vi "FIB MAIN.vi"() -> ()   [LabVIEW 2018]
uses:
  <vilib>/userdefined/High Color/IMAQdx.ctl
  STAGE POSITION.ctl
  Original FIB Source/CENTER STIGMATOR.ctl
  FIB EVENTS.ctl
  PI APERTURE POSITION.ctl
  APERTURE POSITION.ctl
  FIB CAMERA EVENTS.ctl
  <vilib>/vision/driver/IMAQdx.llb/IMAQdx Buffer Number Mode.ctl
  <vilib>/vision/driver/IMAQdx.llb/IMAQdx Camera Control Mode.ctl
  <vilib>/Instr/_visa.llb/VISA Flush IO Buffer Mask.ctl
  <vilib>/Utility/error.llb/whitespace.ctl
  Mikrodaq/HYMOD MAIA/ddd.ctl
  PI STAGE MAXIMUMS.ctl
  FIB STAGE EVENTS.ctl
  <vilib>/Instr/_visa.llb/VISA Configure Serial Port (Instr).vi
  <vilib>/vision/driver/NI_Vision_Acquisition_Software.lvlib
  <resource>/objmgr/imaqdx.rc
  <vilib>/vision/NI_Vision_Development_Module.lvlib
  <vilib>/Utility/Variable/NI_VariableUtilities.lvlib
panel:
  out "elements":T1[](array[typedef])
  out "PREVIOUS GUN SETTINGS":T2 {"ION CURRENT" min=0 max=3e-05 step=1e-07; "SUPPRESSOR" min=0 max=30000 step=250; "EXTRACTOR" min=0 max=30000 step=250; "BEAM ENERGY" min=0 max=30000 step=1000}
  out "size(s) 5":i32
  in  "ENABLE ORSAY":bool=TRUE
  in  "ENABLE CAMERA":bool
  out "size(s) 4":i32
  in  "Tab Control 4":enum32{"COMMANDS", "HV RAMPS"}(tab)
  in  "1V ENERGY RAMP":bool
  out "TEST OUTPUT":string
  in  "TEST COMMAND":bool
  in  "TEST COMMAND":string
  out "SERIAL \nRESPONSE":string[](array[string])
  out "WARNING":string
  out "PROCESS":string
  out "PROCESSES":string[](array[string])
  out "BEAM RAMP":dbl[unit][](graph)
  out "EXTRACTOR RAMP":dbl[unit][](graph)
  out "SUPPRESSOR RAMP":dbl[unit][](graph)
  in  "Tab Control 3":T3(tab)
  in  "E&B":T4 {"ELECTRIC FIELD" min=0 max=20 step=0.1 scale=0.0..2.0; "M-FINE" min=0 max=20000 step=100 scale=-0.08..0.08; "M-COARSE" min=0 max=20 step=0.1 scale=0.0..2.0}
  in  "WIEN":bool
  out "CURRENT":dbl[unit] format="%_4g"
  out "VOLTAGE":dbl[unit] format="%_4g"
  out "BEAM VOLTAGE":dbl[unit](graph)
  out "BEAM CURRENT":dbl[unit](graph)
  out "VOLTAGE":dbl[unit] format="%_4g"
  out "CURRENT":dbl[unit] format="%_4g"
  out "EXTRACTOR":dbl[unit](graph)
  out "EXTRACTOR  CURRENT":dbl[unit](graph)
  out "VOLTAGE":dbl[unit] format="%_4g"
  out "CURRENT":dbl[unit] format="%_4g"
  out "SUPPRESSOR VOLTAGE":dbl[unit](graph)
  out "SUPPRESSOR CURRENT":dbl[unit](graph)
  out "CONDENSOR VOLTAGE":dbl[unit](graph)
  out "CONDENSOR CURRENT":dbl[unit](graph)
  out "OBJECTIVE VOLTAGE":dbl[unit](graph)
  out "OBJECTIVE CURRENT":dbl[unit](graph)
  out "HV SUPPLY FEEDBACK 13":dbl[unit](graph)
  out "HV SUPPLY FEEDBACK 12":dbl[unit](graph)
  out "HEAT POWER":cluster{i32[], dbl[unit][]}(graph)
  in  "IGAIN":dbl=0.00039 format="%_3p"
  in  "IOFFSET":dbl format="%_4g"
  in  "VOFFSET":dbl format="%_4g"
  out "CURRENT":dbl[unit] format="%_4g"
  out "VOLTAGE":dbl[unit] format="%_4g"
  in  "VGAIN":dbl=0.00071 format="%_3p"
  in  "OFFSET":dbl
  in  "RPONT":dbl[unit]
  in  "RMES":dbl[unit]
  out "TIMER":u32
  out "size(s)":i32
  out "SUPPRESSOR RAMP":dbl[unit][](array[numeric])
  out "EXTRACTOR RAMP":dbl[unit][](array[numeric])
  out "BEAM RAMP":dbl[unit][](array[numeric])
  in  "MEASURE HV":bool
  out "SERIAL \nRESPONSE 2":string[](array[string])
  out "VISA ERROR":errorcluster
  out "BEAM CURRENT (FC2)":dbl[unit] format="%_4g"
  out "BEAM CURRENT (FC1)":dbl[unit] format="%_4g"
  in  "APERTURE (MASS)":u16(ring)=3 items=["10 um", "20 um", "50 um", "50 um", "100 um", "200 um", "400 um"]
  in  "BRIGHT,CONT,GAMMA":cluster{"B":dbl, "C":dbl, "G":dbl}={"B"=250.0, "C"=67.0, "G"=1.6000000000000005} {"G" format="%_4g"; "C" format="%_4g"; "B" format="%_4g"}
  in  "REFLECTIVITY":bool
  in  "ROTATE VIEW":bool
  in  "ANGLE":sgl format="%.2f"
  in  "IMAGE SYMMETRY":u32(ring)=2 items=["Horizontal", "Vertical", "CENTRAL", "1st Diagonal", "2nd Diagonal"]
  in  "SYMMETRY":bool
  out "FIB CAMERA ERROR":errorcluster
  out "FIB SAMPLE CAMERA":T5="CSIRO-SAMPLE" caption="Session Out"
  out "IMAGE YCENTRE":dbl
  out "IMAGE XCENTRE":dbl
  out "ActualPeakBandwidth":dbl=1000.0
  out "IMAGE YPIXELS":u32=1024
  out "IMAGE XPIXELS":u32=1360
  in  "START SCANNING":bool
  in  "STOP":bool
  out "INTERLOCK STATE":bool
  in  "BEAM ON":bool=TRUE
  in  "BLANKING CONTROL":u16(ring) items=["LOCAL ", "SOURCE", "EXTERNAL"]
  in  "FIB SETUP FILE":path=path "C:/Users/jamie/Desktop/test.tdms"
  in  "SAVE SETUP":bool
  in  "READ & APPLY SETUP":bool
  in  "OBJECT APERTURE":u16(ring)=3 items=["10 um", "20 um", "50 um", "50 um", "100 um", "200 um", "400 um"]
  in  "USER":string="jslaird"
  in  "COMMENT":string
  in  "NAME":string
  out "gamme":bool
  out "Image":T6(plugin-control)
  in  "Tab Control":T7(tab)
  in  "RESET":bool
  in  "INTERLOCK HV":bool
  out "HIGH ENERGY":bool
  in  "SETTINGS DELAY":dbl[unit]=0.2
  in  "dV ENERGY":dbl[unit]=250.0
  in  "dV SUPPRESS":dbl[unit]=50.0
  in  "SHUTDOWN":bool
  in  "FILAMENT":bool
  out "HIGH VOLTAGE SUPPLIES":cluster{dbl[unit], dbl[unit], dbl[unit]}(knob)={0.0, 103.78830891166923, 181.50345045415557} scale format="%#_6p"
  in  "ION GUN":bool
  in  "FILAMENT HEATING":dbl[unit](slide) min=0.0 max=5.0 step=0.1 scale=0.0..5.000000000000001
  in  "ION GUN SETTINGS":T2 {"ION CURRENT" min=0 max=3e-05 step=1e-07; "SUPPRESSOR" min=0 max=30000 step=250; "EXTRACTOR" min=0 max=30000 step=250; "BEAM ENERGY" min=0 max=30000 step=250}
  in  "dV EXTRACTOR":dbl[unit]=50.0
  in  "MOVE 2 POSITION":T8 {"Z" format="%_4g"; "Y" format="%_4g"; "X" format="%_4g"}
  out "POSITION":T8 {"Z" format="%_4g"; "Y" format="%_4g"; "X" format="%_4g"}
  in  "EXPOSURE":dbl(slide)=106.26827541712952 min=1.0 max=2500.0 step=10.0 scale=5.0..1000.0 scale format="%#_3f"
  out "FIB CAMERA":T6(plugin-control)
  out "IP ADDRESS":string="192.168.1.10"
  in  "CONFIGS":u16(ring) items=["MANUAL", "BEAM FOCUS", "SAMPLE VIEWING"]
  in  "GAIN METHOD":u16(ring)=2 items=["OFF", "ONCE", "CONTINOUS"]
  in  "GAIN":sgl=1.0 min=0 max=31 step=1
  out "CENTRE CAMERA FOV":T9={"Numeric Control"=677, "Numeric Control"=510}
  in  "Tab Control 2":T10(tab)
  in  "STORE OBJECT":bool
  in  "WOBBLER SETTINBGS FOR OBJECT ALIGNMENT":T11={"WOBBLER AMPLITUDE"={0.0, 33.333523, 47.735184}, "WOBBLE"=1} {"WOBBLE" items=["ENERGY", "CONDENSOR", "OBJECTIVE"]; "WOBBLER AMPLITUDE" scale=0.0..100.0}
  in  "OBJ APERTURE ALIGNMENT":T12={"DOWN"=FALSE, "UP"=FALSE, "STEP SIZE"=1, "LEFT"=FALSE, "RIGHT"=FALSE} {"STEP SIZE" items=["1 um", "5 um", "20 um", "50 um", "100 um", "250 um", "500 um", "1000 um"]}
  in  "TURN ON WOBBLER":bool
  out "OBJECT POSITION":T13 {"Yo" format="%.3f"; "Xo" min=0.0 max=12.5 step=0.1 format="%.3f"}
  in  "SET OBJECT":T13 {"Yo" min=0.0 max=10.0 step=0.1 format="%.3f"; "Xo" min=0.0 max=12.5 step=0.1 format="%.3f"}
  in  "OBJECT POSITIONS":T14(array[cluster])=[{"POSITION"={"Xm"=0.5, "Ym"=0.1114}}, {"POSITION"={"Xm"=0.0, "Ym"=0.0}}, {"POSITION"={"Xm"=11.3603, "Ym"=0.0}}, {"POSITION"={"Xm"=9.6127, "Ym"=0.0}}, {"POSITION"={"Xm"=7.8602, "Ym"=0.0}}, {"POSITION"={"Xm"=6.1203, "Ym"=0.0}}, {"POSITION"={"Xm"=4.37, "Ym"=0.0}}, {"POSITION"={"Xm"=0.0, "Ym"=0.0}}, {"POSITION"={"Xm"=0.0, "Ym"=0.0}}] {"POSITION"."Ym" format="%.3f"; "POSITION"."Xm" format="%.3f"}
  in  "MASS APERTURE ALIGNMENT":T12={"DOWN"=FALSE, "UP"=FALSE, "STEP SIZE"=1, "LEFT"=FALSE, "RIGHT"=FALSE} {"STEP SIZE" items=["1 um", "5 um", "20 um", "50 um", "100 um", "250 um", "500 um", "1000 um"]}
  in  "STORE APERTURE":bool
  out "APERTURE POSITION":cluster{"Xm":dbl, "Ym":dbl} {"Ym" format="%.3f"; "Xm" format="%.3f"}
  in  "SET APERTURE":T15 {"Ym" min=-0.5 max=0.5 step=0.01 format="%.3f"; "Xm" min=-25.0 max=25.0 step=0.1 format="%.3f"}
  in  "APERTURE POSITIONS":T14(array[cluster])=[{"POSITION"={"Xm"=0.0, "Ym"=0.0}}, {"POSITION"={"Xm"=0.0, "Ym"=0.0}}, {"POSITION"={"Xm"=0.0, "Ym"=0.0}}, {"POSITION"={"Xm"=0.0, "Ym"=0.0}}, {"POSITION"={"Xm"=1.0, "Ym"=0.0}}, {"POSITION"={"Xm"=0.0, "Ym"=0.0}}, {"POSITION"={"Xm"=0.0, "Ym"=0.0}}] {"POSITION"."Ym" format="%.3f"; "POSITION"."Xm" format="%.3f"}
  in  "STIGMATOR":T16 {"STIG ALIGN"."-Y" min=-100 max=100 step=0.1 scale=-100.0..100.0; "STIG ALIGN"."+Y" min=-100 max=100 step=0.1 scale=-100.0..100.0; "STIG ALIGN"."-X" min=-100 max=100 step=0.1 scale=-100.0..100.0; "STIG ALIGN"."+X" min=-100 max=100 step=0.1 scale=-100.0..100.0; "THETA" format="%_3g"; "OFFY" format="%_3g"; "OFFX" format="%_3g"; "STIG Y" format="%_3g"; "STIG X" format="%_3g"}
  in  "STIGMATOR X & Y":cluster{"X":sgl, "Y":sgl} {"Y" min=0 max=20000 step=100 scale=0.0..1000.0; "X" min=0 max=20 step=0.1 scale=0.0..20.0}
  out "OBJECTIVE":sgl[unit] format="%_4g"
  out "CONDENSOR":sgl[unit] format="%_4g"
  in  "OBJECTIVE":cluster{"COARSE":sgl[unit], "FINE":sgl[unit]} {"FINE" min=0 max=20000 step=100 scale=0.0..1000.0; "COARSE" min=0 max=20000 step=100}
  in  "CONDENSOR":cluster{"COARSE":sgl[unit], "FINE":sgl[unit]} {"FINE" min=0 max=20000 step=100 scale=1.0..1000.0; "COARSE" min=0 max=20000 step=100}
  in  "SCAN CENTRE ON STAGE":T17 {"Zs" format="%_2g"; "Xs" format="%_2g"; "Ys" format="%_2g"}
  in  "STAGE POSITION":T17 {"Zs" format="%_2g"; "Xs" format="%_2g"; "Ys" format="%_2g"}
  in  "SCANNING CLUSTER":T18 {"MAGNIFICATION" scale=-180.0..180.0; "Y-OFFSET" min=0 max=3e-05 step=1e-07; "X-OFFSET" min=0 max=3e-05 step=1e-07; "SCANNING TYPE" items=["EXTERNAL", "ION MILLING"]}
  in  "EXTERNAL SCANNING ROI":T19={"X-AMPLITUDE"=1e-07, "dX"=0.0, "Y-AMPLITUDE"=1e-07, "dY"=0.0} {"Y-AMPLITUDE" min=1e-07 max=0.0005 step=9.999999999999999e-06; "X-AMPLITUDE" min=1e-07 max=0.0005 step=9.999999999999999e-06}
  out "CHAMBER VACUUM":cluster{dbl[unit], dbl[unit]}(knob)={2.179544466940017e-05, 0.00030039245125477424} scale format="%#_2e"
  in  "COLUMN THRESHOLD":dbl[unit]=6.666118421052631e-05
  out "VACUUM STATE":bool
  out "COLUMN VACUUM":dbl[unit](graph)
  out "COLUMN VACUUM":cluster{dbl[unit], dbl[unit]}(knob)={8.118323356328827e-09, 0.00010317996118558537} scale format="%#_1e"
  out "150V GOOD":bool
  in  "CHAMBER THRESHOLD":dbl[unit]
  in  "GATE VALVE":bool=TRUE
  in  "TERMINATION":bool=TRUE
  in  "TERMINATION CHAR":u16(ring)=1 items=["NONE", "CR", "LF", "CR+LF"]
  out "APPEND":string
  out "ORSAY CONNECTED":bool
  in  "STARTUP":T1[](array[typedef])=[enum."OPEN SERIAL CONN TO ORSAY", enum."INITIALISE ORSAY", enum."TURN OFF WOBBLER", enum."VACUUM ", enum."CHECK 150V", enum."BLANKING TOGGLE"]
  out "ORSAY":refnum<visa-resource-name>
  # "EXTRACTOR"
  # "CONDENSOR"
  # "OBJECT\nAPERTURES"
  # "OBJECTIVE"
  # "FILAMENT SHOULD BE ON PRIOR TO GUN !"
  # "E"
  # "C"
  # "O"
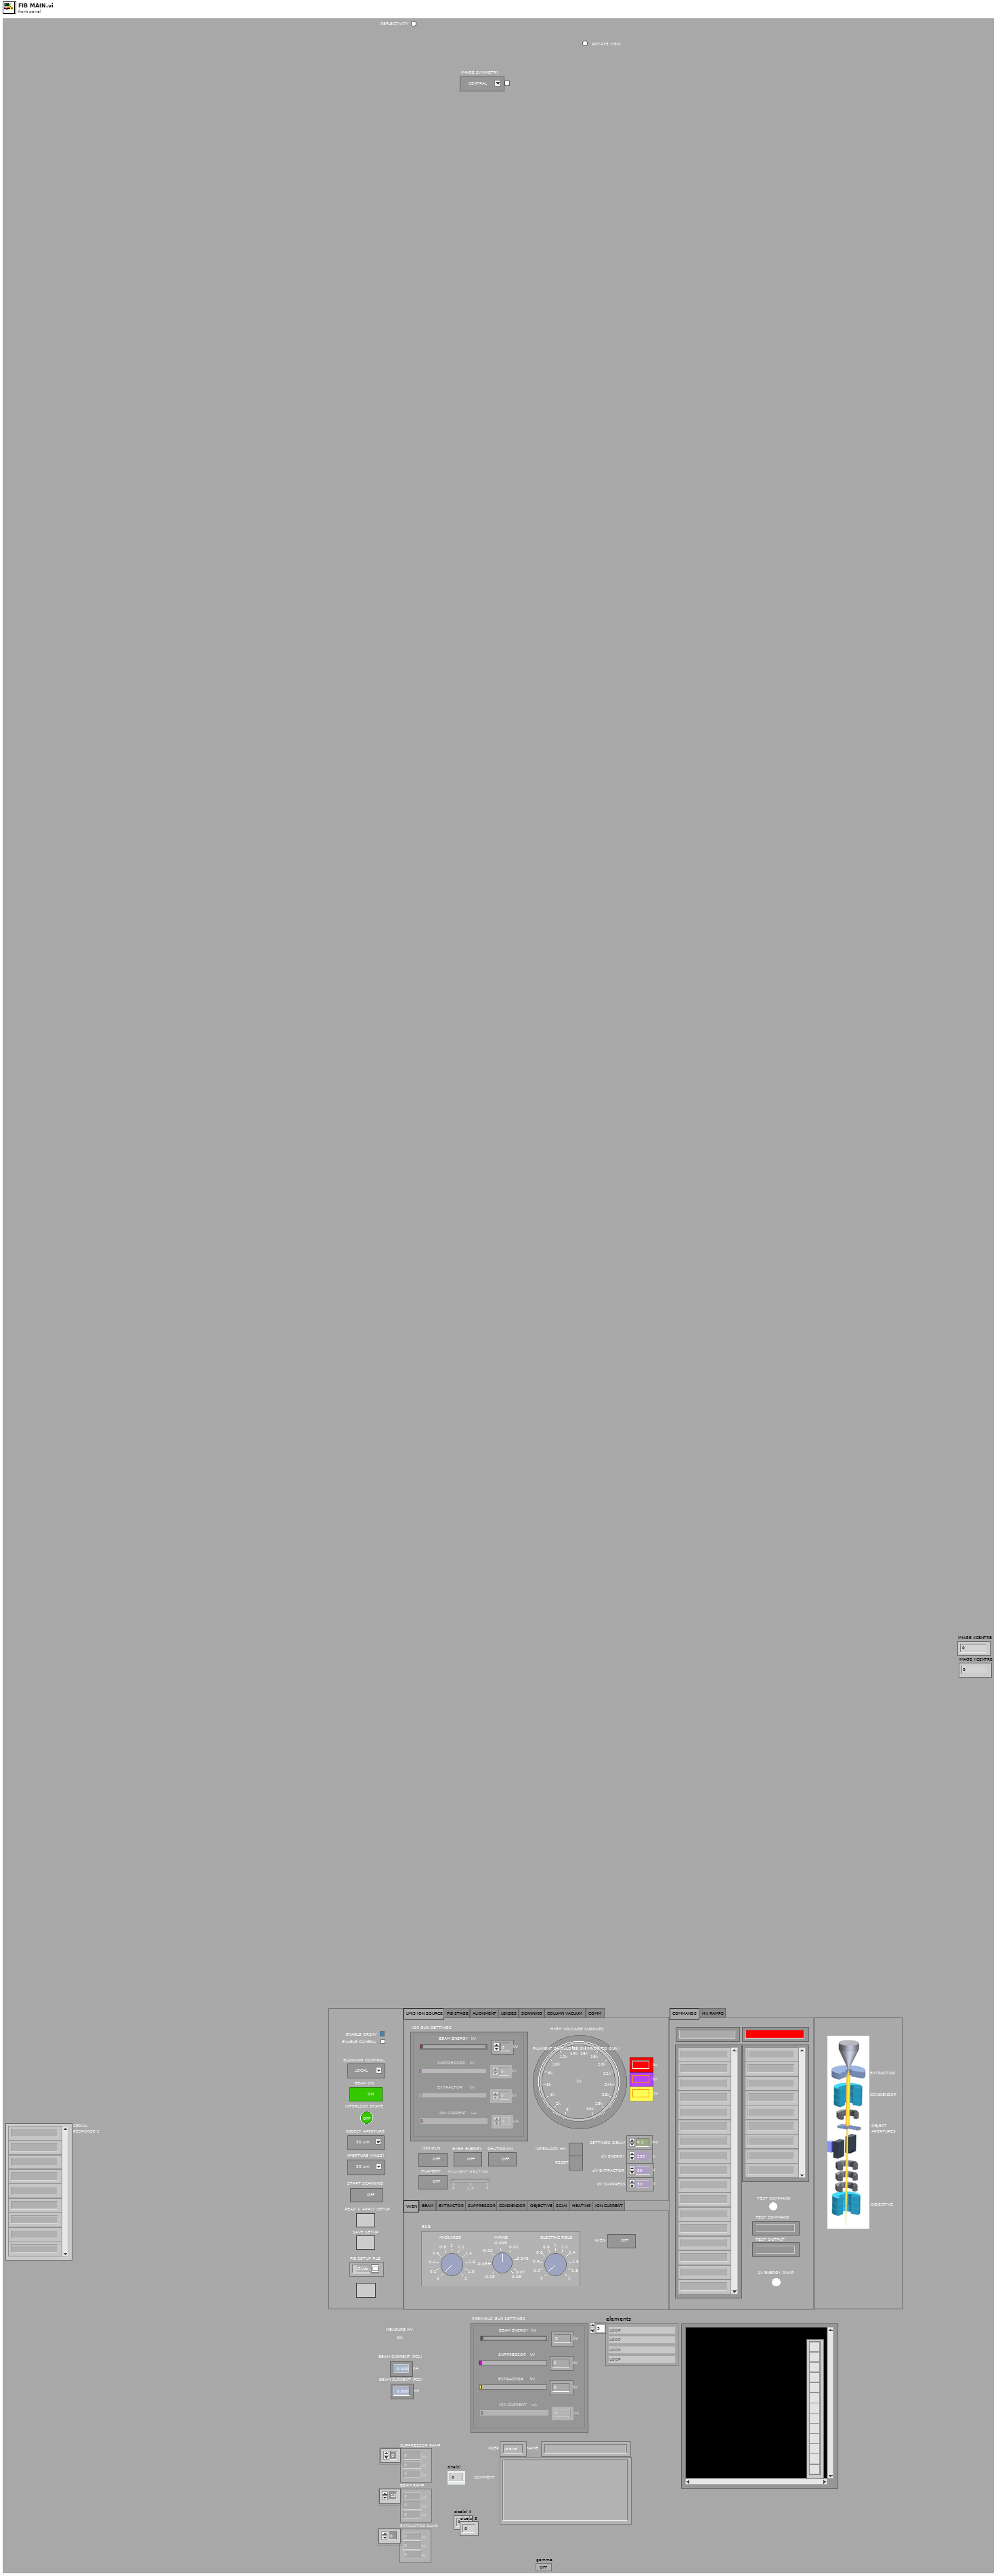
[diagram p1: front panel]
types:
  T1 = typedef "FIB EVENTS.ctl" = enum16{"LOOP", "OPEN SERIAL CONN TO ORSAY", "INITIALISE ORSAY", "READ SETTINGS", "SAVE SETTINGS", "OBJECTIVE LENS", "CONDENSOR LENS", "BLANKING TOGGLE", "TURN ON HEATER", "TURN OFF WOBBLER", "MEASURE HEATER OUTPUT", "TOGGLE GATE VALVE", "SCANNING CONTROLS", "TURN ON BEAM HV", "ENERGY RAMP CYCLE", "TURN ON SUPPRESSOR", "TURN ON EXTRACTOR", "TURN ON WIEN FILTER", "SET ENERGY RANGE", "MEASURE HV SUPPLY VOLTAGES", "SHUTDOWN ION SOURCE", "RESET TYPE II", "PROBE CURRENT FC#1", "PROBE CURRENT FC#2", "VACUUM ", "CHECK 150V", "INITIALISE PI MOTORS", "SET STIGMATOR", "SET WOBBLER FOR OBJECT", "SHIFT OBJECT APERTURE", "STORE OBJECT POSITION", "STORE APERTURE POSITION", "SHIFT MASS APERTURE", "DEFINE NEW APERTURE", "MOVE TO OBJECT", "MOVE TO APERTURE", "STOP SYSTEM", "TEST COMMANDS"}
  T2 = cluster{"BEAM ENERGY":sgl[unit], "SUPPRESSOR":sgl[unit], "EXTRACTOR":sgl[unit], "ION CURRENT":sgl[unit]}
  T3 = enum32{"WIEN", "BEAM", "EXTRACTOR", "SUPPRESSOR", "CONDENSOR", "OBJECTIVE", "SCAN", "HEATING", "ION CURRENT"}
  T4 = cluster{"M-COARSE":sgl, "M-FINE":sgl, "ELECTRIC FIELD":sgl}
  T5 = typedef "IMAQdx.ctl" = refnum<k21>
  T6 = typedef "IMAQ Image.ctl" = refnum<image>
  T7 = enum32{"LMIS ION SOURCE", "FIB STAGE", "ALIGNMENT", "LENSES", "SCANNING", "COLUMN VACUUM", "COMM"}
  T8 = typedef "STAGE POSITION.ctl" = cluster{"X":dbl[unit], "Y":dbl[unit], "Z":dbl[unit]}
  T9 = cluster{"Numeric Control":i32, "Numeric Control":i32}
  T10 = enum32{"OBJECTS", " APERTURES", "CENTRE STIGMATOR"}
  T11 = cluster{"WOBBLER AMPLITUDE":cluster{sgl, sgl, sgl}, "WOBBLE":u16}
  T12 = cluster{"DOWN":bool, "UP":bool, "STEP SIZE":u16, "LEFT":bool, "RIGHT":bool}
  T13 = typedef "PI APERTURE POSITION.ctl" = cluster{"Xo":dbl, "Yo":dbl}
  T14 = cluster{"POSITION":cluster{"Xm":dbl, "Ym":dbl}}[]
  T15 = typedef "APERTURE POSITION.ctl" = cluster{"Xm":dbl, "Ym":dbl}
  T16 = typedef "CENTER STIGMATOR.ctl" = cluster{"STIG ALIGN":cluster{"+X":sgl, "-X":sgl, "+Y":sgl, "-Y":sgl}, "STIG X":dbl, "OFFX":dbl, "STIG Y":dbl, "OFFY":dbl, "THETA":dbl}
  T17 = cluster{"Xs":dbl[unit], "Ys":dbl[unit], "Zs":dbl[unit]}
  T18 = cluster{"SCANNING TYPE":u16, "X-OFFSET":sgl[unit], "Y-OFFSET":sgl[unit], "ROTATION":dbl[unit], "MAGNIFICATION":dbl}
  T19 = cluster{"X-AMPLITUDE":dbl[unit], "dX":dbl[unit], "Y-AMPLITUDE":dbl[unit], "dY":dbl[unit]}
  T20 = typedef "FIB CAMERA EVENTS.ctl" = enum16{"INIT VIDEO", "CAMERA GAIN", "CAMERA EXPOSURE", "LOOP"}
  T21 = enum8{"Enabled", "Disabled", "Disabled and Grayed Out"}
  T22 = cluster{"BEAM ENERGY":sgl[unit], "EXTRACTOR":sgl[unit], "SUPPRESSOR":sgl[unit], "ION CURRENT":sgl[unit]}
  T23 = typedef "FIB STAGE EVENTS.ctl" = enum16{"LOOP", "INIT STAGE CONTROLLER", "SEND COMMAND TO CONTROLLER", "HOME X", "HOME Y", "HOME Z", "ABORT ALL AXES", "GOTO MARKER", "ZERO XYZ", "READ XYZ POSITIONS", "GOTO XYZ POSITION", "STOP", "JOG XYZ", "WAIT FOR MOVE COMPLETE"}
  T24 = cluster{"BEAM":dbl[unit], "SUPPRESSOR":dbl[unit], "EXTRACTOR":dbl[unit]}
  T25 = typedef "ddd.ctl" = string[]
  T26 = enum16{"open", "open or create", "create or replace", "create", "open (read-only)"}
  T27 = typedef "VISA Flush IO Buffer Mask.ctl" = u16
  T28 = cluster{dbl[unit], "CHAMBER THRESHOLD":dbl[unit]}
  T29 = typedef "whitespace.ctl" = u16
  T30 = typedef "PI STAGE MAXIMUMS.ctl" = cluster{"Xo MAX":dbl, "Xm MAX":dbl, "Yo MAX":dbl, "Ym MAX":dbl}
  T31 = cluster{"Xo MIN":dbl, "Xm MIN":dbl, "Yo MIN":dbl, "Ym MIN":dbl}
  T32 = typedef "NI_Vision_Acquisition_Software.lvlib/IMAQdx Buffer Number Mode.ctl" = enum32{"Next", "Last", "Buffer Number", "Every", "Last New"}
  T33 = typedef "NI_Vision_Acquisition_Software.lvlib/IMAQdx Camera Control Mode.ctl" = enum32{"Controller", "Listener"}
  T34 = typedef "Image Type" = u32
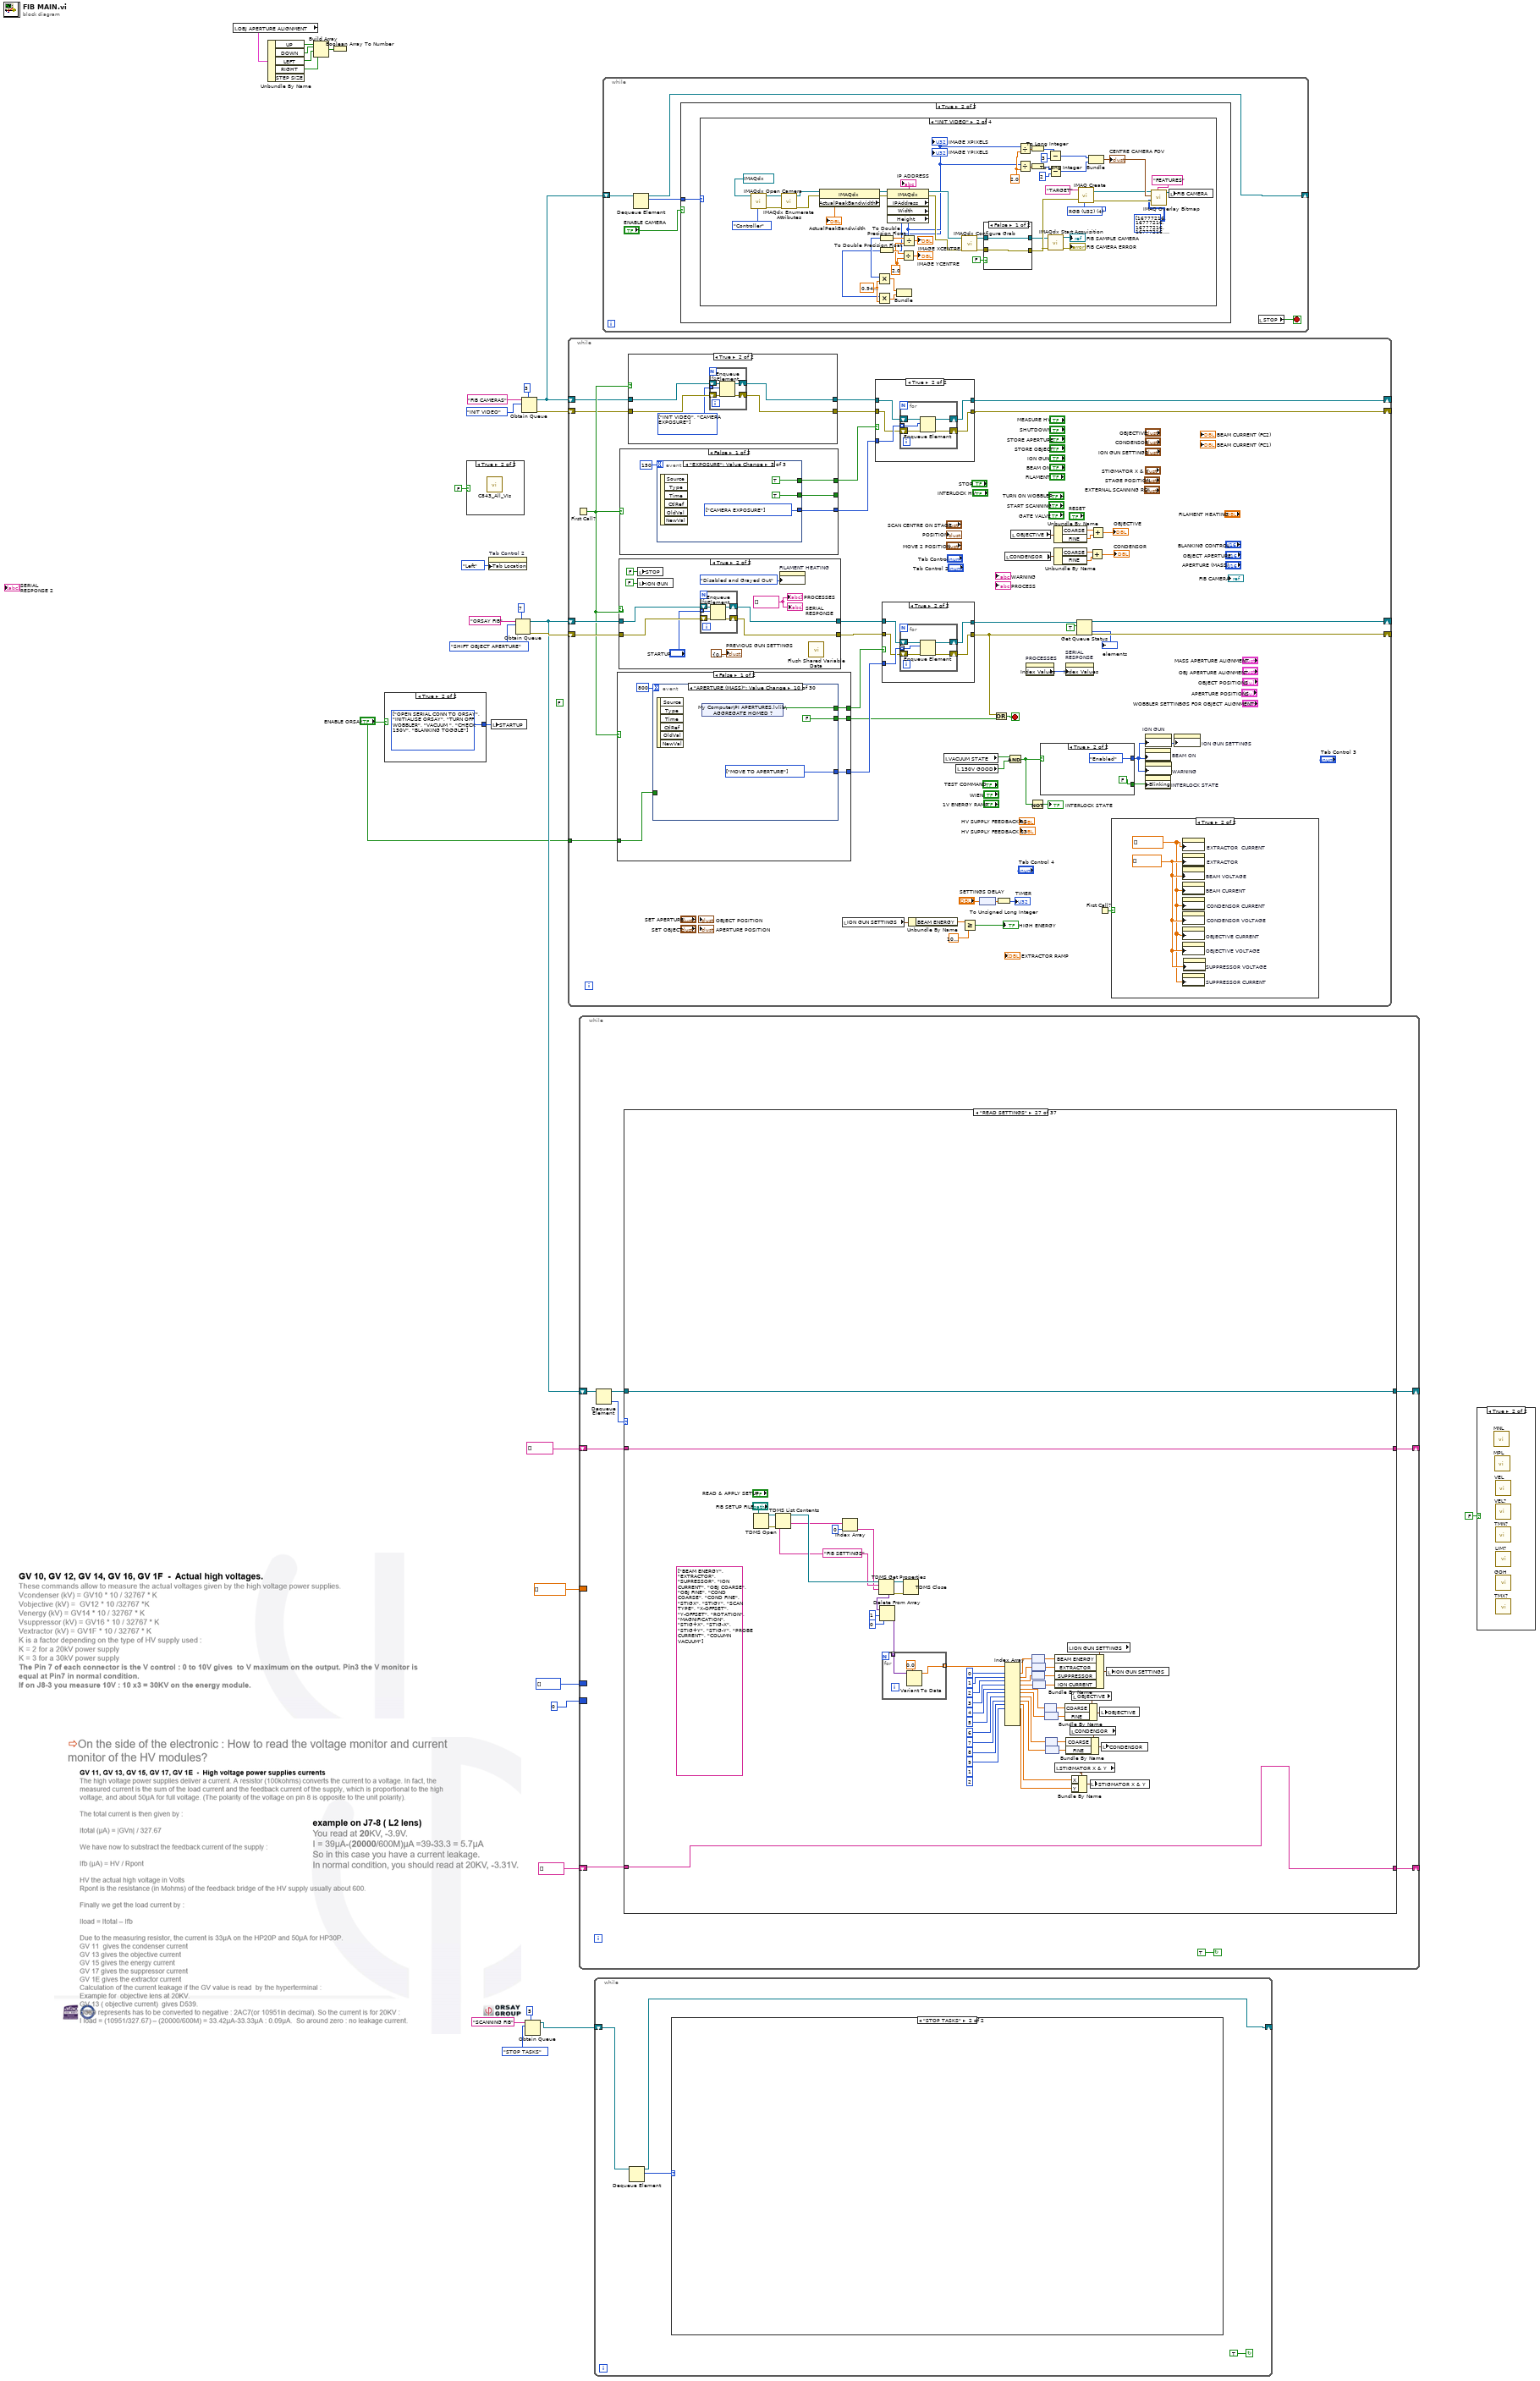
[diagram p0: block diagram]
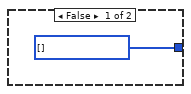
[diagram p2: hidden frame]
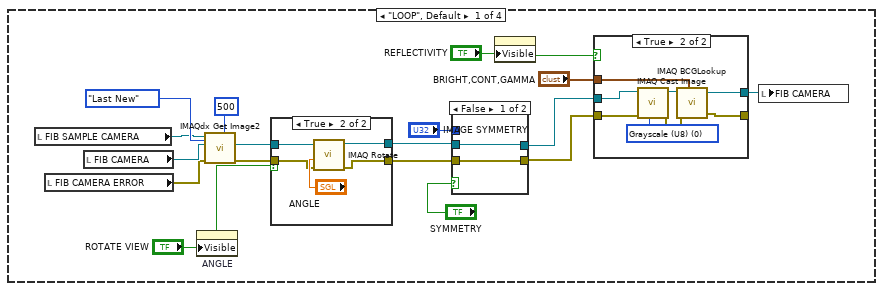
[diagram p7: hidden frame]
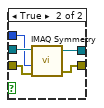
[diagram p10: hidden frame]
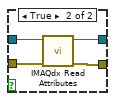
[diagram p11: hidden frame]
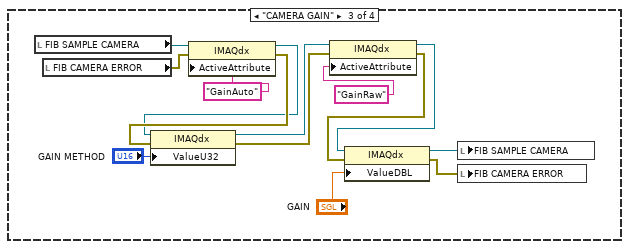
[diagram p12: hidden frame]
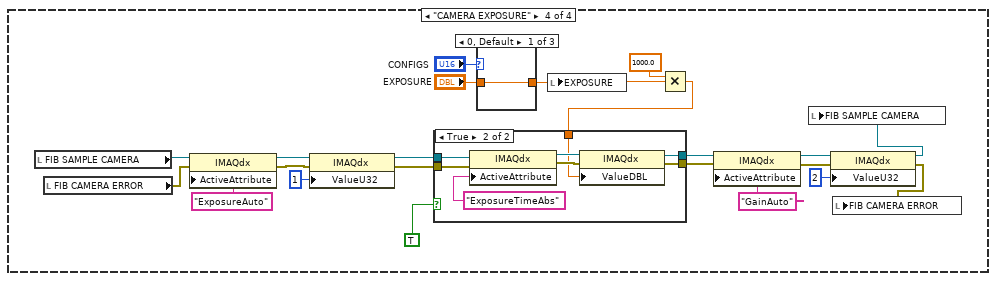
[diagram p13: hidden frame]
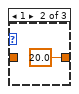
[diagram p15: hidden frame]
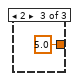
[diagram p16: hidden frame]
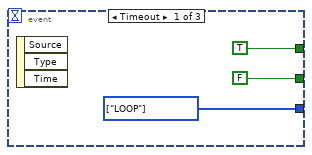
[diagram p19: hidden frame]
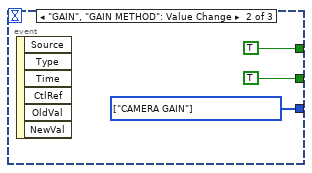
[diagram p20: hidden frame]
diagram:
  (unwired) FALSE ("ION GUN")
  n1 = local read "OBJ APERTURE ALIGNMENT"() -> (w17:T12)
  n2 = Unbundle By Name(w17) -> ("UP"=w18:bool, "DOWN"=w19:bool, "LEFT"=w20:bool, "RIGHT"=w21:bool)  [unwired: 1 out]
  n3 = Build Array(w18, w19, w20, w21) -> (w22:bool[])
  n4 = Boolean Array To Number(Boolean array=w22) -> ()  [unwired: 1 out]
  n5 = case shown="True" "ENABLE ORSAY" {
    tunnel: [w31 w32] -> w1
    frame False {
      w31 = T1[] [] items=["LOOP", "OPEN SERIAL CONN TO ORSAY", "INITIALISE ORSAY", "READ SETTINGS", "SAVE SETTINGS", "OBJECTIVE LENS", "CONDENSOR LENS", "BLANKING TOGGLE", "TURN ON HEATER", "TURN OFF WOBBLER", "MEASURE HEATER OUTPUT", "TOGGLE GATE VALVE", "SCANNING CONTROLS", "TURN ON BEAM HV", "ENERGY RAMP CYCLE", "TURN ON SUPPRESSOR", "TURN ON EXTRACTOR", "TURN ON WIEN FILTER", "SET ENERGY RANGE", "MEASURE HV SUPPLY VOLTAGES", "SHUTDOWN ION SOURCE", "RESET TYPE II", "PROBE CURRENT FC#1", "PROBE CURRENT FC#2", "VACUUM ", "CHECK 150V", "INITIALISE PI MOTORS", "SET STIGMATOR", "SET WOBBLER FOR OBJECT", "SHIFT OBJECT APERTURE", "STORE OBJECT POSITION", "STORE APERTURE POSITION", "SHIFT MASS APERTURE", "DEFINE NEW APERTURE", "MOVE TO OBJECT", "MOVE TO APERTURE", "STOP SYSTEM", "TEST COMMANDS"] ("STARTUP")
    }
    frame True {
      w32 = T1[] [enum."OPEN SERIAL CONN TO ORSAY", enum."INITIALISE ORSAY", enum."TURN OFF WOBBLER", enum."VACUUM ", enum."CHECK 150V", enum."BLANKING TOGGLE"] items=["LOOP", "OPEN SERIAL CONN TO ORSAY", "INITIALISE ORSAY", "READ SETTINGS", "SAVE SETTINGS", "OBJECTIVE LENS", "CONDENSOR LENS", "BLANKING TOGGLE", "TURN ON HEATER", "TURN OFF WOBBLER", "MEASURE HEATER OUTPUT", "TOGGLE GATE VALVE", "SCANNING CONTROLS", "TURN ON BEAM HV", "ENERGY RAMP CYCLE", "TURN ON SUPPRESSOR", "TURN ON EXTRACTOR", "TURN ON WIEN FILTER", "SET ENERGY RANGE", "MEASURE HV SUPPLY VOLTAGES", "SHUTDOWN ION SOURCE", "RESET TYPE II", "PROBE CURRENT FC#1", "PROBE CURRENT FC#2", "VACUUM ", "CHECK 150V", "INITIALISE PI MOTORS", "SET STIGMATOR", "SET WOBBLER FOR OBJECT", "SHIFT OBJECT APERTURE", "STORE OBJECT POSITION", "STORE APERTURE POSITION", "SHIFT MASS APERTURE", "DEFINE NEW APERTURE", "MOVE TO OBJECT", "MOVE TO APERTURE", "STOP SYSTEM", "TEST COMMANDS"] ("STARTUP")
    }
  }
  n6 = case shown="True" FALSE {
    frame False {
    }
    frame True {
      n7 = call "C843_All_VIs.vi"() -> ()  [unwired: 1 in]
    }
  }
  n8 = property on="Tab Control 2" class="TabCtl (strict)"("Tab Location"=enum32{"Top", "Bottom", "Left", "Right"}."Left") -> ()  [unwired: 2 in, 2 out]
  n9 = local write "STARTUP"(w1) -> ()
  n10 = Obtain Queue(max queue size (-1, unlimited)=7, name (unnamed)="ORSAY FIB", element data type=FIB_EVENTS."SHIFT OBJECT APERTURE" ("Enum")) -> (queue out=w7:refnum<queue>, error out=w28:errorcluster)  [unwired: 2 in, 1 out]
  n11 = Obtain Queue(max queue size (-1, unlimited)=3, name (unnamed)="FIB CAMERAS", element data type=FIB_CAMERA_EVENTS."INIT VIDEO") -> (queue out=w23:refnum<queue>, error out=w24:errorcluster)  [unwired: 2 in, 1 out]
  n12 = Obtain Queue(max queue size (-1, unlimited)=5, name (unnamed)="SCANNING FIB", element data type=enum16{"INIT DAQ", "STOP TASKS"}."STOP TASKS") -> (queue out=w11:refnum<queue>)  [unwired: 2 in, 2 out]
  n13 = while {
    shift-right: [w71] -> _
    shift-left: w7 -> [w79]
    shift-right: [w68] -> _
    shift-left: w28 -> [w78]
    shift-right: [w57] -> _
    shift-left: w23 -> [w63]
    shift-right: [w56] -> _
    shift-left: w24 -> [w62]
    tunnel: "ENABLE ORSAY" -> [w34]
    stop <- w40 stop-if-true
    n14 = First Call?() -> (First Call?: T/F=w64:bool)
    n15 = case shown="False" w64 {
      tunnel: [w129 FALSE] -> w76
      tunnel: [w128 w244] -> w75
      tunnel: [w127 FALSE] -> w72
      tunnel: w34 -> [w126 _]
      frame False {
        n16 = event shown="[9] \"APERTURE (MASS)\": Value Change" {
          selector: _ -> [_ _ _ _ _ _ _ _ _ _ _ _ _ _ _ _ _ _ _ _ _ _ _ _ _ _ _ _ _ _]
          dyn-events: _ -> [_ _ _ _ _ _ _ _ _ _ _ _ _ _ _ _ _ _ _ _ _ _ _ _ _ _ _ _ _ _]
          timeout: 800 -> [_ _ _ _ _ _ _ _ _ _ _ _ _ _ _ _ _ _ _ _ _ _ _ _ _ _ _ _ _ _]
          tunnel: [TRUE TRUE ("VACUUM STATE") TRUE ("VACUUM STATE") TRUE ("VACUUM STATE") w148 w150 w157 w162 w165 w168 w171 w175 w179 w182 w189 TRUE ("VACUUM STATE") TRUE ("VACUUM STATE") TRUE ("VACUUM STATE") w203 w205 w211 _ TRUE ("VACUUM STATE") w217 w221 w225 w229 TRUE w235 w239] -> w129
          tunnel: [FALSE FALSE FALSE FALSE FALSE FALSE FALSE FALSE FALSE FALSE FALSE FALSE FALSE FALSE FALSE FALSE FALSE FALSE FALSE FALSE FALSE _ FALSE FALSE FALSE FALSE FALSE FALSE FALSE FALSE] -> w127
          tunnel: [w131 w139 w140 w145 w146 w154 w160 w163 w167 w169 w172 w176 w178 w185 w187 w192 w195 w198 w201 w208 w209 w213 w214 w220 w224 w228 w231 w234 w236 w238] -> w128
          tunnel: w126 -> [w132 _ _ _ _ _ _ _ _ _ _ _ _ _ _ _ _ _ _ _ _ _ _ _ _ _ _ _ _ _]
          event Timeout {
            n17 = event-data() -> ()  [unwired: 1 in, 3 out]
            n18 = case shown="True" w132 {
              tunnel: [w135 w136] -> w131
              frame False {
                w135 = T1[] [] items=["LOOP", "OPEN SERIAL CONN TO ORSAY", "INITIALISE ORSAY", "READ SETTINGS", "SAVE SETTINGS", "OBJECTIVE LENS", "CONDENSOR LENS", "BLANKING TOGGLE", "TURN ON HEATER", "TURN OFF WOBBLER", "MEASURE HEATER OUTPUT", "TOGGLE GATE VALVE", "SCANNING CONTROLS", "TURN ON BEAM HV", "ENERGY RAMP CYCLE", "TURN ON SUPPRESSOR", "TURN ON EXTRACTOR", "TURN ON WIEN FILTER", "SET ENERGY RANGE", "MEASURE HV SUPPLY VOLTAGES", "SHUTDOWN ION SOURCE", "RESET TYPE II", "PROBE CURRENT FC#1", "PROBE CURRENT FC#2", "VACUUM ", "CHECK 150V", "INITIALISE PI MOTORS", "SET STIGMATOR", "SET WOBBLER FOR OBJECT", "SHIFT OBJECT APERTURE", "STORE OBJECT POSITION", "STORE APERTURE POSITION", "SHIFT MASS APERTURE", "DEFINE NEW APERTURE", "MOVE TO OBJECT", "MOVE TO APERTURE", "STOP SYSTEM", "TEST COMMANDS"]
              }
              frame True {
                w136 = T1[] [enum."MEASURE HV SUPPLY VOLTAGES", enum."MEASURE HEATER OUTPUT", enum."CHECK 150V", enum."LOOP"] items=["LOOP", "OPEN SERIAL CONN TO ORSAY", "INITIALISE ORSAY", "READ SETTINGS", "SAVE SETTINGS", "OBJECTIVE LENS", "CONDENSOR LENS", "BLANKING TOGGLE", "TURN ON HEATER", "TURN OFF WOBBLER", "MEASURE HEATER OUTPUT", "TOGGLE GATE VALVE", "SCANNING CONTROLS", "TURN ON BEAM HV", "ENERGY RAMP CYCLE", "TURN ON SUPPRESSOR", "TURN ON EXTRACTOR", "TURN ON WIEN FILTER", "SET ENERGY RANGE", "MEASURE HV SUPPLY VOLTAGES", "SHUTDOWN ION SOURCE", "RESET TYPE II", "PROBE CURRENT FC#1", "PROBE CURRENT FC#2", "VACUUM ", "CHECK 150V", "INITIALISE PI MOTORS", "SET STIGMATOR", "SET WOBBLER FOR OBJECT", "SHIFT OBJECT APERTURE", "STORE OBJECT POSITION", "STORE APERTURE POSITION", "SHIFT MASS APERTURE", "DEFINE NEW APERTURE", "MOVE TO OBJECT", "MOVE TO APERTURE", "STOP SYSTEM", "TEST COMMANDS"]
              }
            }
          }
          event "1V ENERGY RAMP": Mouse Down {
            w139 = T1[] [enum."ENERGY RAMP CYCLE"] items=["LOOP", "OPEN SERIAL CONN TO ORSAY", "INITIALISE ORSAY", "READ SETTINGS", "SAVE SETTINGS", "OBJECTIVE LENS", "CONDENSOR LENS", "BLANKING TOGGLE", "TURN ON HEATER", "TURN OFF WOBBLER", "MEASURE HEATER OUTPUT", "TOGGLE GATE VALVE", "SCANNING CONTROLS", "TURN ON BEAM HV", "ENERGY RAMP CYCLE", "TURN ON SUPPRESSOR", "TURN ON EXTRACTOR", "TURN ON WIEN FILTER", "SET ENERGY RANGE", "MEASURE HV SUPPLY VOLTAGES", "SHUTDOWN ION SOURCE", "RESET TYPE II", "PROBE CURRENT FC#1", "PROBE CURRENT FC#2", "VACUUM ", "CHECK 150V", "INITIALISE PI MOTORS", "SET STIGMATOR", "SET WOBBLER FOR OBJECT", "SHIFT OBJECT APERTURE", "STORE OBJECT POSITION", "STORE APERTURE POSITION", "SHIFT MASS APERTURE", "DEFINE NEW APERTURE", "MOVE TO OBJECT", "MOVE TO APERTURE", "STOP SYSTEM", "TEST COMMANDS"]
            n19 = event-data() -> ()  [unwired: 1 in, 8 out]
          }
          event "RESET": Mouse Down {
            w140 = T1[] [enum."INITIALISE ORSAY"] items=["LOOP", "OPEN SERIAL CONN TO ORSAY", "INITIALISE ORSAY", "READ SETTINGS", "SAVE SETTINGS", "OBJECTIVE LENS", "CONDENSOR LENS", "BLANKING TOGGLE", "TURN ON HEATER", "TURN OFF WOBBLER", "MEASURE HEATER OUTPUT", "TOGGLE GATE VALVE", "SCANNING CONTROLS", "TURN ON BEAM HV", "ENERGY RAMP CYCLE", "TURN ON SUPPRESSOR", "TURN ON EXTRACTOR", "TURN ON WIEN FILTER", "SET ENERGY RANGE", "MEASURE HV SUPPLY VOLTAGES", "SHUTDOWN ION SOURCE", "RESET TYPE II", "PROBE CURRENT FC#1", "PROBE CURRENT FC#2", "VACUUM ", "CHECK 150V", "INITIALISE PI MOTORS", "SET STIGMATOR", "SET WOBBLER FOR OBJECT", "SHIFT OBJECT APERTURE", "STORE OBJECT POSITION", "STORE APERTURE POSITION", "SHIFT MASS APERTURE", "DEFINE NEW APERTURE", "MOVE TO OBJECT", "MOVE TO APERTURE", "STOP SYSTEM", "TEST COMMANDS"]
            n20 = event-data() -> ()  [unwired: 1 in, 8 out]
          }
          event "MEASURE HV": Mouse Down {
            w145 = T1[] [enum."MEASURE HV SUPPLY VOLTAGES"] items=["LOOP", "OPEN SERIAL CONN TO ORSAY", "INITIALISE ORSAY", "READ SETTINGS", "SAVE SETTINGS", "OBJECTIVE LENS", "CONDENSOR LENS", "BLANKING TOGGLE", "TURN ON HEATER", "TURN OFF WOBBLER", "MEASURE HEATER OUTPUT", "TOGGLE GATE VALVE", "SCANNING CONTROLS", "TURN ON BEAM HV", "ENERGY RAMP CYCLE", "TURN ON SUPPRESSOR", "TURN ON EXTRACTOR", "TURN ON WIEN FILTER", "SET ENERGY RANGE", "MEASURE HV SUPPLY VOLTAGES", "SHUTDOWN ION SOURCE", "RESET TYPE II", "PROBE CURRENT FC#1", "PROBE CURRENT FC#2", "VACUUM ", "CHECK 150V", "INITIALISE PI MOTORS", "SET STIGMATOR", "SET WOBBLER FOR OBJECT", "SHIFT OBJECT APERTURE", "STORE OBJECT POSITION", "STORE APERTURE POSITION", "SHIFT MASS APERTURE", "DEFINE NEW APERTURE", "MOVE TO OBJECT", "MOVE TO APERTURE", "STOP SYSTEM", "TEST COMMANDS"]
            n21 = event-data() -> ()  [unwired: 1 in, 8 out]
          }
          event "GATE VALVE": Mouse Down {
            w146 = T1[] [enum."TOGGLE GATE VALVE"] items=["LOOP", "OPEN SERIAL CONN TO ORSAY", "INITIALISE ORSAY", "READ SETTINGS", "SAVE SETTINGS", "OBJECTIVE LENS", "CONDENSOR LENS", "BLANKING TOGGLE", "TURN ON HEATER", "TURN OFF WOBBLER", "MEASURE HEATER OUTPUT", "TOGGLE GATE VALVE", "SCANNING CONTROLS", "TURN ON BEAM HV", "ENERGY RAMP CYCLE", "TURN ON SUPPRESSOR", "TURN ON EXTRACTOR", "TURN ON WIEN FILTER", "SET ENERGY RANGE", "MEASURE HV SUPPLY VOLTAGES", "SHUTDOWN ION SOURCE", "RESET TYPE II", "PROBE CURRENT FC#1", "PROBE CURRENT FC#2", "VACUUM ", "CHECK 150V", "INITIALISE PI MOTORS", "SET STIGMATOR", "SET WOBBLER FOR OBJECT", "SHIFT OBJECT APERTURE", "STORE OBJECT POSITION", "STORE APERTURE POSITION", "SHIFT MASS APERTURE", "DEFINE NEW APERTURE", "MOVE TO OBJECT", "MOVE TO APERTURE", "STOP SYSTEM", "TEST COMMANDS"]
            n22 = event-data() -> ()  [unwired: 1 in, 8 out]
            n23 = local read "INTERLOCK STATE"() -> (w149:bool)
            n24 = Not(x=w149) -> (.not. x?=w148:bool)
          }
          event "ION GUN": Value Change {
            w154 = T1[] [enum."SET ENERGY RANGE", enum."TURN ON BEAM HV", enum."TURN ON SUPPRESSOR", enum."TURN ON EXTRACTOR"] items=["LOOP", "OPEN SERIAL CONN TO ORSAY", "INITIALISE ORSAY", "READ SETTINGS", "SAVE SETTINGS", "OBJECTIVE LENS", "CONDENSOR LENS", "BLANKING TOGGLE", "TURN ON HEATER", "TURN OFF WOBBLER", "MEASURE HEATER OUTPUT", "TOGGLE GATE VALVE", "SCANNING CONTROLS", "TURN ON BEAM HV", "ENERGY RAMP CYCLE", "TURN ON SUPPRESSOR", "TURN ON EXTRACTOR", "TURN ON WIEN FILTER", "SET ENERGY RANGE", "MEASURE HV SUPPLY VOLTAGES", "SHUTDOWN ION SOURCE", "RESET TYPE II", "PROBE CURRENT FC#1", "PROBE CURRENT FC#2", "VACUUM ", "CHECK 150V", "INITIALISE PI MOTORS", "SET STIGMATOR", "SET WOBBLER FOR OBJECT", "SHIFT OBJECT APERTURE", "STORE OBJECT POSITION", "STORE APERTURE POSITION", "SHIFT MASS APERTURE", "DEFINE NEW APERTURE", "MOVE TO OBJECT", "MOVE TO APERTURE", "STOP SYSTEM", "TEST COMMANDS"]
            n25 = event-data() -> ()  [unwired: 1 in, 6 out]
            n26 = local read "INTERLOCK STATE"() -> (w153:bool)
            n27 = local read "ION GUN"() -> (w151:bool)
            n28 = Not(x=w153) -> (.not. x?=w152:bool)
            n29 = And(x=w152, y=w151) -> (x .and. y?=w150:bool)
          }
          event "ION GUN SETTINGS.SUPPRESSOR": Value Change {
            w160 = T1[] [enum."TURN ON SUPPRESSOR"] items=["LOOP", "OPEN SERIAL CONN TO ORSAY", "INITIALISE ORSAY", "READ SETTINGS", "SAVE SETTINGS", "OBJECTIVE LENS", "CONDENSOR LENS", "BLANKING TOGGLE", "TURN ON HEATER", "TURN OFF WOBBLER", "MEASURE HEATER OUTPUT", "TOGGLE GATE VALVE", "SCANNING CONTROLS", "TURN ON BEAM HV", "ENERGY RAMP CYCLE", "TURN ON SUPPRESSOR", "TURN ON EXTRACTOR", "TURN ON WIEN FILTER", "SET ENERGY RANGE", "MEASURE HV SUPPLY VOLTAGES", "SHUTDOWN ION SOURCE", "RESET TYPE II", "PROBE CURRENT FC#1", "PROBE CURRENT FC#2", "VACUUM ", "CHECK 150V", "INITIALISE PI MOTORS", "SET STIGMATOR", "SET WOBBLER FOR OBJECT", "SHIFT OBJECT APERTURE", "STORE OBJECT POSITION", "STORE APERTURE POSITION", "SHIFT MASS APERTURE", "DEFINE NEW APERTURE", "MOVE TO OBJECT", "MOVE TO APERTURE", "STOP SYSTEM", "TEST COMMANDS"]
            n30 = event-data() -> ()  [unwired: 1 in, 6 out]
            n31 = local read "INTERLOCK STATE"() -> (w159:bool)
            n32 = local read "ION GUN"() -> (w156:bool)
            n33 = Not(x=w159) -> (.not. x?=w158:bool)
            n34 = And(x=w158, y=w156) -> (x .and. y?=w157:bool)
          }
          event "OBJ APERTURE ALIGNMENT": Value Change {
            w163 = T1[] [enum."SHIFT OBJECT APERTURE"] items=["LOOP", "OPEN SERIAL CONN TO ORSAY", "INITIALISE ORSAY", "READ SETTINGS", "SAVE SETTINGS", "OBJECTIVE LENS", "CONDENSOR LENS", "BLANKING TOGGLE", "TURN ON HEATER", "TURN OFF WOBBLER", "MEASURE HEATER OUTPUT", "TOGGLE GATE VALVE", "SCANNING CONTROLS", "TURN ON BEAM HV", "ENERGY RAMP CYCLE", "TURN ON SUPPRESSOR", "TURN ON EXTRACTOR", "TURN ON WIEN FILTER", "SET ENERGY RANGE", "MEASURE HV SUPPLY VOLTAGES", "SHUTDOWN ION SOURCE", "RESET TYPE II", "PROBE CURRENT FC#1", "PROBE CURRENT FC#2", "VACUUM ", "CHECK 150V", "INITIALISE PI MOTORS", "SET STIGMATOR", "SET WOBBLER FOR OBJECT", "SHIFT OBJECT APERTURE", "STORE OBJECT POSITION", "STORE APERTURE POSITION", "SHIFT MASS APERTURE", "DEFINE NEW APERTURE", "MOVE TO OBJECT", "MOVE TO APERTURE", "STOP SYSTEM", "TEST COMMANDS"]
            n35 = event-data() -> ()  [unwired: 1 in, 6 out]
            n36 = shared-variable "My Computer\\PI APERTURES.lvlib\\AGGREGATE HOMED ?"() -> (w162:bool)  [unwired: 1 in, 1 out]
          }
          event "OBJECT APERTURE": Value Change {
            w167 = T1[] [enum."MOVE TO OBJECT"] items=["LOOP", "OPEN SERIAL CONN TO ORSAY", "INITIALISE ORSAY", "READ SETTINGS", "SAVE SETTINGS", "OBJECTIVE LENS", "CONDENSOR LENS", "BLANKING TOGGLE", "TURN ON HEATER", "TURN OFF WOBBLER", "MEASURE HEATER OUTPUT", "TOGGLE GATE VALVE", "SCANNING CONTROLS", "TURN ON BEAM HV", "ENERGY RAMP CYCLE", "TURN ON SUPPRESSOR", "TURN ON EXTRACTOR", "TURN ON WIEN FILTER", "SET ENERGY RANGE", "MEASURE HV SUPPLY VOLTAGES", "SHUTDOWN ION SOURCE", "RESET TYPE II", "PROBE CURRENT FC#1", "PROBE CURRENT FC#2", "VACUUM ", "CHECK 150V", "INITIALISE PI MOTORS", "SET STIGMATOR", "SET WOBBLER FOR OBJECT", "SHIFT OBJECT APERTURE", "STORE OBJECT POSITION", "STORE APERTURE POSITION", "SHIFT MASS APERTURE", "DEFINE NEW APERTURE", "MOVE TO OBJECT", "MOVE TO APERTURE", "STOP SYSTEM", "TEST COMMANDS"]
            n37 = event-data() -> ()  [unwired: 1 in, 6 out]
            n38 = shared-variable "My Computer\\PI APERTURES.lvlib\\AGGREGATE HOMED ?"() -> (w165:bool)  [unwired: 1 in, 1 out]
          }
          event "APERTURE (MASS)": Value Change {
            w169 = T1[] [enum."MOVE TO APERTURE"] items=["LOOP", "OPEN SERIAL CONN TO ORSAY", "INITIALISE ORSAY", "READ SETTINGS", "SAVE SETTINGS", "OBJECTIVE LENS", "CONDENSOR LENS", "BLANKING TOGGLE", "TURN ON HEATER", "TURN OFF WOBBLER", "MEASURE HEATER OUTPUT", "TOGGLE GATE VALVE", "SCANNING CONTROLS", "TURN ON BEAM HV", "ENERGY RAMP CYCLE", "TURN ON SUPPRESSOR", "TURN ON EXTRACTOR", "TURN ON WIEN FILTER", "SET ENERGY RANGE", "MEASURE HV SUPPLY VOLTAGES", "SHUTDOWN ION SOURCE", "RESET TYPE II", "PROBE CURRENT FC#1", "PROBE CURRENT FC#2", "VACUUM ", "CHECK 150V", "INITIALISE PI MOTORS", "SET STIGMATOR", "SET WOBBLER FOR OBJECT", "SHIFT OBJECT APERTURE", "STORE OBJECT POSITION", "STORE APERTURE POSITION", "SHIFT MASS APERTURE", "DEFINE NEW APERTURE", "MOVE TO OBJECT", "MOVE TO APERTURE", "STOP SYSTEM", "TEST COMMANDS"]
            n39 = event-data() -> ()  [unwired: 1 in, 6 out]
            n40 = shared-variable "My Computer\\PI APERTURES.lvlib\\AGGREGATE HOMED ?"() -> (w168:bool)  [unwired: 1 in, 1 out]
          }
          event "MASS APERTURE ALIGNMENT": Value Change {
            w172 = T1[] [enum."SHIFT MASS APERTURE"] items=["LOOP", "OPEN SERIAL CONN TO ORSAY", "INITIALISE ORSAY", "READ SETTINGS", "SAVE SETTINGS", "OBJECTIVE LENS", "CONDENSOR LENS", "BLANKING TOGGLE", "TURN ON HEATER", "TURN OFF WOBBLER", "MEASURE HEATER OUTPUT", "TOGGLE GATE VALVE", "SCANNING CONTROLS", "TURN ON BEAM HV", "ENERGY RAMP CYCLE", "TURN ON SUPPRESSOR", "TURN ON EXTRACTOR", "TURN ON WIEN FILTER", "SET ENERGY RANGE", "MEASURE HV SUPPLY VOLTAGES", "SHUTDOWN ION SOURCE", "RESET TYPE II", "PROBE CURRENT FC#1", "PROBE CURRENT FC#2", "VACUUM ", "CHECK 150V", "INITIALISE PI MOTORS", "SET STIGMATOR", "SET WOBBLER FOR OBJECT", "SHIFT OBJECT APERTURE", "STORE OBJECT POSITION", "STORE APERTURE POSITION", "SHIFT MASS APERTURE", "DEFINE NEW APERTURE", "MOVE TO OBJECT", "MOVE TO APERTURE", "STOP SYSTEM", "TEST COMMANDS"]
            n41 = event-data() -> ()  [unwired: 1 in, 6 out]
            n42 = shared-variable "My Computer\\PI APERTURES.lvlib\\AGGREGATE HOMED ?"() -> (w171:bool)  [unwired: 1 in, 1 out]
          }
          event "STORE OBJECT": Mouse Down {
            w176 = T1[] [enum."STORE OBJECT POSITION"] items=["LOOP", "OPEN SERIAL CONN TO ORSAY", "INITIALISE ORSAY", "READ SETTINGS", "SAVE SETTINGS", "OBJECTIVE LENS", "CONDENSOR LENS", "BLANKING TOGGLE", "TURN ON HEATER", "TURN OFF WOBBLER", "MEASURE HEATER OUTPUT", "TOGGLE GATE VALVE", "SCANNING CONTROLS", "TURN ON BEAM HV", "ENERGY RAMP CYCLE", "TURN ON SUPPRESSOR", "TURN ON EXTRACTOR", "TURN ON WIEN FILTER", "SET ENERGY RANGE", "MEASURE HV SUPPLY VOLTAGES", "SHUTDOWN ION SOURCE", "RESET TYPE II", "PROBE CURRENT FC#1", "PROBE CURRENT FC#2", "VACUUM ", "CHECK 150V", "INITIALISE PI MOTORS", "SET STIGMATOR", "SET WOBBLER FOR OBJECT", "SHIFT OBJECT APERTURE", "STORE OBJECT POSITION", "STORE APERTURE POSITION", "SHIFT MASS APERTURE", "DEFINE NEW APERTURE", "MOVE TO OBJECT", "MOVE TO APERTURE", "STOP SYSTEM", "TEST COMMANDS"]
            n43 = event-data() -> ()  [unwired: 1 in, 8 out]
            n44 = shared-variable "My Computer\\PI APERTURES.lvlib\\AGGREGATE HOMED ?"() -> (w175:bool)  [unwired: 1 in, 1 out]
          }
          event "STORE APERTURE": Mouse Down {
            w178 = T1[] [enum."STORE APERTURE POSITION"] items=["LOOP", "OPEN SERIAL CONN TO ORSAY", "INITIALISE ORSAY", "READ SETTINGS", "SAVE SETTINGS", "OBJECTIVE LENS", "CONDENSOR LENS", "BLANKING TOGGLE", "TURN ON HEATER", "TURN OFF WOBBLER", "MEASURE HEATER OUTPUT", "TOGGLE GATE VALVE", "SCANNING CONTROLS", "TURN ON BEAM HV", "ENERGY RAMP CYCLE", "TURN ON SUPPRESSOR", "TURN ON EXTRACTOR", "TURN ON WIEN FILTER", "SET ENERGY RANGE", "MEASURE HV SUPPLY VOLTAGES", "SHUTDOWN ION SOURCE", "RESET TYPE II", "PROBE CURRENT FC#1", "PROBE CURRENT FC#2", "VACUUM ", "CHECK 150V", "INITIALISE PI MOTORS", "SET STIGMATOR", "SET WOBBLER FOR OBJECT", "SHIFT OBJECT APERTURE", "STORE OBJECT POSITION", "STORE APERTURE POSITION", "SHIFT MASS APERTURE", "DEFINE NEW APERTURE", "MOVE TO OBJECT", "MOVE TO APERTURE", "STOP SYSTEM", "TEST COMMANDS"]
            n45 = event-data() -> ()  [unwired: 1 in, 8 out]
            n46 = shared-variable "My Computer\\PI APERTURES.lvlib\\AGGREGATE HOMED ?"() -> (w179:bool)  [unwired: 1 in, 1 out]
          }
          event "ION GUN SETTINGS.EXTRACTOR": Value Change {
            w185 = T1[] [enum."TURN ON EXTRACTOR"] items=["LOOP", "OPEN SERIAL CONN TO ORSAY", "INITIALISE ORSAY", "READ SETTINGS", "SAVE SETTINGS", "OBJECTIVE LENS", "CONDENSOR LENS", "BLANKING TOGGLE", "TURN ON HEATER", "TURN OFF WOBBLER", "MEASURE HEATER OUTPUT", "TOGGLE GATE VALVE", "SCANNING CONTROLS", "TURN ON BEAM HV", "ENERGY RAMP CYCLE", "TURN ON SUPPRESSOR", "TURN ON EXTRACTOR", "TURN ON WIEN FILTER", "SET ENERGY RANGE", "MEASURE HV SUPPLY VOLTAGES", "SHUTDOWN ION SOURCE", "RESET TYPE II", "PROBE CURRENT FC#1", "PROBE CURRENT FC#2", "VACUUM ", "CHECK 150V", "INITIALISE PI MOTORS", "SET STIGMATOR", "SET WOBBLER FOR OBJECT", "SHIFT OBJECT APERTURE", "STORE OBJECT POSITION", "STORE APERTURE POSITION", "SHIFT MASS APERTURE", "DEFINE NEW APERTURE", "MOVE TO OBJECT", "MOVE TO APERTURE", "STOP SYSTEM", "TEST COMMANDS"]
            n47 = event-data() -> ()  [unwired: 1 in, 6 out]
            n48 = local read "INTERLOCK STATE"() -> (w184:bool)
            n49 = local read "ION GUN"() -> (w180:bool)
            n50 = Not(x=w184) -> (.not. x?=w181:bool)
            n51 = And(x=w181, y=w180) -> (x .and. y?=w182:bool)
          }
          event "ION GUN SETTINGS.BEAM ENERGY": Value Change {
            w187 = T1[] [enum."TURN ON BEAM HV"] items=["LOOP", "OPEN SERIAL CONN TO ORSAY", "INITIALISE ORSAY", "READ SETTINGS", "SAVE SETTINGS", "OBJECTIVE LENS", "CONDENSOR LENS", "BLANKING TOGGLE", "TURN ON HEATER", "TURN OFF WOBBLER", "MEASURE HEATER OUTPUT", "TOGGLE GATE VALVE", "SCANNING CONTROLS", "TURN ON BEAM HV", "ENERGY RAMP CYCLE", "TURN ON SUPPRESSOR", "TURN ON EXTRACTOR", "TURN ON WIEN FILTER", "SET ENERGY RANGE", "MEASURE HV SUPPLY VOLTAGES", "SHUTDOWN ION SOURCE", "RESET TYPE II", "PROBE CURRENT FC#1", "PROBE CURRENT FC#2", "VACUUM ", "CHECK 150V", "INITIALISE PI MOTORS", "SET STIGMATOR", "SET WOBBLER FOR OBJECT", "SHIFT OBJECT APERTURE", "STORE OBJECT POSITION", "STORE APERTURE POSITION", "SHIFT MASS APERTURE", "DEFINE NEW APERTURE", "MOVE TO OBJECT", "MOVE TO APERTURE", "STOP SYSTEM", "TEST COMMANDS"]
            n52 = event-data() -> ()  [unwired: 1 in, 6 out]
            n53 = local read "INTERLOCK STATE"() -> (w186:bool)
            n54 = local read "ION GUN"() -> (w191:bool)
            n55 = Not(x=w186) -> (.not. x?=w190:bool)
            n56 = And(x=w190, y=w191) -> (x .and. y?=w189:bool)
          }
          event "TEST COMMAND": Mouse Down {
            w192 = T1[] [enum."TEST COMMANDS"] items=["LOOP", "OPEN SERIAL CONN TO ORSAY", "INITIALISE ORSAY", "READ SETTINGS", "SAVE SETTINGS", "OBJECTIVE LENS", "CONDENSOR LENS", "BLANKING TOGGLE", "TURN ON HEATER", "TURN OFF WOBBLER", "MEASURE HEATER OUTPUT", "TOGGLE GATE VALVE", "SCANNING CONTROLS", "TURN ON BEAM HV", "ENERGY RAMP CYCLE", "TURN ON SUPPRESSOR", "TURN ON EXTRACTOR", "TURN ON WIEN FILTER", "SET ENERGY RANGE", "MEASURE HV SUPPLY VOLTAGES", "SHUTDOWN ION SOURCE", "RESET TYPE II", "PROBE CURRENT FC#1", "PROBE CURRENT FC#2", "VACUUM ", "CHECK 150V", "INITIALISE PI MOTORS", "SET STIGMATOR", "SET WOBBLER FOR OBJECT", "SHIFT OBJECT APERTURE", "STORE OBJECT POSITION", "STORE APERTURE POSITION", "SHIFT MASS APERTURE", "DEFINE NEW APERTURE", "MOVE TO OBJECT", "MOVE TO APERTURE", "STOP SYSTEM", "TEST COMMANDS"]
            n57 = event-data() -> ()  [unwired: 1 in, 8 out]
          }
          event "INTERLOCK HV": Mouse Down {
            w195 = T1[] [enum."RESET TYPE II"] items=["LOOP", "OPEN SERIAL CONN TO ORSAY", "INITIALISE ORSAY", "READ SETTINGS", "SAVE SETTINGS", "OBJECTIVE LENS", "CONDENSOR LENS", "BLANKING TOGGLE", "TURN ON HEATER", "TURN OFF WOBBLER", "MEASURE HEATER OUTPUT", "TOGGLE GATE VALVE", "SCANNING CONTROLS", "TURN ON BEAM HV", "ENERGY RAMP CYCLE", "TURN ON SUPPRESSOR", "TURN ON EXTRACTOR", "TURN ON WIEN FILTER", "SET ENERGY RANGE", "MEASURE HV SUPPLY VOLTAGES", "SHUTDOWN ION SOURCE", "RESET TYPE II", "PROBE CURRENT FC#1", "PROBE CURRENT FC#2", "VACUUM ", "CHECK 150V", "INITIALISE PI MOTORS", "SET STIGMATOR", "SET WOBBLER FOR OBJECT", "SHIFT OBJECT APERTURE", "STORE OBJECT POSITION", "STORE APERTURE POSITION", "SHIFT MASS APERTURE", "DEFINE NEW APERTURE", "MOVE TO OBJECT", "MOVE TO APERTURE", "STOP SYSTEM", "TEST COMMANDS"]
            n58 = event-data() -> ()  [unwired: 1 in, 8 out]
          }
          event "STOP": Mouse Down {
            w198 = T1[] [enum."SHUTDOWN ION SOURCE", enum."STOP SYSTEM"] items=["LOOP", "OPEN SERIAL CONN TO ORSAY", "INITIALISE ORSAY", "READ SETTINGS", "SAVE SETTINGS", "OBJECTIVE LENS", "CONDENSOR LENS", "BLANKING TOGGLE", "TURN ON HEATER", "TURN OFF WOBBLER", "MEASURE HEATER OUTPUT", "TOGGLE GATE VALVE", "SCANNING CONTROLS", "TURN ON BEAM HV", "ENERGY RAMP CYCLE", "TURN ON SUPPRESSOR", "TURN ON EXTRACTOR", "TURN ON WIEN FILTER", "SET ENERGY RANGE", "MEASURE HV SUPPLY VOLTAGES", "SHUTDOWN ION SOURCE", "RESET TYPE II", "PROBE CURRENT FC#1", "PROBE CURRENT FC#2", "VACUUM ", "CHECK 150V", "INITIALISE PI MOTORS", "SET STIGMATOR", "SET WOBBLER FOR OBJECT", "SHIFT OBJECT APERTURE", "STORE OBJECT POSITION", "STORE APERTURE POSITION", "SHIFT MASS APERTURE", "DEFINE NEW APERTURE", "MOVE TO OBJECT", "MOVE TO APERTURE", "STOP SYSTEM", "TEST COMMANDS"]
            n59 = event-data() -> ()  [unwired: 1 in, 8 out]
          }
          event "HIGH ENERGY": Value Change {
            w201 = T1[] [enum."SET ENERGY RANGE"] items=["LOOP", "OPEN SERIAL CONN TO ORSAY", "INITIALISE ORSAY", "READ SETTINGS", "SAVE SETTINGS", "OBJECTIVE LENS", "CONDENSOR LENS", "BLANKING TOGGLE", "TURN ON HEATER", "TURN OFF WOBBLER", "MEASURE HEATER OUTPUT", "TOGGLE GATE VALVE", "SCANNING CONTROLS", "TURN ON BEAM HV", "ENERGY RAMP CYCLE", "TURN ON SUPPRESSOR", "TURN ON EXTRACTOR", "TURN ON WIEN FILTER", "SET ENERGY RANGE", "MEASURE HV SUPPLY VOLTAGES", "SHUTDOWN ION SOURCE", "RESET TYPE II", "PROBE CURRENT FC#1", "PROBE CURRENT FC#2", "VACUUM ", "CHECK 150V", "INITIALISE PI MOTORS", "SET STIGMATOR", "SET WOBBLER FOR OBJECT", "SHIFT OBJECT APERTURE", "STORE OBJECT POSITION", "STORE APERTURE POSITION", "SHIFT MASS APERTURE", "DEFINE NEW APERTURE", "MOVE TO OBJECT", "MOVE TO APERTURE", "STOP SYSTEM", "TEST COMMANDS"]
            n60 = event-data() -> ()  [unwired: 1 in, 6 out]
            n61 = local read "INTERLOCK STATE"() -> (w204:bool)
            n62 = Not(x=w204) -> (.not. x?=w203:bool)
          }
          event "BEAM ON": Value Change {
            w208 = T1[] [enum."BLANKING TOGGLE"] items=["LOOP", "OPEN SERIAL CONN TO ORSAY", "INITIALISE ORSAY", "READ SETTINGS", "SAVE SETTINGS", "OBJECTIVE LENS", "CONDENSOR LENS", "BLANKING TOGGLE", "TURN ON HEATER", "TURN OFF WOBBLER", "MEASURE HEATER OUTPUT", "TOGGLE GATE VALVE", "SCANNING CONTROLS", "TURN ON BEAM HV", "ENERGY RAMP CYCLE", "TURN ON SUPPRESSOR", "TURN ON EXTRACTOR", "TURN ON WIEN FILTER", "SET ENERGY RANGE", "MEASURE HV SUPPLY VOLTAGES", "SHUTDOWN ION SOURCE", "RESET TYPE II", "PROBE CURRENT FC#1", "PROBE CURRENT FC#2", "VACUUM ", "CHECK 150V", "INITIALISE PI MOTORS", "SET STIGMATOR", "SET WOBBLER FOR OBJECT", "SHIFT OBJECT APERTURE", "STORE OBJECT POSITION", "STORE APERTURE POSITION", "SHIFT MASS APERTURE", "DEFINE NEW APERTURE", "MOVE TO OBJECT", "MOVE TO APERTURE", "STOP SYSTEM", "TEST COMMANDS"]
            n63 = event-data() -> ()  [unwired: 1 in, 6 out]
            n64 = local read "INTERLOCK STATE"() -> (w206:bool)
            n65 = Not(x=w206) -> (.not. x?=w205:bool)
          }
          event "WIEN", "E&B": Value Change {
            w209 = T1[] [enum."TURN ON WIEN FILTER"] items=["LOOP", "OPEN SERIAL CONN TO ORSAY", "INITIALISE ORSAY", "READ SETTINGS", "SAVE SETTINGS", "OBJECTIVE LENS", "CONDENSOR LENS", "BLANKING TOGGLE", "TURN ON HEATER", "TURN OFF WOBBLER", "MEASURE HEATER OUTPUT", "TOGGLE GATE VALVE", "SCANNING CONTROLS", "TURN ON BEAM HV", "ENERGY RAMP CYCLE", "TURN ON SUPPRESSOR", "TURN ON EXTRACTOR", "TURN ON WIEN FILTER", "SET ENERGY RANGE", "MEASURE HV SUPPLY VOLTAGES", "SHUTDOWN ION SOURCE", "RESET TYPE II", "PROBE CURRENT FC#1", "PROBE CURRENT FC#2", "VACUUM ", "CHECK 150V", "INITIALISE PI MOTORS", "SET STIGMATOR", "SET WOBBLER FOR OBJECT", "SHIFT OBJECT APERTURE", "STORE OBJECT POSITION", "STORE APERTURE POSITION", "SHIFT MASS APERTURE", "DEFINE NEW APERTURE", "MOVE TO OBJECT", "MOVE TO APERTURE", "STOP SYSTEM", "TEST COMMANDS"]
            n66 = event-data() -> ()  [unwired: 1 in, 6 out]
            n67 = local read "INTERLOCK STATE"() -> (w212:bool)
            n68 = Not(x=w212) -> (.not. x?=w211:bool)
          }
          event "SHUTDOWN": Mouse Down {
            w213 = T1[] [enum."SHUTDOWN ION SOURCE"] items=["LOOP", "OPEN SERIAL CONN TO ORSAY", "INITIALISE ORSAY", "READ SETTINGS", "SAVE SETTINGS", "OBJECTIVE LENS", "CONDENSOR LENS", "BLANKING TOGGLE", "TURN ON HEATER", "TURN OFF WOBBLER", "MEASURE HEATER OUTPUT", "TOGGLE GATE VALVE", "SCANNING CONTROLS", "TURN ON BEAM HV", "ENERGY RAMP CYCLE", "TURN ON SUPPRESSOR", "TURN ON EXTRACTOR", "TURN ON WIEN FILTER", "SET ENERGY RANGE", "MEASURE HV SUPPLY VOLTAGES", "SHUTDOWN ION SOURCE", "RESET TYPE II", "PROBE CURRENT FC#1", "PROBE CURRENT FC#2", "VACUUM ", "CHECK 150V", "INITIALISE PI MOTORS", "SET STIGMATOR", "SET WOBBLER FOR OBJECT", "SHIFT OBJECT APERTURE", "STORE OBJECT POSITION", "STORE APERTURE POSITION", "SHIFT MASS APERTURE", "DEFINE NEW APERTURE", "MOVE TO OBJECT", "MOVE TO APERTURE", "STOP SYSTEM", "TEST COMMANDS"]
            n69 = event-data() -> ()  [unwired: 1 in, 8 out]
          }
          event "FILAMENT HEATING", "FILAMENT": Value Change {
            w214 = T1[] [enum."TURN ON HEATER", enum."MEASURE HEATER OUTPUT"] items=["LOOP", "OPEN SERIAL CONN TO ORSAY", "INITIALISE ORSAY", "READ SETTINGS", "SAVE SETTINGS", "OBJECTIVE LENS", "CONDENSOR LENS", "BLANKING TOGGLE", "TURN ON HEATER", "TURN OFF WOBBLER", "MEASURE HEATER OUTPUT", "TOGGLE GATE VALVE", "SCANNING CONTROLS", "TURN ON BEAM HV", "ENERGY RAMP CYCLE", "TURN ON SUPPRESSOR", "TURN ON EXTRACTOR", "TURN ON WIEN FILTER", "SET ENERGY RANGE", "MEASURE HV SUPPLY VOLTAGES", "SHUTDOWN ION SOURCE", "RESET TYPE II", "PROBE CURRENT FC#1", "PROBE CURRENT FC#2", "VACUUM ", "CHECK 150V", "INITIALISE PI MOTORS", "SET STIGMATOR", "SET WOBBLER FOR OBJECT", "SHIFT OBJECT APERTURE", "STORE OBJECT POSITION", "STORE APERTURE POSITION", "SHIFT MASS APERTURE", "DEFINE NEW APERTURE", "MOVE TO OBJECT", "MOVE TO APERTURE", "STOP SYSTEM", "TEST COMMANDS"]
            n70 = event-data() -> ()  [unwired: 1 in, 6 out]
          }
          event "OBJECTIVE": Value Change {
            w220 = T1[] [enum."OBJECTIVE LENS"] items=["LOOP", "OPEN SERIAL CONN TO ORSAY", "INITIALISE ORSAY", "READ SETTINGS", "SAVE SETTINGS", "OBJECTIVE LENS", "CONDENSOR LENS", "BLANKING TOGGLE", "TURN ON HEATER", "TURN OFF WOBBLER", "MEASURE HEATER OUTPUT", "TOGGLE GATE VALVE", "SCANNING CONTROLS", "TURN ON BEAM HV", "ENERGY RAMP CYCLE", "TURN ON SUPPRESSOR", "TURN ON EXTRACTOR", "TURN ON WIEN FILTER", "SET ENERGY RANGE", "MEASURE HV SUPPLY VOLTAGES", "SHUTDOWN ION SOURCE", "RESET TYPE II", "PROBE CURRENT FC#1", "PROBE CURRENT FC#2", "VACUUM ", "CHECK 150V", "INITIALISE PI MOTORS", "SET STIGMATOR", "SET WOBBLER FOR OBJECT", "SHIFT OBJECT APERTURE", "STORE OBJECT POSITION", "STORE APERTURE POSITION", "SHIFT MASS APERTURE", "DEFINE NEW APERTURE", "MOVE TO OBJECT", "MOVE TO APERTURE", "STOP SYSTEM", "TEST COMMANDS"]
            n71 = event-data() -> ()  [unwired: 1 in, 6 out]
            n72 = local read "INTERLOCK STATE"() -> (w218:bool)
            n73 = Not(x=w218) -> (.not. x?=w217:bool)
          }
          event "CONDENSOR": Value Change {
            w224 = T1[] [enum."CONDENSOR LENS"] items=["LOOP", "OPEN SERIAL CONN TO ORSAY", "INITIALISE ORSAY", "READ SETTINGS", "SAVE SETTINGS", "OBJECTIVE LENS", "CONDENSOR LENS", "BLANKING TOGGLE", "TURN ON HEATER", "TURN OFF WOBBLER", "MEASURE HEATER OUTPUT", "TOGGLE GATE VALVE", "SCANNING CONTROLS", "TURN ON BEAM HV", "ENERGY RAMP CYCLE", "TURN ON SUPPRESSOR", "TURN ON EXTRACTOR", "TURN ON WIEN FILTER", "SET ENERGY RANGE", "MEASURE HV SUPPLY VOLTAGES", "SHUTDOWN ION SOURCE", "RESET TYPE II", "PROBE CURRENT FC#1", "PROBE CURRENT FC#2", "VACUUM ", "CHECK 150V", "INITIALISE PI MOTORS", "SET STIGMATOR", "SET WOBBLER FOR OBJECT", "SHIFT OBJECT APERTURE", "STORE OBJECT POSITION", "STORE APERTURE POSITION", "SHIFT MASS APERTURE", "DEFINE NEW APERTURE", "MOVE TO OBJECT", "MOVE TO APERTURE", "STOP SYSTEM", "TEST COMMANDS"]
            n74 = event-data() -> ()  [unwired: 1 in, 6 out]
            n75 = local read "INTERLOCK STATE"() -> (w222:bool)
            n76 = Not(x=w222) -> (.not. x?=w221:bool)
          }
          event "READ & APPLY SETUP": Mouse Down {
            w228 = T1[] [enum."READ SETTINGS"] items=["LOOP", "OPEN SERIAL CONN TO ORSAY", "INITIALISE ORSAY", "READ SETTINGS", "SAVE SETTINGS", "OBJECTIVE LENS", "CONDENSOR LENS", "BLANKING TOGGLE", "TURN ON HEATER", "TURN OFF WOBBLER", "MEASURE HEATER OUTPUT", "TOGGLE GATE VALVE", "SCANNING CONTROLS", "TURN ON BEAM HV", "ENERGY RAMP CYCLE", "TURN ON SUPPRESSOR", "TURN ON EXTRACTOR", "TURN ON WIEN FILTER", "SET ENERGY RANGE", "MEASURE HV SUPPLY VOLTAGES", "SHUTDOWN ION SOURCE", "RESET TYPE II", "PROBE CURRENT FC#1", "PROBE CURRENT FC#2", "VACUUM ", "CHECK 150V", "INITIALISE PI MOTORS", "SET STIGMATOR", "SET WOBBLER FOR OBJECT", "SHIFT OBJECT APERTURE", "STORE OBJECT POSITION", "STORE APERTURE POSITION", "SHIFT MASS APERTURE", "DEFINE NEW APERTURE", "MOVE TO OBJECT", "MOVE TO APERTURE", "STOP SYSTEM", "TEST COMMANDS"]
            n77 = event-data() -> ()  [unwired: 1 in, 8 out]
            n78 = local read "INTERLOCK STATE"() -> (w226:bool)
            n79 = Not(x=w226) -> (.not. x?=w225:bool)
          }
          event "SCANNING CLUSTER": Value Change {
            w231 = T1[] [enum."SCANNING CONTROLS"] items=["LOOP", "OPEN SERIAL CONN TO ORSAY", "INITIALISE ORSAY", "READ SETTINGS", "SAVE SETTINGS", "OBJECTIVE LENS", "CONDENSOR LENS", "BLANKING TOGGLE", "TURN ON HEATER", "TURN OFF WOBBLER", "MEASURE HEATER OUTPUT", "TOGGLE GATE VALVE", "SCANNING CONTROLS", "TURN ON BEAM HV", "ENERGY RAMP CYCLE", "TURN ON SUPPRESSOR", "TURN ON EXTRACTOR", "TURN ON WIEN FILTER", "SET ENERGY RANGE", "MEASURE HV SUPPLY VOLTAGES", "SHUTDOWN ION SOURCE", "RESET TYPE II", "PROBE CURRENT FC#1", "PROBE CURRENT FC#2", "VACUUM ", "CHECK 150V", "INITIALISE PI MOTORS", "SET STIGMATOR", "SET WOBBLER FOR OBJECT", "SHIFT OBJECT APERTURE", "STORE OBJECT POSITION", "STORE APERTURE POSITION", "SHIFT MASS APERTURE", "DEFINE NEW APERTURE", "MOVE TO OBJECT", "MOVE TO APERTURE", "STOP SYSTEM", "TEST COMMANDS"]
            n80 = event-data() -> ()  [unwired: 1 in, 6 out]
            n81 = local read "INTERLOCK STATE"() -> (w229:bool)
          }
          event "SAVE SETUP": Mouse Down {
            w234 = T1[] [enum."SAVE SETTINGS"] items=["LOOP", "OPEN SERIAL CONN TO ORSAY", "INITIALISE ORSAY", "READ SETTINGS", "SAVE SETTINGS", "OBJECTIVE LENS", "CONDENSOR LENS", "BLANKING TOGGLE", "TURN ON HEATER", "TURN OFF WOBBLER", "MEASURE HEATER OUTPUT", "TOGGLE GATE VALVE", "SCANNING CONTROLS", "TURN ON BEAM HV", "ENERGY RAMP CYCLE", "TURN ON SUPPRESSOR", "TURN ON EXTRACTOR", "TURN ON WIEN FILTER", "SET ENERGY RANGE", "MEASURE HV SUPPLY VOLTAGES", "SHUTDOWN ION SOURCE", "RESET TYPE II", "PROBE CURRENT FC#1", "PROBE CURRENT FC#2", "VACUUM ", "CHECK 150V", "INITIALISE PI MOTORS", "SET STIGMATOR", "SET WOBBLER FOR OBJECT", "SHIFT OBJECT APERTURE", "STORE OBJECT POSITION", "STORE APERTURE POSITION", "SHIFT MASS APERTURE", "DEFINE NEW APERTURE", "MOVE TO OBJECT", "MOVE TO APERTURE", "STOP SYSTEM", "TEST COMMANDS"]
            n82 = event-data() -> ()  [unwired: 1 in, 8 out]
          }
          event "WOBBLER SETTINBGS FOR OBJECT ALIGNMENT": Value Change {
            w236 = T1[] [enum."SET WOBBLER FOR OBJECT"] items=["LOOP", "OPEN SERIAL CONN TO ORSAY", "INITIALISE ORSAY", "READ SETTINGS", "SAVE SETTINGS", "OBJECTIVE LENS", "CONDENSOR LENS", "BLANKING TOGGLE", "TURN ON HEATER", "TURN OFF WOBBLER", "MEASURE HEATER OUTPUT", "TOGGLE GATE VALVE", "SCANNING CONTROLS", "TURN ON BEAM HV", "ENERGY RAMP CYCLE", "TURN ON SUPPRESSOR", "TURN ON EXTRACTOR", "TURN ON WIEN FILTER", "SET ENERGY RANGE", "MEASURE HV SUPPLY VOLTAGES", "SHUTDOWN ION SOURCE", "RESET TYPE II", "PROBE CURRENT FC#1", "PROBE CURRENT FC#2", "VACUUM ", "CHECK 150V", "INITIALISE PI MOTORS", "SET STIGMATOR", "SET WOBBLER FOR OBJECT", "SHIFT OBJECT APERTURE", "STORE OBJECT POSITION", "STORE APERTURE POSITION", "SHIFT MASS APERTURE", "DEFINE NEW APERTURE", "MOVE TO OBJECT", "MOVE TO APERTURE", "STOP SYSTEM", "TEST COMMANDS"]
            n83 = event-data() -> ()  [unwired: 1 in, 6 out]
            n84 = local read "INTERLOCK STATE"() -> (w235:bool)
          }
          event Value Change {
            w238 = T1[] [enum."SET STIGMATOR"] items=["LOOP", "OPEN SERIAL CONN TO ORSAY", "INITIALISE ORSAY", "READ SETTINGS", "SAVE SETTINGS", "OBJECTIVE LENS", "CONDENSOR LENS", "BLANKING TOGGLE", "TURN ON HEATER", "TURN OFF WOBBLER", "MEASURE HEATER OUTPUT", "TOGGLE GATE VALVE", "SCANNING CONTROLS", "TURN ON BEAM HV", "ENERGY RAMP CYCLE", "TURN ON SUPPRESSOR", "TURN ON EXTRACTOR", "TURN ON WIEN FILTER", "SET ENERGY RANGE", "MEASURE HV SUPPLY VOLTAGES", "SHUTDOWN ION SOURCE", "RESET TYPE II", "PROBE CURRENT FC#1", "PROBE CURRENT FC#2", "VACUUM ", "CHECK 150V", "INITIALISE PI MOTORS", "SET STIGMATOR", "SET WOBBLER FOR OBJECT", "SHIFT OBJECT APERTURE", "STORE OBJECT POSITION", "STORE APERTURE POSITION", "SHIFT MASS APERTURE", "DEFINE NEW APERTURE", "MOVE TO OBJECT", "MOVE TO APERTURE", "STOP SYSTEM", "TEST COMMANDS"]
            n85 = event-data() -> ()  [unwired: 1 in, 6 out]
            n86 = local read "INTERLOCK STATE"() -> (w239:bool)
          }
        }
      }
      frame True {
        w244 = T23[] [] items=["LOOP", "INIT STAGE CONTROLLER", "SEND COMMAND TO CONTROLLER", "HOME X", "HOME Y", "HOME Z", "ABORT ALL AXES", "GOTO MARKER", "ZERO XYZ", "READ XYZ POSITIONS", "GOTO XYZ POSITION", "STOP", "JOG XYZ", "WAIT FOR MOVE COMPLETE"]
        n87 = local write "ION GUN SETTINGS"(T22 {"BEAM ENERGY"=0.0, "EXTRACTOR"=0.0, "SUPPRESSOR"=0.0, "ION CURRENT"=0.0} ("ION GUN SETTINGS")) -> ()
      }
    }
    n88 = case shown="True" w64 {
      tunnel: w79 -> [w258 w268]
      tunnel: w78 -> [w257 w267]
      tunnel: [w258 w266] -> w77
      tunnel: [w257 w265] -> w74
      frame False {
      }
      frame True {
        w262 = string[] [] ("PROCESSES")
        n89 = local write "STOP"(FALSE ("STOP")) -> ()
        n90 = local write "ION GUN"(FALSE ("TURN ON GUN")) -> ()
        n91 = for {
          shift-right: [w271] -> w266
          shift-left: w268 -> [w273]
          shift-right: [w270] -> w265
          shift-left: w267 -> [w272]
          tunnel: "STARTUP" -> [w269] mode=indexing
          n92 = Enqueue Element(queue=w273, element=w269, error in (no error)=w272) -> (queue out=w271:refnum<queue>, error out=w270:errorcluster)  [unwired: 1 in, 1 out]
        }
        n93 = property on="FILAMENT HEATING" class="Slide (strict)"("DisabledEnum"=T21."Disabled and Grayed Out" ("Disabled")) -> ()  [unwired: 2 in, 2 out]
        n94 = call <vilib>:"Flush Shared Variable Data.vi"() -> ()  [unwired: 11 in, 1 out]
        "PROCESSES" <- w262
        "SERIAL \nRESPONSE" <- w262
        "PREVIOUS GUN SETTINGS" <- T2 {"BEAM ENERGY"=0.0, "SUPPRESSOR"=0.0, "EXTRACTOR"=0.0, "ION CURRENT"=0.0} ("PREVIOUS GUN SETTINGS")
      }
    }
    n95 = case shown="False" w64 {
      tunnel: [w96 FALSE] -> w59
      tunnel: [w95 w107] -> w58
      tunnel: [w94 FALSE] -> _
      frame False {
        n96 = event shown="[2] \"EXPOSURE\": Value Change" {
          selector: _ -> [_ _ _]
          dyn-events: _ -> [_ _ _]
          timeout: 150 -> [_ _ _]
          tunnel: [TRUE TRUE TRUE] -> w96
          tunnel: [FALSE TRUE TRUE] -> w94
          tunnel: [w98 w103 w106] -> w95
          event Timeout {
            w98 = T20[] [enum."LOOP"] items=["INIT VIDEO", "CAMERA GAIN", "CAMERA EXPOSURE", "LOOP"]
            n97 = event-data() -> ()  [unwired: 1 in, 3 out]
          }
          event "GAIN", "GAIN METHOD": Value Change {
            w103 = T20[] [enum."CAMERA GAIN"] items=["INIT VIDEO", "CAMERA GAIN", "CAMERA EXPOSURE", "LOOP"]
            n98 = event-data() -> ()  [unwired: 1 in, 6 out]
          }
          event "EXPOSURE": Value Change {
            w106 = T20[] [enum."CAMERA EXPOSURE"] items=["INIT VIDEO", "CAMERA GAIN", "CAMERA EXPOSURE", "LOOP"]
            n99 = event-data() -> ()  [unwired: 1 in, 6 out]
          }
        }
      }
      frame True {
        w107 = T20[] [] items=["INIT VIDEO", "CAMERA GAIN", "CAMERA EXPOSURE", "LOOP"]
      }
    }
    n100 = case shown="True" w64 {
      tunnel: w63 -> [w111 w116]
      tunnel: w62 -> [w110 w115]
      tunnel: [w111 w114] -> w61
      tunnel: [w110 w113] -> w60
      frame False {
      }
      frame True {
        w112 = T20[] [enum."INIT VIDEO", enum."CAMERA EXPOSURE"] items=["INIT VIDEO", "CAMERA GAIN", "CAMERA EXPOSURE", "LOOP"]
        n101 = for {
          shift-right: [w119] -> w114
          shift-left: w116 -> [w121]
          shift-right: [w118] -> w113
          shift-left: w115 -> [w120]
          tunnel: w112 -> [w117] mode=indexing
          n102 = Enqueue Element(queue=w121, element=w117, error in (no error)=w120) -> (queue out=w119:refnum<queue>, error out=w118:errorcluster)  [unwired: 1 in, 1 out]
        }
      }
    }
    n103 = local read "ION GUN SETTINGS"() -> (w43:T2)
    n104 = case shown="True" w59 {
      tunnel: w61 -> [w83 w88]
      tunnel: w58 -> [_ w87]
      tunnel: [w83 w86] -> w57
      tunnel: [w82 w85] -> w56
      tunnel: w60 -> [w82 w84]
      frame False {
      }
      frame True {
        n105 = for {
          shift-right: [w91] -> w86
          shift-left: w88 -> [w93]
          shift-right: [w90] -> w85
          shift-left: w84 -> [w92]
          tunnel: w87 -> [w89] mode=indexing
          n106 = Enqueue Element(queue=w93, element=w89, error in (no error)=w92) -> (queue out=w91:refnum<queue>, error out=w90:errorcluster)  [unwired: 1 in, 1 out]
        }
      }
    }
    n107 = case shown="True" w76 {
      tunnel: w77 -> [w246 w251]
      tunnel: w75 -> [_ w250]
      tunnel: [w246 w249] -> w73
      tunnel: [w245 w248] -> w70
      tunnel: w74 -> [w245 w247]
      frame False {
      }
      frame True {
        n108 = for {
          shift-right: [w254] -> w249
          shift-left: w251 -> [w256]
          shift-right: [w253] -> w248
          shift-left: w247 -> [w255]
          tunnel: w250 -> [w252] mode=indexing
          n109 = Enqueue Element(queue=w256, element=w252, error in (no error)=w255) -> (queue out=w254:refnum<queue>, error out=w253:errorcluster)  [unwired: 1 in, 1 out]
        }
      }
    }
    n110 = Unbundle By Name(w43) -> ("BEAM ENERGY"=w35:sgl[unit])
    n111 = local read "VACUUM STATE"() -> (w66:bool)
    n112 = local read "150V GOOD"() -> (w67:bool)
    n113 = Greater Or Equal?(x=w35, y=sgl[unit] 10000.0) -> (x >= y?=→"HIGH ENERGY":bool)
    n114 = node("SETTINGS DELAY") -> (w38:dbl)
    n115 = Or(x=w70, y=w72) -> (x .or. y?=w40:bool)
    n116 = To Unsigned Long Integer(number=w38) -> (unsigned 32bit integer=→"TIMER":u32)
    n117 = local read "CONDENSOR"() -> (w45:cluster{"COARSE":sgl[unit], "FINE":sgl[unit]})
    n118 = Compound Arithmetic op=AND(w66, w67) -> (w53:bool)
    n119 = local read "OBJECTIVE"() -> (w44:cluster{"COARSE":sgl[unit], "FINE":sgl[unit]})
    n120 = property on="PROCESSES" class="Arr (strict)"() -> ("Index Values"=w52:u32[])  [unwired: 2 in, 2 out]
    n121 = Not(x=w53) -> (.not. x?=→"INTERLOCK STATE":bool)
    n122 = case shown="True" w53 {
      tunnel: [T21."Disabled and Grayed Out" ("Disabled") T21."Enabled" ("Disabled")] -> w55
      tunnel: [TRUE FALSE] -> w65
      frame False {
      }
      frame True {
      }
    }
    n123 = Unbundle By Name(w44) -> ("COARSE"=w47:sgl[unit], "FINE"=w46:sgl[unit])
    n124 = Unbundle By Name(w45) -> ("COARSE"=w48:sgl[unit], "FINE"=w49:sgl[unit])
    n125 = property on="SERIAL \nRESPONSE" class="Arr (strict)"("Index Values"=w52) -> ()  [unwired: 2 in, 2 out]
    n126 = Get Queue Status(queue=w73, return elements? (F)=TRUE, error in (no error)=w70) -> (queue out=w71:refnum<queue>, error out=w68:errorcluster, elements=→"elements":T1[])  [unwired: 5 out]
    n127 = Add(x=w48, y=w49) -> (x+y=→"CONDENSOR":sgl[unit])
    n128 = Add(x=w47, y=w46) -> (x+y=→"OBJECTIVE":sgl[unit])
    n129 = First Call?() -> (First Call?: T/F=w39:bool)
    n130 = case shown="True" w39 {
      frame False {
      }
      frame True {
        w80 = dbl[unit][] [] ("History Data")
        w81 = dbl[unit][] [] ("History Data")
        n131 = property on="BEAM VOLTAGE" class="WFChart (strict)"("History Data"=w81) -> ()  [unwired: 2 in, 2 out]
        n132 = property on="BEAM CURRENT" class="WFChart (strict)"("History Data"=w80) -> ()  [unwired: 2 in, 2 out]
        n133 = property on="EXTRACTOR  CURRENT" class="WFChart (strict)"("History Data"=w80) -> ()  [unwired: 2 in, 2 out]
        n134 = property on="EXTRACTOR" class="WFChart (strict)"("History Data"=w81) -> ()  [unwired: 2 in, 2 out]
        n135 = property on="CONDENSOR CURRENT" class="WFChart (strict)"("History Data"=w80) -> ()  [unwired: 2 in, 2 out]
        n136 = property on="CONDENSOR VOLTAGE" class="WFChart (strict)"("History Data"=w81) -> ()  [unwired: 2 in, 2 out]
        n137 = property on="OBJECTIVE CURRENT" class="WFChart (strict)"("History Data"=w80) -> ()  [unwired: 2 in, 2 out]
        n138 = property on="OBJECTIVE VOLTAGE" class="WFChart (strict)"("History Data"=w81) -> ()  [unwired: 2 in, 2 out]
        n139 = property on="SUPPRESSOR CURRENT" class="WFChart (strict)"("History Data"=w80) -> ()  [unwired: 2 in, 2 out]
        n140 = property on="SUPPRESSOR VOLTAGE" class="WFChart (strict)"("History Data"=w81) -> ()  [unwired: 2 in, 2 out]
      }
    }
    n141 = property on="BEAM ON" class="Bool (strict)"("DisabledEnum"=w55) -> ()  [unwired: 2 in, 2 out]
    n142 = property on="ION GUN" class="Bool (strict)"("DisabledEnum"=w55) -> ()  [unwired: 2 in, 2 out]
    n143 = property on="WARNING" class="Str"("DisabledEnum"=w55) -> ()  [unwired: 2 in, 2 out]
    n144 = property on="INTERLOCK STATE" class="Bool (strict)"("Blinking"=w65) -> ()  [unwired: 2 in, 2 out]
    n145 = property on="ION GUN SETTINGS" class="Clust (strict)"("DisabledEnum"=w55) -> ()  [unwired: 2 in, 2 out]
  }
  n146 = while {
    shift-right: [w280] -> _
    shift-left: string[] [] -> [w281]
    shift-right: [w275] -> _
    shift-left: string[] [] -> [w279]
    shift-right: [w278] -> _
    shift-left: w7 -> [w276]
    border: i32[] [] -> [_]
    border: dbl[unit][] [] -> [_]
    border: 0 -> [_]
    stop <- TRUE continue-if-true
    n147 = Dequeue Element(queue=w276) -> (queue out=w277:refnum<queue>, element=w282:T1)  [unwired: 2 in, 2 out]
    n148 = case shown="\"READ SETTINGS\"" w282 {
      tunnel: w281 -> [w295 w316 w373 w404 w431 w515 w534 w578 w633 w647 w652 w663 w722 w770 w801 w831 w856 w932 w963 w1043 w1118 w1167 w1186 w1223 w1230 w1275 w1452 w1512 w1559 w1575 w1579 w1592 w1604 w1611 w1622 w1636 w1701]
      tunnel: [w293 w314 w371 w404 w430 w513 w533 w579 w633 w648 w652 w660 w721 w769 w800 w831 w855 w932 w962 w1042 w1118 w1167 w1186 w1222 w1228 w1275 w1452 w1509 w1557 w1575 w1579 w1592 w1604 w1611 w1622 w1636 w1701] -> w280
      tunnel: w279 -> [w292 w312 w374 w403 w429 w511 w532 w580 w631 w635 w650 w662 w757 w768 w802 w843 w858 w933 w965 w1045 w1119 w1168 w1188 w1220 w1231 w1273 w1450 w1510 w1560 w1573 w1577 w1590 w1605 w1612 w1620 w1635 w1700]
      tunnel: [w289 w310 w369 w403 w424 w505 w529 w568 w631 w635 w650 w657 w757 w765 w795 w828 w857 w933 w964 w1044 w1119 w1168 w1188 w1220 w1225 w1273 w1450 w1507 w1555 w1573 w1577 w1590 w1605 w1612 w1620 w1633 w1698] -> w275
      tunnel: [w290 w311 w370 w402 w425 w525 w530 w570 w632 w645 w651 w658 w758 w766 w796 w830 w853 w934 w960 w1040 w1120 w1166 w1187 w1221 w1226 w1274 w1451 w1508 w1556 w1574 w1578 w1591 w1606 w1613 w1621 w1637 w1702] -> w278
      tunnel: w277 -> [w290 w311 w370 w402 w426 w525 w530 w570 w632 w645 w651 w658 w758 w766 w796 w830 w853 w934 w960 w1040 w1120 w1166 w1187 w1221 w1226 w1274 w1451 w1508 w1556 w1574 w1578 w1591 w1606 w1613 w1621 w1637 w1702]
      frame "LOOP", Default {
        w283 = T27 16 items=["Flush Receive Buffer"=16, "Write Transmit Buffer to Device"=32, "Flush Receive Buffer (No I/O)"=64, "Flush Transmit Buffer"=128] ("Mask")
        w288 = dbl[unit][] [] ("EXTRACTOR RAMP")
        w294 = "LOOP" ("PROCESS")
        n149 = local read "WOBBLER SETTINBGS FOR OBJECT ALIGNMENT"() -> (w297:T11)
        n150 = Unbundle By Name(w297) -> ("WOBBLE"=w296:u16)
        n151 = local write "PROCESS"(w294) -> ()
        n152 = local read "VISA ERROR"() -> (w286:errorcluster)
        n153 = local read "ORSAY"() -> (w285:refnum<visa-resource-name>)
        n154 = case shown="1" w296 {
          tunnel: [TRUE FALSE FALSE] -> w300
          tunnel: [FALSE TRUE FALSE] -> w299
          tunnel: [FALSE FALSE TRUE] -> w298
          frame 0, Default {
          }
          frame 1 {
          }
          frame 2 {
          }
        }
        n155 = Build Array (concatenate)(w295, w294) -> (w293:string[])
        n156 = property class="DigNum (strict)"("Blinking"=w300) -> ()  [unwired: 2 in, 2 out]
        n157 = property class="DigNum (strict)"("Blinking"=w299) -> ()  [unwired: 2 in, 2 out]
        n158 = property class="DigNum (strict)"("Blinking"=w298) -> ()  [unwired: 2 in, 2 out]
        n159 = VISA Flush I/O Buffer(VISA resource name=w285, mask (16)=w283, error in (no error)=w286) -> (VISA resource name out=w284:refnum<visa-resource-name>, error out=w287:errorcluster)
        n160 = local write "PROCESSES"(w293) -> ()
        n161 = local write "ORSAY"(w284) -> ()
        n162 = local write "VISA ERROR"(w287) -> ()
        n163 = local write "EXTRACTOR RAMP"(w288) -> ()
        n164 = local write "BEAM RAMP"(w288) -> ()
        n165 = local write "SUPPRESSOR RAMP"(w288) -> ()
        n166 = Build Array (concatenate)(w292, "LOOP") -> (w289:string[])
        n167 = local write "SERIAL \nRESPONSE"(w289) -> ()
      }
      frame "OPEN SERIAL CONN TO ORSAY" {
        w315 = "OPENING SERIAL CONNECTION TO ORSAY MB" ("PROCESS")
        n168 = flat-sequence {
          tunnel: [w328] -> w313
          frame #0 {
            w320 = T27 128 items=["Flush Receive Buffer"=16, "Write Transmit Buffer to Device"=32, "Flush Receive Buffer (No I/O)"=64, "Flush Transmit Buffer"=128] ("Mask")
            w337 = T27 16 items=["Flush Receive Buffer"=16, "Write Transmit Buffer to Device"=32, "Flush Receive Buffer (No I/O)"=64, "Flush Transmit Buffer"=128] ("Mask")
            n169 = case shown="0, Default" "TERMINATION CHAR" {
              tunnel: [0 13 10] -> w326
              tunnel: [w349 w352 w357] -> w325
              tunnel: [w348 w351 w356] -> w324
              tunnel: ["" "\r" "\n"] -> w317
              frame 0, Default {
                w348 = u16 0 items=["None", "Last Bit", "TermChar"] ("Serial Settings:End Mode for Reads")
                w349 = u16 0 items=["None", "Last Bit", "TermChar"] ("Serial Settings:End Mode for Reads")
              }
              frame 1 {
                w351 = u16 0 items=["None", "Last Bit", "TermChar"] ("Serial Settings:End Mode for Reads")
                w352 = u16 2 items=["None", "Last Bit", "TermChar"] ("Serial Settings:End Mode for Reads")
              }
              frame 2 {
                w356 = u16 0 items=["None", "Last Bit", "TermChar"] ("Serial Settings:End Mode for Reads")
                w357 = u16 2 items=["None", "Last Bit", "TermChar"] ("Serial Settings:End Mode for Reads")
              }
            }
            "APPEND" <- w317
            n170 = call-poly "VISA Configure Serial Port"("VISA resource name"=refnum<visa-resource-name> "ORSAY-USB", "Enable Termination\nChar (T)"=FALSE ("Enable Termination\nChar (T)"), "baud rate (9600)"=9600) -> ("VISA resource name out"=w341:refnum<visa-resource-name>, "error out"=w340:errorcluster)  [unwired: 11 in]
            n171 = property class="Instr"(reference=w341, error in=w340, "Serial Settings:End Mode for Writes"=w325, "Message Based Settings:Send End Enable"="TERMINATION", "Message Based Settings:Termination Character"=w326, "ASRL End In"=w324) -> (reference out=w332:refnum<visa-resource-name>, error out=w330:errorcluster)
            n172 = flat-sequence {
              tunnel: [w360] -> w331
              tunnel: w332 -> [w360]
              tunnel: [w359] -> w329
              tunnel: w330 -> [w359]
              frame #0 {
                n173 = Wait (ms)(milliseconds to wait=u32 200) -> ()  [unwired: 1 out]
              }
            }
            n174 = property class="Instr"(reference=w331, error in=w329) -> (reference out=w336:refnum<visa-resource-name>, error out=w333:errorcluster, "Serial Settings:Number of Bytes at Serial Port"=w334:u32)
            n175 = VISA Read(VISA resource name=w336, byte count=w334, error in (no error)=w333) -> (VISA resource name out=w335:refnum<visa-resource-name>, read buffer=w328:string, error out=w322:errorcluster)  [unwired: 1 out]
            n176 = VISA Flush I/O Buffer(VISA resource name=w335, mask (16)=w320, error in (no error)=w322) -> (VISA resource name out=w323:refnum<visa-resource-name>, error out=w321:errorcluster)
            n177 = VISA Flush I/O Buffer(VISA resource name=w323, mask (16)=w337, error in (no error)=w321) -> (VISA resource name out=→"ORSAY":refnum<visa-resource-name>, error out=→"VISA ERROR":errorcluster)
            n178 = Unbundle By Name(w321) -> ("status"=w343:bool)
            n179 = Not(x=w343) -> (.not. x?=→"ORSAY CONNECTED":bool)
          }
          frame #1 {
            n180 = Wait (ms)(milliseconds to wait=u32 2000 ("millisecond timer value")) -> ()  [unwired: 1 out]
          }
        }
        n181 = local write "PROCESS"(w315) -> ()
        n182 = Build Array (concatenate)(w316, w315) -> (w314:string[])
        n183 = Build Array (concatenate)(w312, w313) -> (w310:string[])
        n184 = local write "SERIAL \nRESPONSE"(w310) -> ()
      }
      frame "INITIALISE ORSAY" {
        w364 = cluster{"COARSE":sgl[unit], "FINE":sgl[unit]} {"COARSE"=0.0, "FINE"=0.0} ("CONDENSOR")
        w368 = dbl[unit][] [] ("SUPPRESSOR RAMP")
        w372 = "RESET ORSAY" ("PROCESS")
        n185 = flat-sequence {
          tunnel: [w382] -> w375
          tunnel: "DS CF12,58A4,30EE,58A4,7630,24B2,7630,DB4E,0" -> [w379]
          frame #0 {
            n186 = local read "APPEND"() -> (w380:string)
            n187 = Concatenate Strings("RE 1" ("ORSAY COMMAND"), w380) -> (w377:string)
            n188 = Concatenate Strings(w379, w380) -> (w376:string)
            n189 = local read "ORSAY"() -> (w384:refnum<visa-resource-name>)
            n190 = Build Array(w377, w376) -> (w378:string[])
            n191 = for {
              tunnel: [w397] -> w385
              tunnel: [w394] -> w382
              tunnel: w378 -> [w386] mode=indexing
              shift-right: [w395] -> w383
              shift-left: w384 -> [w396]
              n192 = VISA Write(VISA resource name=w396, write buffer=w386) -> (VISA resource name out=w390:refnum<visa-resource-name>, error out=w389:errorcluster)  [unwired: 1 in, 1 out]
              n193 = flat-sequence {
                tunnel: w390 -> [w398]
                tunnel: [w400] -> w387
                tunnel: w389 -> [w400]
                tunnel: [w398] -> w388
                frame #0 {
                  n194 = Wait (ms)(milliseconds to wait=u32 1000) -> ()  [unwired: 1 out]
                }
              }
              n195 = property class="Instr"(reference=w388, error in=w387) -> (reference out=w391:refnum<visa-resource-name>, error out=w393:errorcluster, "Serial Settings:Number of Bytes at Serial Port"=w392:u32)
              n196 = VISA Read(VISA resource name=w391, byte count=w392, error in (no error)=w393) -> (VISA resource name out=w395:refnum<visa-resource-name>, read buffer=w394:string, error out=w397:errorcluster)  [unwired: 1 out]
            }
            n197 = local write "ORSAY"(w383) -> ()
            n198 = local write "VISA ERROR"(w385) -> ()
          }
          frame #1 {
            n199 = Wait (ms)(milliseconds to wait=u32 200) -> ()  [unwired: 1 out]
          }
        }
        n200 = Build Array (concatenate)(w373, w372) -> (w371:string[])
        n201 = local write "PROCESS"(w372) -> ()
        n202 = Build Array (concatenate)(w374, w375) -> (w369:string[])
        n203 = local write "SERIAL \nRESPONSE"(w369) -> ()
        n204 = local write "CONDENSOR"(w364) -> ()
        n205 = local write "OBJECTIVE"(w364) -> ()
        n206 = property on="SUPPRESSOR" class="Slide (strict)"("DisabledEnum"=T21."Disabled and Grayed Out" ("Disabled")) -> ()  [unwired: 2 in, 2 out]
        n207 = property on="ION CURRENT" class="Slide (strict)"("DisabledEnum"=T21."Disabled and Grayed Out" ("Disabled")) -> ()  [unwired: 2 in, 2 out]
        n208 = property on="EXTRACTOR" class="Slide (strict)"("DisabledEnum"=T21."Disabled and Grayed Out" ("Disabled")) -> ()  [unwired: 2 in, 2 out]
        n209 = property on="SUPPRESSOR" class="Slide (strict)" props=["DisabledEnum"]() -> ()  [unwired: 2 in, 3 out]
        n210 = local write "ION GUN SETTINGS"(T22 {"BEAM ENERGY"=0.0, "EXTRACTOR"=0.0, "SUPPRESSOR"=0.0, "ION CURRENT"=0.0} ("ION GUN SETTINGS")) -> ()
        n211 = local write "EXTRACTOR RAMP"(w368) -> ()
        n212 = local write "BEAM RAMP"(w368) -> ()
        n213 = local write "SUPPRESSOR RAMP"(w368) -> ()
        "SUPPRESSOR RAMP" <- w368
        "EXTRACTOR RAMP" <- w368
        "BEAM RAMP" <- w368
      }
      frame "TEST COMMANDS" {
        n214 = flat-sequence {
          frame #0 {
            n215 = local read "APPEND"() -> (w415:string)
            n216 = Concatenate Strings("TEST COMMAND", w415) -> (w406:string)
            n217 = local read "VISA ERROR"() -> (w416:errorcluster)
            n218 = local read "ORSAY"() -> (w417:refnum<visa-resource-name>)
            n219 = VISA Write(VISA resource name=w417, write buffer=w406, error in (no error)=w416) -> (VISA resource name out=w410:refnum<visa-resource-name>, error out=w409:errorcluster)  [unwired: 1 out]
            n220 = flat-sequence {
              tunnel: w410 -> [w420]
              tunnel: [w422] -> w407
              tunnel: w409 -> [w422]
              tunnel: [w420] -> w408
              frame #0 {
                n221 = Wait (ms)(milliseconds to wait=u32 1000) -> ()  [unwired: 1 out]
              }
            }
            n222 = property class="Instr"(reference=w408, error in=w407) -> (reference out=w411:refnum<visa-resource-name>, error out=w413:errorcluster, "Serial Settings:Number of Bytes at Serial Port"=w412:u32)
            n223 = VISA Read(VISA resource name=w411, byte count=w412, error in (no error)=w413) -> (VISA resource name out=w419:refnum<visa-resource-name>, read buffer=→"TEST OUTPUT":string, error out=w418:errorcluster)  [unwired: 1 out]
            n224 = local write "ORSAY"(w419) -> ()
            n225 = local write "VISA ERROR"(w418) -> ()
          }
          frame #1 {
            n226 = local write "TEST COMMAND"(FALSE ("TEST COMMAND")) -> ()
          }
        }
      }
      frame "VACUUM " {
        w432 = "VACUUM CHECK"
        w465 = i16 2
        w464 = i16 2
        # "Bypass"
        # "Where is the column vac ?\nMust be before manual GV"
        # "Need a measure of vac in the target chamber & valve ??"
        n227 = local read "VISA ERROR"() -> (w482:errorcluster)
        n228 = local read "APPEND"() -> (w428:string)
        n229 = local read "ORSAY"() -> (w483:refnum<visa-resource-name>)
        n230 = Concatenate Strings("GV F", w428) -> (w444:string)
        n231 = Concatenate Strings("GV D", w428) -> (w442:string)
        n232 = VISA Write(VISA resource name=w483, write buffer=w444, error in (no error)=w482) -> (VISA resource name out=w440:refnum<visa-resource-name>, error out=w438:errorcluster)  [unwired: 1 out]
        n233 = flat-sequence {
          tunnel: [w495] -> w434
          tunnel: w437 -> [w495]
          tunnel: [w494] -> w435
          tunnel: w436 -> [w494]
          frame #0 {
            n234 = Wait (ms)(milliseconds to wait=u32 200) -> ()  [unwired: 1 out]
          }
        }
        n235 = flat-sequence {
          tunnel: [w498] -> w441
          tunnel: w440 -> [w498]
          tunnel: [w497] -> w439
          tunnel: w438 -> [w497]
          frame #0 {
            n236 = Wait (ms)(milliseconds to wait=u32 200) -> ()  [unwired: 1 out]
          }
        }
        n237 = property class="Instr"(reference=w441, error in=w439) -> (reference out=w451:refnum<visa-resource-name>, error out=w450:errorcluster, "Serial Settings:Number of Bytes at Serial Port"=w449:u32)
        n238 = property class="Instr"(reference=w434, error in=w435) -> (reference out=w448:refnum<visa-resource-name>, error out=w446:errorcluster, "Serial Settings:Number of Bytes at Serial Port"=w447:u32)
        n239 = VISA Read(VISA resource name=w451, byte count=w449, error in (no error)=w450) -> (VISA resource name out=w463:refnum<visa-resource-name>, read buffer=w453:string)  [unwired: 2 out]
        n240 = VISA Write(VISA resource name=w463, write buffer=w442) -> (VISA resource name out=w437:refnum<visa-resource-name>, error out=w436:errorcluster)  [unwired: 1 in, 1 out]
        n241 = VISA Read(VISA resource name=w448, byte count=w447, error in (no error)=w446) -> (VISA resource name out=w462:refnum<visa-resource-name>, read buffer=w452:string, error out=w461:errorcluster)  [unwired: 1 out]
        n242 = local write "ORSAY"(w462) -> ()
        n243 = local write "VISA ERROR"(w461) -> ()
        n244 = Concatenate Strings(w453, w452) -> (w433:string)
        n245 = Match Pattern(string=w453, regular expression=",") -> (before substring=w471:string)  [unwired: 1 in, 3 out]
        n246 = Match Pattern(string=w452, regular expression=",") -> (before substring=w473:string)  [unwired: 1 in, 3 out]
        n247 = property on="COLUMN VACUUM" class="Knob (strict)"("Scale.RampVis"=TRUE ("Scale.Ramp Visible")) -> ()  [unwired: 2 in, 2 out]
        n248 = local write "PROCESS"(w432) -> ()
        n249 = Hexadecimal String To Number(string=w471, offset=w464, default (0uL)=w464) -> (number=w475:i16)  [unwired: 1 out]
        n250 = Hexadecimal String To Number(string=w473, offset=w465, default (0uL)=w465) -> (number=w472:i16)  [unwired: 1 out]
        n251 = Absolute Value(x=w472) -> (abs(x)=w477:i16)
        n252 = Less?(x=w475, y=320) -> (x < y?=w478:bool)
        n253 = Build Array (concatenate)(w431, w432) -> (w430:string[])
        n254 = Equal To 0?(x=w475) -> (x = 0?=w474:bool)
        n255 = Equal To 0?(x=w477) -> (x = 0?=w476:bool)
        n256 = Build Array (concatenate)(w429, w433) -> (w424:string[])
        n257 = local write "PROCESSES"(w430) -> ()
        n258 = Select(t=i16 1, s=w474, f=w475) -> (s? t:f=w479:i16)
        n259 = Select(t=i16 1, s=w476, f=w477) -> (s? t:f=w480:i16)
        n260 = case shown="True" w478 {
          tunnel: w479 -> [w500 _]
          tunnel: w480 -> [_ w503]
          tunnel: [w499 w504] -> w481
          frame False {
            n261 = To Single Precision Float(number=w500) -> (single precision float=w499:sgl)
          }
          frame True {
            n262 = To Single Precision Float(number=w503) -> (single precision float=w501:sgl)
            n263 = Divide(x=w501, y=sgl 20.0) -> (x/y=w504:sgl)
          }
        }
        n264 = formula code="k=log(lp/3276700)-2.7;\np=10** k;"("lp"=w481) -> ("p"=w459:dbl)  [unwired: 1 out]
        n265 = node(w459) -> (w454:dbl[unit])
        "COLUMN VACUUM" <- w454
        n266 = Bundle(w454, "COLUMN THRESHOLD"="COLUMN THRESHOLD") -> (→"COLUMN VACUUM":cluster{dbl[unit], "COLUMN THRESHOLD":dbl[unit]})  [unwired: 1 in]
        n267 = Bundle(w454, "CHAMBER THRESHOLD"="CHAMBER THRESHOLD") -> (→"CHAMBER VACUUM":T28)  [unwired: 1 in]
        n268 = Less?(x=w454, y="COLUMN THRESHOLD") -> (x < y?=w427:bool)
        "VACUUM STATE" <- w427
        n269 = case shown="False" w427 {
          tunnel: w426 -> [w488 w492]
          tunnel: [w487 w492] -> w425
          frame False {
            w486 = T1[] [enum."TOGGLE GATE VALVE", enum."RESET TYPE II"] items=["LOOP", "OPEN SERIAL CONN TO ORSAY", "INITIALISE ORSAY", "READ SETTINGS", "SAVE SETTINGS", "OBJECTIVE LENS", "CONDENSOR LENS", "BLANKING TOGGLE", "TURN ON HEATER", "TURN OFF WOBBLER", "MEASURE HEATER OUTPUT", "TOGGLE GATE VALVE", "SCANNING CONTROLS", "TURN ON BEAM HV", "ENERGY RAMP CYCLE", "TURN ON SUPPRESSOR", "TURN ON EXTRACTOR", "TURN ON WIEN FILTER", "SET ENERGY RANGE", "MEASURE HV SUPPLY VOLTAGES", "SHUTDOWN ION SOURCE", "RESET TYPE II", "PROBE CURRENT FC#1", "PROBE CURRENT FC#2", "VACUUM ", "CHECK 150V", "INITIALISE PI MOTORS", "SET STIGMATOR", "SET WOBBLER FOR OBJECT", "SHIFT OBJECT APERTURE", "STORE OBJECT POSITION", "STORE APERTURE POSITION", "SHIFT MASS APERTURE", "DEFINE NEW APERTURE", "MOVE TO OBJECT", "MOVE TO APERTURE", "STOP SYSTEM", "TEST COMMANDS"]
            n270 = local write "GATE VALVE"(FALSE ("GATE VALVE")) -> ()
            n271 = for {
              shift-right: [w490] -> w487
              shift-left: w488 -> [w491]
              tunnel: w486 -> [w489] mode=indexing
              n272 = Enqueue Element(queue=w491, element=w489) -> (queue out=w490:refnum<queue>)  [unwired: 2 in, 2 out]
            }
            n273 = One Button Dialog(message="FIB Low Vacuum !") -> ()  [unwired: 1 in, 1 out]
          }
          frame True {
          }
        }
        n274 = local write "SERIAL \nRESPONSE"(w424) -> ()
      }
      frame "RESET TYPE II" {
        n275 = local read "APPEND"() -> (w506:string)
        n276 = local read "VISA ERROR"() -> (w509:errorcluster)
        n277 = local read "ORSAY"() -> (w510:refnum<visa-resource-name>)
        n278 = Concatenate Strings("RE 2", w506) -> (w516:string)
        n279 = VISA Write(VISA resource name=w510, write buffer=w516, error in (no error)=w509) -> (VISA resource name out=w520:refnum<visa-resource-name>, error out=w517:errorcluster)  [unwired: 1 out]
        n280 = flat-sequence {
          tunnel: [w528] -> w519
          tunnel: w520 -> [w528]
          tunnel: [w527] -> w518
          tunnel: w517 -> [w527]
          frame #0 {
            n281 = Wait (ms)(milliseconds to wait=u32 200) -> ()  [unwired: 1 out]
          }
        }
        n282 = Build Array (concatenate)(w515, "RESET TYPE II") -> (w513:string[])
        n283 = property class="Instr"(reference=w519, error in=w518) -> (reference out=w523:refnum<visa-resource-name>, error out=w522:errorcluster, "Serial Settings:Number of Bytes at Serial Port"=w521:u32)
        n284 = local write "PROCESSES"(w513) -> ()
        n285 = VISA Read(VISA resource name=w523, byte count=w521, error in (no error)=w522) -> (VISA resource name out=w508:refnum<visa-resource-name>, read buffer=w512:string, error out=w507:errorcluster)  [unwired: 1 out]
        n286 = Build Array (concatenate)(w511, w512) -> (w505:string[])
        n287 = local write "SERIAL \nRESPONSE"(w505) -> ()
        n288 = local write "ORSAY"(w508) -> ()
        n289 = local write "VISA ERROR"(w507) -> ()
      }
      frame "CHECK 150V" {
        # "Should be true for 150V OK"
        # "NOT COMPLETE!!"
        n290 = local read "APPEND"() -> (w531:string)
        n291 = local read "ORSAY"() -> (w555:refnum<visa-resource-name>)
        n292 = Concatenate Strings("GV 15", w531) -> (w544:string)
        n293 = local read "VISA ERROR"() -> (w554:errorcluster)
        n294 = VISA Write(VISA resource name=w555, write buffer=w544, error in (no error)=w554) -> (VISA resource name out=w542:refnum<visa-resource-name>, error out=w540:errorcluster)  [unwired: 1 out]
        n295 = flat-sequence {
          tunnel: [w565] -> w543
          tunnel: w542 -> [w565]
          tunnel: [w564] -> w541
          tunnel: w540 -> [w564]
          frame #0 {
            n296 = Wait (ms)(milliseconds to wait=u32 50) -> ()  [unwired: 1 out]
          }
        }
        n297 = property class="Instr"(reference=w543, error in=w541) -> (reference out=w550:refnum<visa-resource-name>, error out=w548:errorcluster, "Serial Settings:Number of Bytes at Serial Port"=w549:u32)
        n298 = Build Array (concatenate)(w534, "150V CHECK") -> (w533:string[])
        n299 = VISA Read(VISA resource name=w550, byte count=w549, error in (no error)=w548) -> (VISA resource name out=w553:refnum<visa-resource-name>, read buffer=w536:string, error out=w552:errorcluster)  [unwired: 1 out]
        n300 = local write "VISA ERROR"(w552) -> ()
        n301 = local write "PROCESSES"(w533) -> ()
        n302 = local write "ORSAY"(w553) -> ()
        n303 = call <vilib>:"Trim Whitespace.vi"("string"=w536) -> ("trimmed string"=w539:string)  [unwired: 1 in]
        n304 = Match Pattern(string=w539, regular expression=",") -> (after substring=w538:string)  [unwired: 1 in, 3 out]
        n305 = Build Array (concatenate)(w532, w536) -> (w529:string[])
        n306 = Hexadecimal String To Number(string=w538, default (0uL)=i16 0 ("constante")) -> (number=w547:i16)  [unwired: 1 in, 1 out]
        n307 = local write "SERIAL \nRESPONSE"(w529) -> ()
        n308 = Compound Arithmetic op=AND(w547, 64 ("constante")) -> (w560:i32)
        n309 = Compound Arithmetic op=AND(w547, 16 ("constante")) -> (w561:i32)
        n310 = Not Equal To 0?(x=w560) -> (x != 0?=w558:bool)
        n311 = Not Equal To 0?(x=w561) -> (x != 0?=w546:bool)
        n312 = Or(x=w558, y=w546) -> (x .or. y?=w537:bool)
        "150V GOOD" <- w537
        n313 = case shown="True" w537 {
          tunnel: ["150V INTERLOCKED!" ""] -> w551
          frame False {
          }
          frame True {
          }
        }
        n314 = local write "WARNING"(w551) -> ()
      }
      frame "PROBE CURRENT FC#1" {
        w577 = "MEASURE PROBE CURRENT #1"
        w610 = i16 2
        w604 = i16 2
        n315 = local read "VISA ERROR"() -> (w591:errorcluster)
        n316 = local read "ORSAY"() -> (w598:refnum<visa-resource-name>)
        n317 = local read "APPEND"() -> (w573:string)
        n318 = Concatenate Strings("GV 9", w573) -> (w576:string)
        n319 = VISA Write(VISA resource name=w598, write buffer=w576, error in (no error)=w591) -> (VISA resource name out=w589:refnum<visa-resource-name>, error out=w586:errorcluster)  [unwired: 1 out]
        n320 = flat-sequence {
          tunnel: [w628] -> w588
          tunnel: w589 -> [w628]
          tunnel: [w627] -> w587
          tunnel: w586 -> [w627]
          frame #0 {
            n321 = Wait (ms)(milliseconds to wait=u32 200) -> ()  [unwired: 1 out]
          }
        }
        n322 = property class="Instr"(reference=w588, error in=w587) -> (reference out=w603:refnum<visa-resource-name>, error out=w595:errorcluster, "Serial Settings:Number of Bytes at Serial Port"=w602:u32)
        n323 = local read "APPEND"() -> (w571:string)
        n324 = VISA Read(VISA resource name=w603, byte count=w602, error in (no error)=w595) -> (VISA resource name out=w597:refnum<visa-resource-name>, read buffer=w601:string, error out=w596:errorcluster)  [unwired: 1 out]
        n325 = Match Pattern(string=w601, regular expression=",") -> (before substring=w613:string)  [unwired: 1 in, 3 out]
        n326 = Concatenate Strings("GV 8", w571) -> (w574:string)
        n327 = Hexadecimal String To Number(string=w613, offset=w604, default (0uL)=w604) -> (number=w620:i16)  [unwired: 1 out]
        n328 = VISA Write(VISA resource name=w597, write buffer=w574, error in (no error)=w596) -> (VISA resource name out=w585:refnum<visa-resource-name>, error out=w583:errorcluster)  [unwired: 1 out]
        n329 = Divide(x=w620, y=i16 32767) -> (x/y=w614:dbl)
        n330 = Build Array (concatenate)(w578, w577) -> (w579:string[])
        n331 = Less?(x=w620, y=i16 1600) -> (x < y?=w618:bool)
        "gamme" <- w618
        n332 = Multiply(x=w614, y=sgl 21.28) -> (x*y=w615:dbl)
        n333 = local write "PROCESS"(w577) -> ()
        n334 = flat-sequence {
          tunnel: [w625] -> w584
          tunnel: w585 -> [w625]
          tunnel: [w624] -> w582
          tunnel: w583 -> [w624]
          frame #0 {
            n335 = Wait (ms)(milliseconds to wait=u32 100) -> ()  [unwired: 1 out]
          }
        }
        n336 = property class="Instr"(reference=w584, error in=w582) -> (reference out=w600:refnum<visa-resource-name>, error out=w594:errorcluster, "Serial Settings:Number of Bytes at Serial Port"=w599:u32)
        n337 = VISA Read(VISA resource name=w600, byte count=w599, error in (no error)=w594) -> (VISA resource name out=w593:refnum<visa-resource-name>, read buffer=w581:string, error out=w592:errorcluster)  [unwired: 1 out]
        n338 = Match Pattern(string=w581, regular expression=",") -> (before substring=w619:string)  [unwired: 1 in, 3 out]
        n339 = Hexadecimal String To Number(string=w619, offset=w610, default (0uL)=w610) -> (number=w622:i16)  [unwired: 1 out]
        n340 = Negate(x=w622) -> (-x=w621:i16)
        n341 = Divide(x=w621, y=i16 32767) -> (x/y=w616:dbl)
        n342 = Multiply(x=w616, y=sgl 1060.0) -> (x*y=w617:dbl)
        n343 = case shown="True" w618 {
          tunnel: w615 -> [w629 _]
          tunnel: w617 -> [_ w630]
          tunnel: [w629 w630] -> w590
          frame False {
            (unwired) "Probe current (nA)" ("Définir l'attribut")
          }
          frame True {
            (unwired) "Probe current (pA)" ("Définir l'attribut")
          }
        }
        n344 = node(w590) -> (w569:dbl[unit])
        n345 = Build Array (concatenate)(w580, w581) -> (w568:string[])
        n346 = local write "SERIAL \nRESPONSE"(w568) -> ()
        n347 = local write "BEAM CURRENT (FC1)"(w569) -> ()
        n348 = local write "ORSAY"(w593) -> ()
        n349 = local write "VISA ERROR"(w592) -> ()
      }
      frame "PROBE CURRENT FC#2" {
      }
      frame "CONDENSOR LENS" {
        w641 = u16 3 items=["BEAM ENERGY", "EXTRACTOR", "SUPPRESSOR", "CONDENSOR", "OBJECTIVE"] ("HV SUPPLY")
        w646 = "CONDENSOR LENS"
        n350 = local read "CONDENSOR"() -> (w649:cluster{"COARSE":sgl[unit], "FINE":sgl[unit]})
        n351 = Unbundle By Name(w649) -> ("COARSE"=w640:sgl[unit], "FINE"=w639:sgl[unit])
        n352 = local read "VISA ERROR"() -> (w643:errorcluster)
        n353 = local read "ORSAY"() -> (w644:refnum<visa-resource-name>)
        n354 = Add(x=w640, y=w639) -> (x+y=w634:sgl[unit])
        n355 = local read "TIMER"() -> (w636:u32)
        n356 = local write "PROCESS"(w646) -> ()
        n357 = local read "APPEND"() -> (w642:string)
        n358 = call "SET HV SUPPLY MEASURE IV.vi"("ORSAY"=w644, "SETTLE"=w636, "HV SUPPLY"=w641, "VOLTAGE"=w634, "ORSAY ERROR"=w643, "APPEND"=w642) -> ("ORSAY 2"=w638:refnum<visa-resource-name>, "ORSAY ERROR"=w637:errorcluster)  [unwired: 8 in]
        n359 = Build Array (concatenate)(w647, w646) -> (w648:string[])
        n360 = local write "ORSAY"(w638) -> ()
        n361 = local write "VISA ERROR"(w637) -> ()
      }
      frame "SHUTDOWN ION SOURCE" {
        w653 = FALSE ("TURN ON FILAMENT")
        n362 = local write "FILAMENT HEATING"(dbl[unit] 0.0 ("FILAMENT HEATING")) -> ()
        n363 = local write "ION GUN"(w653) -> ()
        n364 = local write "FILAMENT"(w653) -> ()
        n365 = local write "ION GUN SETTINGS"(T22 {"BEAM ENERGY"=0.0, "EXTRACTOR"=0.0, "SUPPRESSOR"=0.0, "ION CURRENT"=0.0} ("ION GUN SETTINGS")) -> ()
      }
      frame "TURN ON HEATER" {
        w661 = "TURN ON HEATER"
        n366 = local read "FILAMENT"() -> (w656:bool)
        n367 = case shown="True" w656 {
          tunnel: ["SH 0,0" w685] -> w659
          frame False {
          }
          frame True {
            n368 = local read "FILAMENT HEATING"() -> (w680:dbl[unit])
            n369 = node(w680) -> (w678:dbl)
            n370 = call "conversion data to bits.vi"("Data input"=w678, "15 /16b"=TRUE, "Max supply"=sgl 5.0) -> ("15 bits output"=w682:u16)  [unwired: 1 out]
            n371 = Number To Hexadecimal String(2:w682) -> (0:w683:string)  [unwired: 1 in]
            n372 = Concatenate Strings("SH ", w683, ",1" ("string")) -> (w685:string)
          }
        }
        n373 = local read "VISA ERROR"() -> (w666:errorcluster)
        n374 = local read "ORSAY"() -> (w667:refnum<visa-resource-name>)
        n375 = VISA Write(VISA resource name=w667, write buffer=w659, error in (no error)=w666) -> (VISA resource name out=w673:refnum<visa-resource-name>, error out=w670:errorcluster)  [unwired: 1 out]
        n376 = flat-sequence {
          tunnel: [w689] -> w672
          tunnel: w673 -> [w689]
          tunnel: [w688] -> w671
          tunnel: w670 -> [w688]
          frame #0 {
            n377 = Wait (ms)(milliseconds to wait=u32 200) -> ()  [unwired: 1 out]
          }
        }
        n378 = property class="Instr"(reference=w672, error in=w671) -> (reference out=w676:refnum<visa-resource-name>, error out=w675:errorcluster, "Serial Settings:Number of Bytes at Serial Port"=w674:u32)
        n379 = VISA Read(VISA resource name=w676, byte count=w674, error in (no error)=w675) -> (VISA resource name out=w669:refnum<visa-resource-name>, read buffer=w665:string, error out=w668:errorcluster)  [unwired: 1 out]
        n380 = local write "ORSAY"(w669) -> ()
        n381 = local write "VISA ERROR"(w668) -> ()
        n382 = local write "PROCESS"(w661) -> ()
        n383 = Build Array (concatenate)(w663, w661) -> (w660:string[])
        n384 = local write "PROCESSES"(w660) -> ()
        n385 = property on="FILAMENT HEATING" class="Slide (strict)"("DisabledEnum"=T21."Enabled" ("Disabled")) -> ()  [unwired: 2 in, 2 out]
        n386 = Build Array (concatenate)(w662, w665) -> (w657:string[])
        n387 = local write "SERIAL \nRESPONSE"(w657) -> ()
      }
      frame "MEASURE HEATER OUTPUT" {
        w710 = T29 0 items=["both", "start of string", "end of string"] ("location (both)")
        w719 = T29 0 items=["both", "start of string", "end of string"] ("location (both)")
        # "SH, 0, 3.8e-4,0,0,0.71e-3"
        n388 = local read "VISA ERROR"() -> (w733:errorcluster)
        n389 = local read "APPEND"() -> (w736:string)
        n390 = local read "ORSAY"() -> (w734:refnum<visa-resource-name>)
        n391 = Concatenate Strings("GV 18" ("string"), w736) -> (w749:string)
        n392 = VISA Write(VISA resource name=w734, write buffer=w749, error in (no error)=w733) -> (VISA resource name out=w753:refnum<visa-resource-name>, error out=w752:errorcluster)  [unwired: 1 out]
        n393 = flat-sequence {
          tunnel: [w764] -> w751
          tunnel: w753 -> [w764]
          tunnel: [w763] -> w750
          tunnel: w752 -> [w763]
          frame #0 {
            n394 = Wait (ms)(milliseconds to wait=u32 100) -> ()  [unwired: 1 out]
          }
        }
        n395 = property class="Instr"(reference=w751, error in=w750) -> (reference out=w756:refnum<visa-resource-name>, error out=w755:errorcluster, "Serial Settings:Number of Bytes at Serial Port"=w754:u32)
        n396 = VISA Read(VISA resource name=w756, byte count=w754, error in (no error)=w755) -> (VISA resource name out=w738:refnum<visa-resource-name>, read buffer=w712:string, error out=w737:errorcluster)  [unwired: 1 out]
        n397 = call <vilib>:"Trim Whitespace.vi"("string"=w712, "location (both)"=w719) -> ("trimmed string"=w718:string)
        n398 = Match Pattern(string=w718, regular expression="FIB>") -> (before substring=w716:string)  [unwired: 1 in, 3 out]
        n399 = Match Pattern(string=w716, regular expression=",") -> (before substring=w713:string)  [unwired: 1 in, 3 out]
        n400 = Hexadecimal String To Number(string=w713, default (0uL)=u16 0 ("default (0 U32)")) -> (number=w711:u16)  [unwired: 1 in, 1 out]
        n401 = To Double Precision Float(number=w711) -> (double precision float=w723:dbl)
        n402 = Multiply(x=w723, y="IGAIN") -> (x*y=w729:dbl)
        n403 = Add(x=w729, y="IOFFSET") -> (x+y=w701:dbl)
        n404 = local read "APPEND"() -> (w735:string)
        n405 = node(w701) -> (w696:dbl[unit])
        "CURRENT" <- w696
        n406 = Concatenate Strings("GV 19" ("string"), w735) -> (w741:string)
        n407 = VISA Write(VISA resource name=w738, write buffer=w741, error in (no error)=w737) -> (VISA resource name out=w745:refnum<visa-resource-name>, error out=w744:errorcluster)  [unwired: 1 out]
        n408 = feedback #1() -> (w692:i32)
        n409 = Increment(x=w692) -> (x+1=w693:i32)
        n410 = feedback-in #1(w693) -> ()
        n411 = flat-sequence {
          tunnel: [w761] -> w743
          tunnel: w745 -> [w761]
          tunnel: [w760] -> w742
          tunnel: w744 -> [w760]
          frame #0 {
            n412 = Wait (ms)(milliseconds to wait=u32 100) -> ()  [unwired: 1 out]
          }
        }
        n413 = Build Array (concatenate)(w722, "MEASURE HEATER OUTPUT") -> (w721:string[])
        n414 = feedback #2() -> (w699:i32[])
        n415 = Build Array (concatenate)(w699, w693) -> (w691:i32[])
        n416 = feedback-in #2(w691) -> ()
        n417 = feedback #3() -> (w697:dbl[unit][])
        n418 = property class="Instr"(reference=w743, error in=w742) -> (reference out=w748:refnum<visa-resource-name>, error out=w747:errorcluster, "Serial Settings:Number of Bytes at Serial Port"=w746:u32)
        n419 = VISA Read(VISA resource name=w748, byte count=w746, error in (no error)=w747) -> (VISA resource name out=w732:refnum<visa-resource-name>, read buffer=w705:string, error out=w731:errorcluster)  [unwired: 1 out]
        n420 = call <vilib>:"Trim Whitespace.vi"("string"=w705, "location (both)"=w710) -> ("trimmed string"=w709:string)
        n421 = Match Pattern(string=w709, regular expression="FIB>") -> (before substring=w707:string)  [unwired: 1 in, 3 out]
        n422 = local write "ORSAY"(w732) -> ()
        n423 = local write "VISA ERROR"(w731) -> ()
        n424 = Match Pattern(string=w707, regular expression=",") -> (before substring=w703:string)  [unwired: 1 in, 3 out]
        n425 = Hexadecimal String To Number(string=w703, default (0uL)=u16 0 ("default (0 U32)")) -> (number=w702:u16)  [unwired: 1 in, 1 out]
        n426 = To Double Precision Float(number=w702) -> (double precision float=w724:dbl)
        n427 = Multiply(x="VGAIN", y=w724) -> (x*y=w725:dbl)
        n428 = Add(x="VOFFSET", y=w725) -> (x+y=w700:dbl)
        n429 = node(w700) -> (w695:dbl[unit])
        "VOLTAGE" <- w695
        n430 = Multiply(x=w696, y=w695) -> (x*y=w698:dbl[unit])
        n431 = Build Array (concatenate)(w697, w698) -> (w694:dbl[unit][])
        n432 = feedback-in #3(w694) -> ()
        n433 = Bundle(w691, w694) -> (→"HEAT POWER":cluster{i32[], dbl[unit][]})  [unwired: 1 in]
      }
      frame "TOGGLE GATE VALVE" {
        n434 = local read "GATE VALVE"() -> (w773:bool)
        n435 = case shown="True" w773 {
          tunnel: ["1" "0"] -> w772
          tunnel: ["OPENING GATE VALVE" "CLOSING GATE VALVE"] -> w771
          frame False {
          }
          frame True {
          }
        }
        n436 = local read "VISA ERROR"() -> (w783:errorcluster)
        n437 = local read "ORSAY"() -> (w782:refnum<visa-resource-name>)
        n438 = local read "APPEND"() -> (w767:string)
        n439 = Concatenate Strings("VC ", w772, w767) -> (w784:string)
        n440 = VISA Write(VISA resource name=w782, write buffer=w784, error in (no error)=w783) -> (VISA resource name out=w778:refnum<visa-resource-name>, error out=w781:errorcluster)  [unwired: 1 out]
        n441 = flat-sequence {
          tunnel: [w794] -> w779
          tunnel: w778 -> [w794]
          tunnel: [w793] -> w780
          tunnel: w781 -> [w793]
          frame #0 {
            n442 = Wait (ms)(milliseconds to wait=u32 200) -> ()  [unwired: 1 out]
          }
        }
        n443 = Build Array (concatenate)(w770, w771) -> (w769:string[])
        n444 = local write "PROCESSES"(w769) -> ()
        n445 = property class="Instr"(reference=w779, error in=w780) -> (reference out=w775:refnum<visa-resource-name>, error out=w776:errorcluster, "Serial Settings:Number of Bytes at Serial Port"=w777:u32)
        n446 = VISA Read(VISA resource name=w775, byte count=w777, error in (no error)=w776) -> (VISA resource name out=w785:refnum<visa-resource-name>, read buffer=w787:string, error out=w786:errorcluster)  [unwired: 1 out]
        n447 = local write "ORSAY"(w785) -> ()
        n448 = local write "VISA ERROR"(w786) -> ()
        n449 = Build Array (concatenate)(w768, w787) -> (w765:string[])
        n450 = local write "SERIAL \nRESPONSE"(w765) -> ()
      }
      frame "OBJECTIVE LENS" {
        w799 = "OBJECTIVE LENS"
        n451 = local read "OBJECTIVE"() -> (w822:cluster{"COARSE":sgl[unit], "FINE":sgl[unit]})
        n452 = Unbundle By Name(w822) -> ("COARSE"=w817:sgl[unit], "FINE"=w816:sgl[unit])
        n453 = node(w817) -> (w814:sgl)
        n454 = node(w816) -> (w815:sgl)
        n455 = Add(x=w814, y=w815) -> (x+y=w813:sgl)
        n456 = local read "VISA ERROR"() -> (w809:errorcluster)
        n457 = call "conversion data to bits.vi"("Data input"=w813, "Max supply"=sgl 20000.0) -> ("15 bits output"=w819:u16)  [unwired: 1 in, 1 out]
        n458 = local write "PROCESS"(w799) -> ()
        n459 = local read "ORSAY"() -> (w824:refnum<visa-resource-name>)
        n460 = Number To Hexadecimal String(2:w819) -> (0:w818:string)  [unwired: 1 in]
        n461 = local read "APPEND"() -> (w797:string)
        n462 = Concatenate Strings("L2 ", w818, w797) -> (w798:string)
        n463 = Build Array (concatenate)(w801, w799) -> (w800:string[])
        n464 = VISA Write(VISA resource name=w824, write buffer=w798, error in (no error)=w809) -> (VISA resource name out=w808:refnum<visa-resource-name>, error out=w807:errorcluster)  [unwired: 1 out]
        n465 = flat-sequence {
          tunnel: [w827] -> w806
          tunnel: w808 -> [w827]
          tunnel: [w826] -> w805
          tunnel: w807 -> [w826]
          frame #0 {
            n466 = Wait (ms)(milliseconds to wait=u32 50) -> ()  [unwired: 1 out]
          }
        }
        n467 = local write "PROCESSES"(w800) -> ()
        n468 = property class="Instr"(reference=w806, error in=w805) -> (reference out=w812:refnum<visa-resource-name>, error out=w811:errorcluster, "Serial Settings:Number of Bytes at Serial Port"=w810:u32)
        n469 = VISA Read(VISA resource name=w812, byte count=w810, error in (no error)=w811) -> (VISA resource name out=w823:refnum<visa-resource-name>, read buffer=w803:string, error out=w804:errorcluster)  [unwired: 1 out]
        n470 = local write "ORSAY"(w823) -> ()
        n471 = local write "VISA ERROR"(w804) -> ()
        n472 = Build Array (concatenate)(w802, w803) -> (w795:string[])
        n473 = local write "SERIAL \nRESPONSE"(w795) -> ()
      }
      frame "SET ENERGY RANGE" {
        # "HIGH energy range (MAX 30kV)"
        # "LOW energy range (MAX 10kV)"
        n474 = local read "HIGH ENERGY"() -> (w829:bool)
        n475 = local read "VISA ERROR"() -> (w846:errorcluster)
        n476 = local read "ORSAY"() -> (w847:refnum<visa-resource-name>)
        n477 = Select(t="RE 3", s=w829, f="RE 4") -> (s? t:f=w840:string)
        n478 = VISA Write(VISA resource name=w847, write buffer=w840, error in (no error)=w846) -> (VISA resource name out=w836:refnum<visa-resource-name>, error out=w835:errorcluster)  [unwired: 1 out]
        n479 = flat-sequence {
          tunnel: [w850] -> w833
          tunnel: w836 -> [w850]
          tunnel: [w849] -> w834
          tunnel: w835 -> [w849]
          frame #0 {
            n480 = Wait (ms)(milliseconds to wait=u32 100) -> ()  [unwired: 1 out]
          }
        }
        n481 = property class="Instr"(reference=w833, error in=w834) -> (reference out=w839:refnum<visa-resource-name>, error out=w838:errorcluster, "Serial Settings:Number of Bytes at Serial Port"=w837:u32)
        n482 = VISA Read(VISA resource name=w839, byte count=w837, error in (no error)=w838) -> (VISA resource name out=w845:refnum<visa-resource-name>, read buffer=w832:string, error out=w844:errorcluster)  [unwired: 1 out]
        n483 = Build Array (concatenate)(w843, w832) -> (w828:string[])
        n484 = local write "SERIAL \nRESPONSE"(w828) -> ()
        n485 = local write "VISA ERROR"(w844) -> ()
        n486 = local write "ORSAY"(w845) -> ()
      }
      frame "TURN ON BEAM HV" {
        w851 = "RAMPING UP/DOWN ION GUN PARAMETERS" ("PROCESS")
        n487 = flat-sequence {
          tunnel: [w860] -> w854
          tunnel: [w859] -> w852
          tunnel: w858 -> [w866]
          tunnel: [w865] -> w857
          tunnel: w854 -> [w861]
          tunnel: w852 -> [w863]
          frame #0 {
            n488 = local read "PREVIOUS GUN SETTINGS"() -> (w859:T2)
            n489 = local read "ION GUN SETTINGS"() -> (w860:T2)
          }
          frame #1 {
            # "New settings"
            n490 = Unbundle By Name(w863) -> ("BEAM ENERGY"=w862:sgl[unit])  [unwired: 3 out]
            n491 = Unbundle By Name(w861) -> ("BEAM ENERGY"=w864:sgl[unit])
            n492 = local write "PREVIOUS GUN SETTINGS"(w861) -> ()
            n493 = stacked-sequence {
              tunnel: w864 -> [w877 _ _]
              tunnel: w866 -> [_ w897 _]
              tunnel: w862 -> [w867 _ _]
              tunnel: [_ w897 _] -> w865
              frame #0 {
                n494 = Subtract(x=w877, y=w867) -> (x-y=w874:sgl[unit])
                n495 = node(w874) -> (w873:sgl)
                n496 = Greater Than 0?(x=w873) -> (x > 0?=w875:bool)
                n497 = case shown="False" w875 {
                  tunnel: [w880 w882] -> w869
                  tunnel: "dV ENERGY" -> [w881 w882]
                  frame False {
                    n498 = Negate(x=w881) -> (-x=w880:dbl[unit])
                  }
                  frame True {
                  }
                }
                n499 = Absolute Value(x=w874) -> (abs(x)=w876:sgl[unit])
                n500 = Divide(x=w876, y=w869) -> (x/y=w879:dbl)
                n501 = Absolute Value(x=w879) -> (abs(x)=w868:dbl)
                n502 = To Long Integer(number=w868) -> (32bit integer=w878:i32)
                n503 = for {
                  N: w878 -> [_]
                  tunnel: w869 -> [w886]
                  tunnel: [w883] -> w870 mode=indexing
                  tunnel: w867 -> [w884]
                  i -> [w888]
                  n504 = Increment(x=w888) -> (x+1=w887:i32)
                  n505 = Multiply(x=w886, y=w887) -> (x*y=w885:dbl[unit])
                  n506 = Add(x=w884, y=w885) -> (x+y=w883:dbl[unit])
                }
                "BEAM RAMP" <- w870
                n507 = local write "BEAM RAMP"(w870) -> ()
                n508 = Array Size(array=w870) -> (size(s)=→"size(s)":i32)
              }
              frame #1 {
                n509 = local read "BEAM RAMP"() -> (w890:dbl[unit][])
                n510 = Array Size(array=w890) -> (size(s)=w889:i32)
                n511 = local read "VISA ERROR"() -> (w895:errorcluster)
                n512 = local read "ORSAY"() -> (w896:refnum<visa-resource-name>)
                n513 = local read "TIMER"() -> (w894:u32)
                n514 = Not Equal To 0?(x=w889) -> (x != 0?=w891:bool)
                n515 = case shown="True" w891 {
                  tunnel: w896 -> [w899 w905]
                  tunnel: w895 -> [w898 w904]
                  tunnel: w894 -> [_ w903]
                  tunnel: [w899 w902] -> w893
                  tunnel: w890 -> [_ w900]
                  tunnel: [w898 w901] -> w892
                  frame False {
                  }
                  frame True {
                    n516 = for {
                      shift-right: [w920] -> w902
                      shift-left: w905 -> [w929]
                      shift-right: [w917] -> w901
                      shift-left: w904 -> [w928]
                      tunnel: w903 -> [w927]
                      tunnel: w900 -> [w924] mode=indexing
                      w915 = u16 2 items=["BEAM ENERGY", "EXTRACTOR", "SUPPRESSOR", "CONDENSOR", "OBJECTIVE"] ("HV SUPPLY")
                      w916 = u16 1 items=["BEAM ENERGY", "EXTRACTOR", "SUPPRESSOR", "CONDENSOR", "OBJECTIVE"] ("HV SUPPLY")
                      w923 = u16 0 items=["BEAM ENERGY", "EXTRACTOR", "SUPPRESSOR", "CONDENSOR", "OBJECTIVE"] ("HV SUPPLY")
                      n517 = local read "APPEND"() -> (w912:string)
                      n518 = call "SET HV SUPPLY MEASURE IV.vi"("ORSAY"=w929, "SETTLE"=w927, "HV SUPPLY"=w923, "VOLTAGE"=w924, "ORSAY ERROR"=w928, "APPEND"=w912) -> ("ORSAY 2"=w926:refnum<visa-resource-name>, "ORSAY ERROR"=w925:errorcluster)  [unwired: 8 in]
                      n519 = call "READ HV SUPPLIES.vi"("ORSAY"=w926, "HV SUPPLY"=w923, "ORSAY ERROR"=w925, "APPEND"=w912) -> ("ORSAY 2"=w922:refnum<visa-resource-name>, "VOLTAGE"=w907:dbl[unit], "CURRENT"=w906:dbl[unit], "ORSAY ERROR"=w919:errorcluster)  [unwired: 8 in]
                      n520 = local write "CURRENT"(w906) -> ()
                      n521 = local write "VOLTAGE"(w907) -> ()
                      n522 = local write "BEAM VOLTAGE"(w907) -> ()
                      n523 = local write "BEAM CURRENT"(w906) -> ()
                      n524 = call "READ HV SUPPLIES.vi"("ORSAY"=w922, "HV SUPPLY"=w916, "ORSAY ERROR"=w919, "APPEND"=w912) -> ("ORSAY 2"=w921:refnum<visa-resource-name>, "VOLTAGE"=w909:dbl[unit], "CURRENT"=w914:dbl[unit], "ORSAY ERROR"=w918:errorcluster)  [unwired: 8 in]
                      n525 = call "READ HV SUPPLIES.vi"("ORSAY"=w921, "HV SUPPLY"=w915, "ORSAY ERROR"=w918, "APPEND"=w912) -> ("ORSAY 2"=w920:refnum<visa-resource-name>, "VOLTAGE"=w910:dbl[unit], "CURRENT"=w913:dbl[unit], "ORSAY ERROR"=w917:errorcluster)  [unwired: 8 in]
                      n526 = Bundle By Name(cluster=T24 {"BEAM"=0.0, "SUPPRESSOR"=0.0, "EXTRACTOR"=0.0} ("HIGH VOLTAGE SUPPLIES"), "BEAM"=w907, "SUPPRESSOR"=w910, "EXTRACTOR"=w909) -> (w911:T24)
                      n527 = local write "HIGH VOLTAGE SUPPLIES"(w911) -> ()
                      n528 = local write "EXTRACTOR  CURRENT"(w914) -> ()
                      n529 = local write "EXTRACTOR"(w909) -> ()
                      n530 = local write "SUPPRESSOR CURRENT"(w913) -> ()
                      n531 = local write "SUPPRESSOR VOLTAGE"(w910) -> ()
                    }
                  }
                }
                n532 = local write "VISA ERROR"(w892) -> ()
                n533 = local write "ORSAY"(w893) -> ()
              }
              frame #2 {
                n534 = property on="SUPPRESSOR" class="Slide (strict)"("DisabledEnum"=T21."Enabled" ("Disabled")) -> ()  [unwired: 2 in, 2 out]
              }
            }
          }
        }
        n535 = local write "PROCESS"(w851) -> ()
        n536 = Build Array (concatenate)(w856, w851) -> (w855:string[])
        n537 = local write "PROCESSES"(w855) -> ()
      }
      frame "ENERGY RAMP CYCLE" {
        n538 = while {
          tunnel: dbl[unit][] [500.0, 1000.0, 1500.0, 2000.0, 2500.0, 3000.0, 3500.0, 4000.0, 4500.0, 5000.0, 4500.0, 4000.0, 3500.0, 3000.0, 2500.0, 2000.0, 1500.0, 1000.0, 500.0, 0.0] -> [w937]
          stop <- w935 continue-if-true
          n539 = local read "VISA ERROR"() -> (w941:errorcluster)
          n540 = local read "TIMER"() -> (w938:u32)
          n541 = local read "ORSAY"() -> (w942:refnum<visa-resource-name>)
          n542 = Array Size(array=w937) -> (size(s)=w936:i32)
          n543 = for {
            N: w936 -> [_]
            shift-right: [w947] -> w940
            shift-left: w942 -> [w954]
            shift-right: [w945] -> w939
            shift-left: w941 -> [w953]
            tunnel: w938 -> [w952]
            tunnel: w937 -> [w943] mode=indexing
            w948 = u16 0 items=["BEAM ENERGY", "EXTRACTOR", "SUPPRESSOR", "CONDENSOR", "OBJECTIVE"] ("HV SUPPLY")
            n544 = local read "APPEND"() -> (w949:string)
            n545 = call "SET HV SUPPLY MEASURE IV.vi"("ORSAY"=w954, "SETTLE"=w952, "HV SUPPLY"=w948, "VOLTAGE"=w943, "ORSAY ERROR"=w953, "APPEND"=w949) -> ("ORSAY 2"=w951:refnum<visa-resource-name>, "ORSAY ERROR"=w950:errorcluster)  [unwired: 8 in]
            n546 = call "READ HV SUPPLIES.vi"("ORSAY"=w951, "HV SUPPLY"=w948, "ORSAY ERROR"=w950, "APPEND"=w949) -> ("ORSAY 2"=w946:refnum<visa-resource-name>, "ORSAY ERROR"=w944:errorcluster)  [unwired: 8 in, 2 out]
            n547 = flat-sequence {
              tunnel: [w956] -> w947
              tunnel: w946 -> [w956]
              tunnel: [w955] -> w945
              tunnel: w944 -> [w955]
              frame #0 {
                n548 = Wait (ms)(milliseconds to wait=u32 100) -> ()  [unwired: 1 out]
              }
            }
          }
          n549 = local read "1V ENERGY RAMP"() -> (w935:bool)
          n550 = local write "ORSAY"(w940) -> ()
          n551 = local write "VISA ERROR"(w939) -> ()
        }
      }
      frame "TURN ON SUPPRESSOR" {
        w959 = "RAMPING UP/DOWN SUPPRESSOR" ("PROCESS")
        n552 = flat-sequence {
          tunnel: [w967] -> w961
          tunnel: [w966] -> w958
          tunnel: w965 -> [w973]
          tunnel: [w972] -> w964
          tunnel: w961 -> [w969]
          tunnel: w958 -> [w970]
          frame #0 {
            n553 = local read "PREVIOUS GUN SETTINGS"() -> (w966:T2)
            n554 = local read "ION GUN SETTINGS"() -> (w967:T2)
          }
          frame #1 {
            # "New settings"
            n555 = Unbundle By Name(w970) -> ("SUPPRESSOR"=w968:sgl[unit])  [unwired: 3 out]
            n556 = local write "PREVIOUS GUN SETTINGS"(w969) -> ()
            n557 = Unbundle By Name(w969) -> ("SUPPRESSOR"=w971:sgl[unit])
            n558 = stacked-sequence {
              tunnel: w971 -> [w976 _ _]
              tunnel: w973 -> [_ w1004 _]
              tunnel: w968 -> [w974 _ _]
              tunnel: [_ w1004 _] -> w972
              frame #0 {
                # "S-E=Seffective"
                n559 = Subtract(x=w976, y=w974) -> (x-y=w975:sgl[unit])
                n560 = node(w975) -> (w983:sgl)
                n561 = Greater Than 0?(x=w983) -> (x > 0?=w982:bool)
                n562 = case shown="False" w982 {
                  tunnel: [w988 w989] -> w980
                  tunnel: "dV SUPPRESS" -> [w987 w989]
                  frame False {
                    n563 = Negate(x=w987) -> (-x=w988:dbl[unit])
                  }
                  frame True {
                  }
                }
                n564 = Absolute Value(x=w975) -> (abs(x)=w984:sgl[unit])
                n565 = Divide(x=w984, y=w980) -> (x/y=w986:dbl)
                n566 = Absolute Value(x=w986) -> (abs(x)=w979:dbl)
                n567 = To Long Integer(number=w979) -> (32bit integer=w985:i32)
                n568 = for {
                  N: w985 -> [_]
                  tunnel: w980 -> [w994]
                  tunnel: [w992] -> w977 mode=indexing
                  tunnel: w974 -> [w991]
                  i -> [w995]
                  n569 = Increment(x=w995) -> (x+1=w993:i32)
                  n570 = Multiply(x=w994, y=w993) -> (x*y=w990:dbl[unit])
                  n571 = Add(x=w991, y=w990) -> (x+y=w992:dbl[unit])
                }
                "SUPPRESSOR RAMP" <- w977
                n572 = local write "SUPPRESSOR RAMP"(w977) -> ()
                n573 = Array Size(array=w977) -> (size(s)=→"size(s) 4":i32)
              }
              frame #1 {
                n574 = local read "SUPPRESSOR RAMP"() -> (w997:dbl[unit][])
                n575 = Array Size(array=w997) -> (size(s)=w996:i32)
                n576 = local read "VISA ERROR"() -> (w1002:errorcluster)
                n577 = local read "ORSAY"() -> (w1003:refnum<visa-resource-name>)
                n578 = local read "TIMER"() -> (w1001:u32)
                n579 = Not Equal To 0?(x=w996) -> (x != 0?=w998:bool)
                n580 = case shown="True" w998 {
                  tunnel: w1003 -> [w1006 w1012]
                  tunnel: w1002 -> [w1005 w1011]
                  tunnel: w1001 -> [_ w1010]
                  tunnel: [w1006 w1009] -> w1000
                  tunnel: w997 -> [_ w1007]
                  tunnel: [w1005 w1008] -> w999
                  frame False {
                  }
                  frame True {
                    n581 = for {
                      shift-right: [w1022] -> w1009
                      shift-left: w1012 -> [w1036]
                      shift-right: [w1021] -> w1008
                      shift-left: w1011 -> [w1035]
                      tunnel: w1010 -> [w1034]
                      tunnel: w1007 -> [w1031] mode=indexing
                      w1023 = u16 1 items=["BEAM ENERGY", "EXTRACTOR", "SUPPRESSOR", "CONDENSOR", "OBJECTIVE"] ("HV SUPPLY")
                      w1027 = u16 0 items=["BEAM ENERGY", "EXTRACTOR", "SUPPRESSOR", "CONDENSOR", "OBJECTIVE"] ("HV SUPPLY")
                      w1030 = u16 2 items=["BEAM ENERGY", "EXTRACTOR", "SUPPRESSOR", "CONDENSOR", "OBJECTIVE"] ("HV SUPPLY")
                      n582 = local read "APPEND"() -> (w1024:string)
                      n583 = call "SET HV SUPPLY MEASURE IV.vi"("ORSAY"=w1036, "SETTLE"=w1034, "HV SUPPLY"=w1030, "VOLTAGE"=w1031, "ORSAY ERROR"=w1035, "APPEND"=w1024) -> ("ORSAY 2"=w1033:refnum<visa-resource-name>, "ORSAY ERROR"=w1032:errorcluster)  [unwired: 8 in]
                      n584 = call "READ HV SUPPLIES.vi"("ORSAY"=w1033, "HV SUPPLY"=w1030, "ORSAY ERROR"=w1032, "APPEND"=w1024) -> ("ORSAY 2"=w1029:refnum<visa-resource-name>, "VOLTAGE"=w1013:dbl[unit], "CURRENT"=w1014:dbl[unit], "ORSAY ERROR"=w1028:errorcluster)  [unwired: 8 in]
                      n585 = local write "VOLTAGE"(w1013) -> ()
                      n586 = local write "CURRENT"(w1014) -> ()
                      n587 = local write "SUPPRESSOR CURRENT"(w1014) -> ()
                      n588 = local write "SUPPRESSOR VOLTAGE"(w1013) -> ()
                      n589 = call "READ HV SUPPLIES.vi"("ORSAY"=w1029, "HV SUPPLY"=w1027, "ORSAY ERROR"=w1028, "APPEND"=w1024) -> ("ORSAY 2"=w1026:refnum<visa-resource-name>, "VOLTAGE"=w1018:dbl[unit], "CURRENT"=w1020:dbl[unit], "ORSAY ERROR"=w1025:errorcluster)  [unwired: 8 in]
                      n590 = local write "BEAM CURRENT"(w1020) -> ()
                      n591 = local write "BEAM VOLTAGE"(w1018) -> ()
                      n592 = call "READ HV SUPPLIES.vi"("ORSAY"=w1026, "HV SUPPLY"=w1023, "ORSAY ERROR"=w1025, "APPEND"=w1024) -> ("ORSAY 2"=w1022:refnum<visa-resource-name>, "VOLTAGE"=w1016:dbl[unit], "CURRENT"=w1019:dbl[unit], "ORSAY ERROR"=w1021:errorcluster)  [unwired: 8 in]
                      n593 = local write "EXTRACTOR  CURRENT"(w1019) -> ()
                      n594 = local write "EXTRACTOR"(w1016) -> ()
                      n595 = Bundle By Name(cluster=T24 {"BEAM"=0.0, "SUPPRESSOR"=0.0, "EXTRACTOR"=0.0} ("HIGH VOLTAGE SUPPLIES"), "BEAM"=w1018, "SUPPRESSOR"=w1013, "EXTRACTOR"=w1016) -> (w1017:T24)
                      n596 = local write "HIGH VOLTAGE SUPPLIES"(w1017) -> ()
                    }
                  }
                }
                n597 = local write "VISA ERROR"(w999) -> ()
                n598 = local write "ORSAY"(w1000) -> ()
              }
              frame #2 {
                n599 = property on="EXTRACTOR" class="Slide (strict)"("DisabledEnum"=T21."Enabled" ("Disabled")) -> ()  [unwired: 2 in, 2 out]
              }
            }
          }
        }
        n600 = local write "PROCESS"(w959) -> ()
        n601 = Build Array (concatenate)(w963, w959) -> (w962:string[])
        n602 = local write "PROCESSES"(w962) -> ()
      }
      frame "TURN ON EXTRACTOR" {
        w1039 = "RAMPING UP/DOWN SUPPRESSOR" ("PROCESS")
        n603 = flat-sequence {
          tunnel: [w1047] -> w1041
          tunnel: [w1046] -> w1038
          tunnel: w1045 -> [w1053]
          tunnel: [w1052] -> w1044
          tunnel: w1041 -> [w1048]
          tunnel: w1038 -> [w1050]
          frame #0 {
            n604 = local read "PREVIOUS GUN SETTINGS"() -> (w1046:T2)
            n605 = local read "ION GUN SETTINGS"() -> (w1047:T2)
          }
          frame #1 {
            # "New settings"
            n606 = local write "PREVIOUS GUN SETTINGS"(w1048) -> ()
            n607 = Unbundle By Name(w1050) -> ("EXTRACTOR"=w1049:sgl[unit])  [unwired: 3 out]
            n608 = Unbundle By Name(w1048) -> ("EXTRACTOR"=w1051:sgl[unit])
            n609 = stacked-sequence {
              tunnel: w1051 -> [w1055 _ _]
              tunnel: w1053 -> [_ w1084 _]
              tunnel: w1049 -> [w1054 _ _]
              tunnel: [_ w1084 _] -> w1052
              frame #0 {
                n610 = Subtract(x=w1055, y=w1054) -> (x-y=w1061:sgl[unit])
                n611 = node(w1061) -> (w1063:sgl)
                n612 = Greater Than 0?(x=w1063) -> (x > 0?=w1062:bool)
                n613 = case shown="False" w1062 {
                  tunnel: [w1068 w1069] -> w1059
                  tunnel: "dV EXTRACTOR" -> [w1067 w1069]
                  frame False {
                    n614 = Negate(x=w1067) -> (-x=w1068:dbl[unit])
                  }
                  frame True {
                  }
                }
                n615 = Absolute Value(x=w1061) -> (abs(x)=w1064:sgl[unit])
                n616 = Divide(x=w1064, y=w1059) -> (x/y=w1066:dbl)
                n617 = Absolute Value(x=w1066) -> (abs(x)=w1058:dbl)
                n618 = To Long Integer(number=w1058) -> (32bit integer=w1065:i32)
                n619 = for {
                  N: w1065 -> [_]
                  tunnel: w1059 -> [w1074]
                  tunnel: [w1072] -> w1056 mode=indexing
                  tunnel: w1054 -> [w1071]
                  i -> [w1075]
                  n620 = Increment(x=w1075) -> (x+1=w1073:i32)
                  n621 = Multiply(x=w1074, y=w1073) -> (x*y=w1070:dbl[unit])
                  n622 = Add(x=w1071, y=w1070) -> (x+y=w1072:dbl[unit])
                }
                n623 = local write "EXTRACTOR RAMP"(w1056) -> ()
                n624 = local write "EXTRACTOR RAMP"(w1056) -> ()
                n625 = Array Size(array=w1056) -> (size(s)=→"size(s) 5":i32)
              }
              frame #1 {
                n626 = local read "EXTRACTOR RAMP"() -> (w1076:dbl[unit][])
                n627 = Array Size(array=w1076) -> (size(s)=w1077:i32)
                n628 = local read "VISA ERROR"() -> (w1082:errorcluster)
                n629 = local read "ORSAY"() -> (w1083:refnum<visa-resource-name>)
                n630 = local read "TIMER"() -> (w1081:u32)
                n631 = Not Equal To 0?(x=w1077) -> (x != 0?=w1078:bool)
                n632 = case shown="True" w1078 {
                  tunnel: w1083 -> [w1086 w1092]
                  tunnel: w1082 -> [w1085 w1091]
                  tunnel: w1081 -> [_ w1090]
                  tunnel: [w1086 w1089] -> w1080
                  tunnel: w1076 -> [_ w1087]
                  tunnel: [w1085 w1088] -> w1079
                  frame False {
                  }
                  frame True {
                    n633 = for {
                      shift-right: [w1105] -> w1089
                      shift-left: w1092 -> [w1116]
                      shift-right: [w1103] -> w1088
                      shift-left: w1091 -> [w1115]
                      tunnel: w1090 -> [w1114]
                      tunnel: w1087 -> [w1111] mode=indexing
                      w1100 = u16 0 items=["BEAM ENERGY", "EXTRACTOR", "SUPPRESSOR", "CONDENSOR", "OBJECTIVE"] ("HV SUPPLY")
                      w1101 = u16 2 items=["BEAM ENERGY", "EXTRACTOR", "SUPPRESSOR", "CONDENSOR", "OBJECTIVE"] ("HV SUPPLY")
                      w1110 = u16 1 items=["BEAM ENERGY", "EXTRACTOR", "SUPPRESSOR", "CONDENSOR", "OBJECTIVE"] ("HV SUPPLY")
                      n634 = local read "APPEND"() -> (w1102:string)
                      n635 = call "SET HV SUPPLY MEASURE IV.vi"("ORSAY"=w1116, "SETTLE"=w1114, "HV SUPPLY"=w1110, "VOLTAGE"=w1111, "ORSAY ERROR"=w1115, "APPEND"=w1102) -> ("ORSAY 2"=w1113:refnum<visa-resource-name>, "ORSAY ERROR"=w1112:errorcluster)  [unwired: 8 in]
                      n636 = call "READ HV SUPPLIES.vi"("ORSAY"=w1113, "HV SUPPLY"=w1110, "ORSAY ERROR"=w1112, "APPEND"=w1102) -> ("ORSAY 2"=w1108:refnum<visa-resource-name>, "VOLTAGE"=w1096:dbl[unit], "CURRENT"=w1109:dbl[unit], "ORSAY ERROR"=w1107:errorcluster)  [unwired: 8 in]
                      n637 = local write "EXTRACTOR"(w1096) -> ()
                      n638 = local write "EXTRACTOR  CURRENT"(w1109) -> ()
                      n639 = call "READ HV SUPPLIES.vi"("ORSAY"=w1108, "HV SUPPLY"=w1100, "ORSAY ERROR"=w1107, "APPEND"=w1102) -> ("ORSAY 2"=w1106:refnum<visa-resource-name>, "VOLTAGE"=w1093:dbl[unit], "CURRENT"=w1094:dbl[unit], "ORSAY ERROR"=w1104:errorcluster)  [unwired: 8 in]
                      n640 = local write "VOLTAGE"(w1093) -> ()
                      n641 = local write "CURRENT"(w1094) -> ()
                      n642 = local write "BEAM CURRENT"(w1094) -> ()
                      n643 = local write "BEAM VOLTAGE"(w1093) -> ()
                      n644 = call "READ HV SUPPLIES.vi"("ORSAY"=w1106, "HV SUPPLY"=w1101, "ORSAY ERROR"=w1104, "APPEND"=w1102) -> ("ORSAY 2"=w1105:refnum<visa-resource-name>, "VOLTAGE"=w1097:dbl[unit], "CURRENT"=w1099:dbl[unit], "ORSAY ERROR"=w1103:errorcluster)  [unwired: 8 in]
                      n645 = Bundle By Name(cluster=T24 {"BEAM"=0.0, "SUPPRESSOR"=0.0, "EXTRACTOR"=0.0} ("HIGH VOLTAGE SUPPLIES"), "BEAM"=w1093, "SUPPRESSOR"=w1097, "EXTRACTOR"=w1096) -> (w1098:T24)
                      n646 = local write "HIGH VOLTAGE SUPPLIES"(w1098) -> ()
                      n647 = local write "SUPPRESSOR CURRENT"(w1099) -> ()
                      n648 = local write "SUPPRESSOR VOLTAGE"(w1097) -> ()
                    }
                  }
                }
                n649 = local write "VISA ERROR"(w1079) -> ()
                n650 = local write "ORSAY"(w1080) -> ()
              }
              frame #2 {
                n651 = property on="EXTRACTOR" class="Slide (strict)"("DisabledEnum"=T21."Enabled" ("Disabled")) -> ()  [unwired: 2 in, 2 out]
              }
            }
          }
        }
        n652 = local write "PROCESS"(w1039) -> ()
        n653 = Build Array (concatenate)(w1043, w1039) -> (w1042:string[])
        n654 = local write "PROCESSES"(w1042) -> ()
      }
      frame "TURN ON WIEN FILTER" {
        w1142 = 9.999999747378752e-06 ("f")
        w1147 = dbl[unit] 30000.0  # kV
        n655 = local read "ION GUN SETTINGS"() -> (w1149:T2)
        n656 = Unbundle By Name("E&B") -> ("M-COARSE"=w1150:sgl, "M-FINE"=w1151:sgl, "ELECTRIC FIELD"=w1141:sgl)
        n657 = Unbundle By Name(w1149) -> ("BEAM ENERGY"=w1148:sgl[unit])
        n658 = Divide(x=w1148, y=w1147) -> (x/y=w1146:dbl)
        n659 = Square Root(x=w1146) -> (sqrt(x)=w1144:dbl)
        n660 = Add(x=w1150, y=w1151) -> (x+y=w1145:sgl)
        n661 = Multiply(x=w1145, y=w1144) -> (x*y=w1138:dbl)
        n662 = local read "WIEN"() -> (w1143:bool)
        n663 = local read "VISA ERROR"() -> (w1127:errorcluster)
        n664 = Less Than 0?(x=w1138) -> (x < 0?=w1140:bool)
        n665 = local read "ORSAY"() -> (w1128:refnum<visa-resource-name>)
        n666 = case shown="True" w1140 {
          tunnel: [w1161 0.0] -> w1139
          tunnel: w1138 -> [w1161 _]
          frame False {
          }
          frame True {
          }
        }
        n667 = Select(t=w1139, s=w1143, f=w1142) -> (s? t:f=w1134:dbl)
        n668 = Select(t=w1141, s=w1143, f=w1142) -> (s? t:f=w1133:dbl)
        n669 = flat-sequence {
          tunnel: w1157 -> [w1163]
          tunnel: [w1165] -> w1160
          tunnel: w1158 -> [w1165]
          tunnel: [w1163] -> w1159
          frame #0 {
            n670 = Wait (ms)(milliseconds to wait=u32 100) -> ()  [unwired: 1 out]
          }
        }
        n671 = call "conversion data to bits.vi"("Data input"=w1134, "Max supply"=2.0) -> ("15 bits output"=w1132:u16)  [unwired: 1 in, 1 out]
        n672 = call "conversion data to bits.vi"("Data input"=w1133, "15 /16b"=TRUE, "Max supply"=150.0) -> ("15 bits output"=w1131:u16)  [unwired: 1 out]
        n673 = Number To Hexadecimal String(2:w1132) -> (0:w1125:string)  [unwired: 1 in]
        n674 = Number To Hexadecimal String(2:w1131) -> (0:w1123:string)  [unwired: 1 in]
        n675 = Concatenate Strings(w1125, ",1", ",", w1123) -> (w1122:string)
        n676 = Concatenate Strings("WF " ("string"), w1122) -> (w1121:string)
        n677 = VISA Write(VISA resource name=w1128, write buffer=w1121, error in (no error)=w1127) -> (VISA resource name out=w1157:refnum<visa-resource-name>, error out=w1158:errorcluster)  [unwired: 1 out]
        n678 = property class="Instr"(reference=w1159, error in=w1160) -> (reference out=w1156:refnum<visa-resource-name>, error out=w1154:errorcluster, "Serial Settings:Number of Bytes at Serial Port"=w1155:u32)
        n679 = VISA Read(VISA resource name=w1156, byte count=w1155, error in (no error)=w1154) -> (VISA resource name out=w1130:refnum<visa-resource-name>, error out=w1129:errorcluster)  [unwired: 2 out]
        n680 = local write "VISA ERROR"(w1129) -> ()
        n681 = local write "ORSAY"(w1130) -> ()
      }
      frame "TURN OFF WOBBLER" {
        n682 = flat-sequence {
          frame #0 {
            n683 = local read "APPEND"() -> (w1178:string)
            n684 = Concatenate Strings("WB 0" ("string"), w1178) -> (w1170:string)
            n685 = local read "VISA ERROR"() -> (w1179:errorcluster)
            n686 = local read "ORSAY"() -> (w1180:refnum<visa-resource-name>)
            n687 = VISA Write(VISA resource name=w1180, write buffer=w1170, error in (no error)=w1179) -> (VISA resource name out=w1174:refnum<visa-resource-name>, error out=w1173:errorcluster)  [unwired: 1 out]
            n688 = flat-sequence {
              tunnel: w1174 -> [w1183]
              tunnel: [w1185] -> w1171
              tunnel: w1173 -> [w1185]
              tunnel: [w1183] -> w1172
              frame #0 {
                n689 = Wait (ms)(milliseconds to wait=u32 100) -> ()  [unwired: 1 out]
              }
            }
            n690 = property class="Instr"(reference=w1172, error in=w1171) -> (reference out=w1175:refnum<visa-resource-name>, error out=w1177:errorcluster, "Serial Settings:Number of Bytes at Serial Port"=w1176:u32)
            n691 = VISA Read(VISA resource name=w1175, byte count=w1176, error in (no error)=w1177) -> (VISA resource name out=w1182:refnum<visa-resource-name>, error out=w1181:errorcluster)  [unwired: 2 out]
            n692 = local write "ORSAY"(w1182) -> ()
            n693 = local write "VISA ERROR"(w1181) -> ()
          }
          frame #1 {
          }
        }
      }
      frame "STOP SYSTEM" {
        n694 = flat-sequence {
          frame #0 {
            n695 = local read "VISA ERROR"() -> (w1189:errorcluster)
            n696 = local read "ORSAY"() -> (w1190:refnum<visa-resource-name>)
            n697 = VISA Close(VISA resource name=w1190, error in (no error)=w1189) -> ()  [unwired: 1 out]
          }
          frame #1 {
            n698 = Stop(stop? (T)=TRUE) -> ()
          }
        }
      }
      frame "MEASURE HV SUPPLY VOLTAGES" {
        w1208 = u16 4 items=["BEAM ENERGY", "EXTRACTOR", "SUPPRESSOR", "CONDENSOR", "OBJECTIVE"] ("HV SUPPLY")
        w1209 = u16 3 items=["BEAM ENERGY", "EXTRACTOR", "SUPPRESSOR", "CONDENSOR", "OBJECTIVE"] ("HV SUPPLY")
        w1212 = u16 2 items=["BEAM ENERGY", "EXTRACTOR", "SUPPRESSOR", "CONDENSOR", "OBJECTIVE"] ("HV SUPPLY")
        w1213 = u16 1 items=["BEAM ENERGY", "EXTRACTOR", "SUPPRESSOR", "CONDENSOR", "OBJECTIVE"] ("HV SUPPLY")
        w1214 = u16 0 items=["BEAM ENERGY", "EXTRACTOR", "SUPPRESSOR", "CONDENSOR", "OBJECTIVE"] ("HV SUPPLY")
        w1224 = "MEASURING ION GUN HV" ("PROCESS")
        n699 = local read "ORSAY"() -> (w1219:refnum<visa-resource-name>)
        n700 = local read "APPEND"() -> (w1204:string)
        n701 = call "READ HV SUPPLIES.vi"("ORSAY"=w1219, "HV SUPPLY"=w1214, "APPEND"=w1204) -> ("ORSAY 2"=w1216:refnum<visa-resource-name>, "VOLTAGE"=w1201:dbl[unit], "CURRENT"=→"BEAM CURRENT" →"CURRENT":dbl[unit], "ORSAY ERROR"=w1218:errorcluster)  [unwired: 9 in]
        "BEAM VOLTAGE" <- w1201
        "VOLTAGE" <- w1201
        n702 = call "READ HV SUPPLIES.vi"("ORSAY"=w1216, "HV SUPPLY"=w1213, "ORSAY ERROR"=w1218, "APPEND"=w1204) -> ("ORSAY 2"=w1215:refnum<visa-resource-name>, "VOLTAGE"=w1193:dbl[unit], "CURRENT"=→"EXTRACTOR  CURRENT" →"CURRENT":dbl[unit], "ORSAY ERROR"=w1217:errorcluster)  [unwired: 8 in]
        "EXTRACTOR" <- w1193
        "VOLTAGE" <- w1193
        n703 = call "READ HV SUPPLIES.vi"("ORSAY"=w1215, "HV SUPPLY"=w1212, "ORSAY ERROR"=w1217, "APPEND"=w1204) -> ("ORSAY 2"=w1211:refnum<visa-resource-name>, "VOLTAGE"=w1192:dbl[unit], "CURRENT"=→"SUPPRESSOR CURRENT" →"CURRENT":dbl[unit], "ORSAY ERROR"=w1205:errorcluster)  [unwired: 8 in]
        "SUPPRESSOR VOLTAGE" <- w1192
        "VOLTAGE" <- w1192
        n704 = local write "PROCESS"(w1224) -> ()
        n705 = Build Array (concatenate)(w1223, w1224) -> (w1222:string[])
        n706 = call "READ HV SUPPLIES.vi"("ORSAY"=w1211, "HV SUPPLY"=w1209, "ORSAY ERROR"=w1205, "APPEND"=w1204) -> ("ORSAY 2"=w1210:refnum<visa-resource-name>, "VOLTAGE"=→"CONDENSOR VOLTAGE":dbl[unit], "CURRENT"=→"CONDENSOR CURRENT":dbl[unit], "ORSAY ERROR"=w1206:errorcluster)  [unwired: 8 in]
        n707 = Bundle By Name(cluster=T24 {"BEAM"=0.0, "SUPPRESSOR"=0.0, "EXTRACTOR"=0.0} ("HIGH VOLTAGE SUPPLIES"), "BEAM"=w1201, "SUPPRESSOR"=w1192, "EXTRACTOR"=w1193) -> (→"HIGH VOLTAGE SUPPLIES":T24)
        n708 = local write "PROCESSES"(w1222) -> ()
        n709 = call "READ HV SUPPLIES.vi"("ORSAY"=w1210, "HV SUPPLY"=w1208, "ORSAY ERROR"=w1206, "APPEND"=w1204) -> ("ORSAY 2"=w1207:refnum<visa-resource-name>, "VOLTAGE"=→"OBJECTIVE VOLTAGE":dbl[unit], "CURRENT"=→"OBJECTIVE CURRENT":dbl[unit])  [unwired: 8 in, 1 out]
        n710 = local write "ORSAY"(w1207) -> ()
      }
      frame "SCANNING CONTROLS" {
        w1229 = "SCANNING CONTROL" ("PROCESS")
        n711 = Unbundle By Name("SCANNING CLUSTER") -> ("X-OFFSET"=w1255:sgl[unit], "Y-OFFSET"=w1254:sgl[unit], "ROTATION"=w1253:dbl[unit])  [unwired: 1 out]
        n712 = node(w1255) -> (w1251:sgl)
        n713 = node(w1254) -> (w1248:sgl)
        n714 = node(w1253) -> (w1247:dbl)
        n715 = local read "ORSAY"() -> (w1233:refnum<visa-resource-name>)
        n716 = call "conversion data to bits.vi"("Data input"=w1251, "Max supply"=sgl 30000.0) -> ("15 bits output"=w1246:u16)  [unwired: 1 in, 1 out]
        n717 = call "conversion data to bits.vi"("Data input"=w1248, "Max supply"=sgl 12000.0) -> ("15 bits output"=w1245:u16)  [unwired: 1 in, 1 out]
        n718 = call "conversion data to bits.vi"("Data input"=w1247, "Max supply"=sgl 2000.0) -> ("15 bits output"=w1244:u16)  [unwired: 1 in, 1 out]
        n719 = Number To Hexadecimal String(2:w1246) -> (0:w1243:string)  [unwired: 1 in]
        n720 = Number To Hexadecimal String(2:w1245) -> (0:w1240:string)  [unwired: 1 in]
        n721 = Number To Hexadecimal String(2:w1244) -> (0:w1239:string)  [unwired: 1 in]
        n722 = local read "APPEND"() -> (w1227:string)
        n723 = Concatenate Strings("XX  ", w1243, w1227) -> (w1238:string)
        n724 = Concatenate Strings("XX  ", w1240, w1227) -> (w1237:string)
        n725 = local write "PROCESS"(w1229) -> ()
        n726 = Concatenate Strings("XX ", w1239, w1227) -> (w1236:string)
        n727 = Build Array (concatenate)(w1230, w1229) -> (w1228:string[])
        n728 = Build Array(w1238, w1237, w1236) -> (w1232:string[])
        n729 = for {
          tunnel: w1232 -> [w1268] mode=indexing
          shift-right: [w1267] -> w1234
          shift-left: w1233 -> [w1269]
          shift-right: [w1257] -> w1225
          shift-left: w1231 -> [w1258]
          n730 = VISA Write(VISA resource name=w1269, write buffer=w1268) -> (VISA resource name out=w1264:refnum<visa-resource-name>, error out=w1263:errorcluster)  [unwired: 1 in, 1 out]
          n731 = flat-sequence {
            tunnel: w1264 -> [w1270]
            tunnel: [w1272] -> w1261
            tunnel: w1263 -> [w1272]
            tunnel: [w1270] -> w1262
            frame #0 {
              n732 = Wait (ms)(milliseconds to wait=u32 100) -> ()  [unwired: 1 out]
            }
          }
          n733 = property class="Instr"(reference=w1262, error in=w1261) -> (reference out=w1266:refnum<visa-resource-name>, error out=w1260:errorcluster, "Serial Settings:Number of Bytes at Serial Port"=w1265:u32)
          n734 = VISA Read(VISA resource name=w1266, byte count=w1265, error in (no error)=w1260) -> (VISA resource name out=w1267:refnum<visa-resource-name>, read buffer=w1259:string)  [unwired: 2 out]
          n735 = Build Array (concatenate)(w1258, w1259) -> (w1257:string[])
          n736 = local write "SERIAL \nRESPONSE"(w1257) -> ()
        }
        n737 = local write "PROCESSES"(w1228) -> ()
        n738 = local write "ORSAY"(w1234) -> ()
      }
      frame "SAVE SETTINGS" {
        n739 = stacked-sequence {
          seq-local: [w1280 _] -> [_ w1394]
          seq-local: [w1279 _] -> [_ w1393]
          frame #0 {
            w1314 = "FIB SETTINGS" ("channel name")
            n740 = local read "STIGMATOR"() -> (w1278:T16)
            n741 = local read "ION GUN SETTINGS"() -> (w1357:T2)
            n742 = local read "STIGMATOR X & Y"() -> (w1340:cluster{"X":sgl, "Y":sgl})
            n743 = local read "CONDENSOR"() -> (w1341:cluster{"COARSE":sgl[unit], "FINE":sgl[unit]})
            n744 = local read "OBJECTIVE"() -> (w1342:cluster{"COARSE":sgl[unit], "FINE":sgl[unit]})
            n745 = Unbundle By Name(w1278) -> ("STIG ALIGN"=w1277:cluster{"+X":sgl, "-X":sgl, "+Y":sgl, "-Y":sgl})
            n746 = local read "COLUMN VACUUM"() -> (w1283:dbl[unit])
            n747 = Unbundle By Name(w1357) -> ("BEAM ENERGY"=w1335:sgl[unit], "EXTRACTOR"=w1311:sgl[unit], "SUPPRESSOR"=w1310:sgl[unit], "ION CURRENT"=w1309:sgl[unit])
            n748 = Unbundle By Name(w1342) -> ("COARSE"=w1334:sgl[unit], "FINE"=w1327:sgl[unit])
            n749 = local read "BEAM CURRENT (FC1)"() -> (w1284:dbl[unit])
            n750 = Unbundle By Name(w1341) -> ("COARSE"=w1326:sgl[unit], "FINE"=w1325:sgl[unit])
            n751 = Unbundle By Name(w1340) -> ("X"=w1324:sgl, "Y"=w1323:sgl)
            n752 = Unbundle By Name(w1277) -> ("+X"=w1293:sgl, "-X"=w1292:sgl, "+Y"=w1291:sgl, "-Y"=w1290:sgl)
            n753 = To Variant(anything=w1293) -> (Variant=w1289:variant)
            n754 = To Variant(anything=w1292) -> (Variant=w1288:variant)
            n755 = To Variant(anything=w1291) -> (Variant=w1287:variant)
            n756 = To Variant(anything=w1290) -> (Variant=w1286:variant)
            n757 = call "File Dialog"() -> ("selected path"=w1359:path, "error out"=w1338:errorcluster)  [unwired: 12 in, 2 out]
            n758 = node(w1326) -> (w1303:sgl)
            n759 = node(w1325) -> (w1302:sgl)
            n760 = node(w1335) -> (w1312:sgl)
            n761 = node(w1311) -> (w1306:sgl)
            n762 = node(w1310) -> (w1307:sgl)
            n763 = node(w1309) -> (w1308:sgl)
            n764 = node(w1334) -> (w1305:sgl)
            n765 = node(w1327) -> (w1304:sgl)
            n766 = TDMS Open(8:w1338, 10:T26."create or replace" ("operation (0:open)"), 11:w1359) -> (0:w1337:errorcluster, 3:w1339:refnum<k34>)  [unwired: 4 in]
            n767 = To Variant(anything=w1312) -> (Variant=w1333:variant)
            n768 = To Variant(anything=w1306) -> (Variant=w1332:variant)
            n769 = To Variant(anything=w1307) -> (Variant=w1331:variant)
            n770 = node(w1284) -> (w1276:dbl)
            n771 = To Variant(anything=w1308) -> (Variant=w1330:variant)
            n772 = To Variant(anything=w1305) -> (Variant=w1329:variant)
            n773 = To Variant(anything=w1304) -> (Variant=w1322:variant)
            n774 = To Variant(anything=w1303) -> (Variant=w1321:variant)
            n775 = To Variant(anything=w1302) -> (Variant=w1320:variant)
            n776 = To Variant(anything=w1324) -> (Variant=w1319:variant)
            n777 = To Variant(anything=w1323) -> (Variant=w1318:variant)
            n778 = node(w1283) -> (w1282:dbl)
            n779 = To Variant(anything=w1276) -> (Variant=w1285:variant)
            n780 = To Variant(anything=w1282) -> (Variant=w1281:variant)
            n781 = Build Array(w1333, w1332, w1331, w1330, w1329, w1322, w1321, w1320, w1319, w1318, w1289, w1288, w1287, w1286, w1285, w1281) -> (w1328:variant[])
            n782 = for {
              tunnel: T25 ["BEAM ENERGY", "EXTRACTOR", "SUPRESSOR", "ION CURRENT", "OBJ COARSE", "OBJ FINE", "COND COARSE", "COND FINE", "STIGX", "STIGY", "STIG+X", "STIG-X", "STIG+Y", "STIG-Y", "PROBE CURRENT", "COLUMN VACUUM"] -> [w1375] mode=indexing
              shift-right: [w1377] -> w1313
              shift-left: w1337 -> [w1373]
              tunnel: w1328 -> [w1371] mode=indexing
              tunnel: w1314 -> [w1370]
              tunnel: "ORSAY COLUMN" -> [w1369]
              shift-right: [w1376] -> w1316
              shift-left: w1339 -> [w1378]
              n783 = call <userlib>:"Set Data Name__ogtk.vi"("error in (no error)"=w1373, "Data Name"=w1375, "Data"=w1371) -> ("error out"=w1372:errorcluster, "Renamed Data"=w1374:variant)  [unwired: 7 in]
              n784 = TDMS Set Properties(5:w1374, 7:w1375, 8:w1372, 9:w1369, 10:w1370, 11:w1378) -> (0:w1377:errorcluster, 3:w1376:refnum<k34>)  [unwired: 2 out]
            }
            n785 = local read "SCANNING CLUSTER"() -> (w1301:T18)
            n786 = Get Date/Time String() -> (date string=w1345:string, time string=w1346:string)  [unwired: 3 in]
            n787 = To Variant(anything=0) -> (Variant=w1347:variant)
            n788 = To Variant(anything="NAME") -> (Variant=w1350:variant)
            n789 = To Variant(anything="USER") -> (Variant=w1351:variant)
            n790 = To Variant(anything=w1345) -> (Variant=w1352:variant)
            n791 = To Variant(anything=w1346) -> (Variant=w1353:variant)
            n792 = To Variant(anything="COMMENT") -> (Variant=w1355:variant)
            n793 = Unbundle By Name(w1301) -> ("X-OFFSET"=w1297:sgl[unit], "Y-OFFSET"=w1296:sgl[unit], "ROTATION"=w1295:dbl[unit], "MAGNIFICATION"=w1294:dbl)  [unwired: 1 out]
            n794 = Build Array(w1347, w1350, w1351, w1352, w1353, w1355) -> (w1356:variant[])
            n795 = for {
              shift-right: [w1367] -> w1279
              shift-left: w1313 -> [w1365]
              tunnel: string[] ["RUN ID", "USER ID", "DATE", "TIME", "COMMENTS"] ("property names") -> [w1362] mode=indexing
              tunnel: "RUN DETAILS" ("channel name") -> [w1363]
              tunnel: w1356 -> [w1361] mode=indexing
              tunnel: w1314 -> [w1360]
              shift-right: [w1366] -> w1280
              shift-left: w1316 -> [w1368]
              n796 = call <userlib>:"Set Data Name__ogtk.vi"("Data Name"=w1362, "Data"=w1361) -> ("Renamed Data"=w1364:variant)  [unwired: 8 in, 1 out]
              n797 = TDMS Set Properties(5:w1364, 7:w1362, 8:w1365, 9:w1363, 10:w1360, 11:w1368) -> (0:w1367:errorcluster, 3:w1366:refnum<k34>)  [unwired: 2 out]
            }
            n798 = node(w1297) -> (w1300:sgl)
            n799 = node(w1296) -> (w1298:sgl)
            n800 = node(w1295) -> (w1299:dbl)
            n801 = To Variant(anything=w1300) -> ()  [unwired: 1 out]
            n802 = To Variant(anything=w1298) -> ()  [unwired: 1 out]
            n803 = To Variant(anything=w1299) -> ()  [unwired: 1 out]
            n804 = To Variant(anything=w1294) -> ()  [unwired: 1 out]
          }
          frame #1 {
            w1386 = "FIB SETTINGS" ("channel name")
            n805 = local read "OBJECT POSITIONS"() -> (w1385:T14)
            n806 = for {
              N: 7 -> [_]
              tunnel: "OBJECT POSITIONS:" ("channel name") -> [w1440]
              tunnel: w1386 -> [w1439]
              shift-right: [w1436] -> w1388
              shift-left: w1394 -> [w1438]
              shift-right: [w1435] -> w1387
              shift-left: w1393 -> [w1437]
              tunnel: w1385 -> [w1432] mode=indexing
              tunnel: "Xo" -> [w1431]
              tunnel: "Yo" -> [w1429]
              i -> [w1434]
              n807 = Unbundle By Name(w1432) -> ("POSITION.Xm"=w1424:dbl, "POSITION.Ym"=w1423:dbl)
              n808 = Number To Decimal String(number=w1434, width (-)=i16 0) -> (decimal integer string=w1430:string)
              n809 = Concatenate Strings(w1430, w1431) -> (w1428:string)
              n810 = Concatenate Strings(w1430, w1429) -> (w1427:string)
              n811 = Build Array(w1428, w1427) -> (w1426:string[])
              n812 = To Variant(anything=w1424) -> ()  [unwired: 1 out]
              n813 = To Variant(anything=w1423) -> ()  [unwired: 1 out]
              n814 = Build Array(w1424, w1423) -> (w1425:dbl[])
              n815 = for {
                shift-right: [w1448] -> w1435
                shift-left: w1437 -> [w1446]
                tunnel: w1426 -> [w1443] mode=indexing
                tunnel: w1440 -> [w1444]
                tunnel: w1439 -> [w1442]
                shift-right: [w1447] -> w1436
                shift-left: w1438 -> [w1449]
                tunnel: w1425 -> [w1441] mode=indexing
                n816 = call <userlib>:"Set Data Name__ogtk.vi"("Data Name"=w1443, "Data"=w1441) -> ("Renamed Data"=w1445:variant)  [unwired: 8 in, 1 out]
                n817 = TDMS Set Properties(5:w1445, 7:w1443, 8:w1446, 9:w1444, 10:w1442, 11:w1449) -> (0:w1448:errorcluster, 3:w1447:refnum<k34>)  [unwired: 2 out]
              }
            }
            n818 = local read "APERTURE POSITIONS"() -> (w1384:T14)
            n819 = for {
              N: 7 -> [_]
              tunnel: "APERTURE POSITIONS:" ("channel name") -> [w1413]
              tunnel: w1386 -> [w1412]
              shift-right: [w1409] -> w1382
              shift-left: w1388 -> [w1411]
              shift-right: [w1408] -> w1381
              shift-left: w1387 -> [w1410]
              tunnel: w1384 -> [w1405] mode=indexing
              tunnel: "Xm" -> [w1404]
              tunnel: "Ym" -> [w1402]
              i -> [w1407]
              n820 = Unbundle By Name(w1405) -> ("POSITION.Xm"=w1397:dbl, "POSITION.Ym"=w1396:dbl)
              n821 = Number To Decimal String(number=w1407, width (-)=i16 0) -> (decimal integer string=w1403:string)
              n822 = Concatenate Strings(w1403, w1404) -> (w1401:string)
              n823 = Concatenate Strings(w1403, w1402) -> (w1400:string)
              n824 = Build Array(w1401, w1400) -> (w1399:string[])
              n825 = To Variant(anything=w1397) -> ()  [unwired: 1 out]
              n826 = To Variant(anything=w1396) -> ()  [unwired: 1 out]
              n827 = Build Array(w1397, w1396) -> (w1398:dbl[])
              n828 = for {
                shift-right: [w1421] -> w1408
                shift-left: w1410 -> [w1419]
                tunnel: w1399 -> [w1416] mode=indexing
                tunnel: w1413 -> [w1417]
                tunnel: w1412 -> [w1415]
                shift-right: [w1420] -> w1409
                shift-left: w1411 -> [w1422]
                tunnel: w1398 -> [w1414] mode=indexing
                n829 = call <userlib>:"Set Data Name__ogtk.vi"("Data Name"=w1416, "Data"=w1414) -> ("Renamed Data"=w1418:variant)  [unwired: 8 in, 1 out]
                n830 = TDMS Set Properties(5:w1418, 7:w1416, 8:w1419, 9:w1417, 10:w1415, 11:w1422) -> (0:w1421:errorcluster, 3:w1420:refnum<k34>)  [unwired: 2 out]
              }
            }
            n831 = TDMS Close(8:w1381, 11:w1382) -> ()  [unwired: 2 out]
          }
        }
      }
      frame "READ SETTINGS" {
        (unwired) 2 ("index")
        (unwired) 1 ("index")
        w1497 = "FIB SETTINGS" ("group name")
        (unwired) string[] ["BEAM ENERGY", "EXTRACTOR", "SUPRESSOR", "ION CURRENT", "OBJ COARSE", "OBJ FINE", "COND COARSE", "COND FINE", "STIGX", "STIGY", "SCAN TYPE", "X-OFFSET", "Y-OFFSET", "ROTATION", "MAGNIFICATION", "STIG+X", "STIG-X", "STIG+Y", "STIG-Y", "PROBE CURRENT", "COLUMN VACUUM"]
        n832 = TDMS Open(11:"FIB SETUP FILE") -> (0:w1502:errorcluster, 3:w1501:refnum<k34>)  [unwired: 6 in]
        n833 = TDMS List Contents(4:w1502, 6:w1497, 7:w1501) -> (1:w1496:string[], 3:w1500:refnum<k34>)  [unwired: 2 out]
        n834 = Index Array(array=w1496, index=0) -> (element=w1494:string)
        n835 = TDMS Get Properties(9:w1494, 10:w1497, 11:w1500) -> (0:w1498:errorcluster, 3:w1499:refnum<k34>, 4:w1456:variant[])  [unwired: 3 in, 3 out]
        n836 = Delete From Array(array=w1456, length=1, index=0) -> (array with subset deleted=w1453:variant[])  [unwired: 1 out]
        n837 = for {
          tunnel: w1453 -> [w1506] mode=indexing
          tunnel: [w1505] -> w1491 mode=indexing
          n838 = Variant To Data(type=sgl 0.0, Variant=w1506) -> (data=w1505:sgl)  [unwired: 1 in, 1 out]
        }
        n839 = TDMS Close(8:w1498, 11:w1499) -> ()  [unwired: 2 out]
        n840 = Index Array(array=w1491, index #1=0 ("index"), index #2=1 ("index"), index #3=2 ("index"), index #4=3 ("index"), index #5=4 ("index"), index #6=5 ("index"), index #7=6 ("index"), index #8=7 ("index"), index #9=8 ("index"), index #10=9 ("index")) -> (element #1=w1490:sgl, element #2=w1489:sgl, element #3=w1488:sgl, element #4=w1487:sgl, element #5=w1474:sgl, element #6=w1473:sgl, element #7=w1472:sgl, element #8=w1471:sgl, element #9=w1458:sgl, element #10=w1457:sgl)  [unwired: 4 in, 4 out]
        n841 = node(w1490) -> (w1486:sgl[unit])
        n842 = node(w1489) -> (w1485:sgl[unit])
        n843 = node(w1488) -> (w1484:sgl[unit])
        n844 = node(w1487) -> (w1483:sgl[unit])
        n845 = node(w1474) -> (w1482:sgl[unit])
        n846 = node(w1473) -> (w1481:sgl[unit])
        n847 = node(w1472) -> (w1480:sgl[unit])
        n848 = node(w1471) -> (w1479:sgl[unit])
        n849 = local read "STIGMATOR X & Y"() -> (w1460:cluster{"X":sgl, "Y":sgl})
        n850 = local read "ION GUN SETTINGS"() -> (w1493:T2)
        n851 = Bundle By Name(cluster=w1493, "BEAM ENERGY"=w1486, "EXTRACTOR"=w1485, "SUPPRESSOR"=w1484, "ION CURRENT"=w1483) -> (w1492:T2)
        n852 = local read "CONDENSOR"() -> (w1477:cluster{"COARSE":sgl[unit], "FINE":sgl[unit]})
        n853 = Bundle By Name(cluster=w1477, "COARSE"=w1480, "FINE"=w1479) -> (w1476:cluster{"COARSE":sgl[unit], "FINE":sgl[unit]})
        n854 = local read "OBJECTIVE"() -> (w1478:cluster{"COARSE":sgl[unit], "FINE":sgl[unit]})
        n855 = Bundle By Name(cluster=w1478, "COARSE"=w1482, "FINE"=w1481) -> (w1475:cluster{"COARSE":sgl[unit], "FINE":sgl[unit]})
        n856 = Bundle By Name(cluster=w1460, "X"=w1458, "Y"=w1457) -> (w1459:cluster{"X":sgl, "Y":sgl})
        n857 = local write "STIGMATOR X & Y"(w1459) -> ()
        n858 = local write "OBJECTIVE"(w1475) -> ()
        n859 = local write "CONDENSOR"(w1476) -> ()
        n860 = local write "ION GUN SETTINGS"(w1492) -> ()
      }
      frame "BLANKING TOGGLE" {
        w1513 = "BLANKING MODE" ("PROCESS")
        n861 = local read "BEAM ON"() -> (w1514:bool)
        n862 = case shown="False" w1514 {
          tunnel: [w1516 w1538] -> w1511
          frame False {
            n863 = local read "APPEND"() -> (w1515:string)
            n864 = local read "VISA ERROR"() -> (w1527:errorcluster)
            n865 = Concatenate Strings("BL 0,1", "," ("string"), "0" ("string"), w1515) -> (w1517:string)
            n866 = local read "ORSAY"() -> (w1528:refnum<visa-resource-name>)
            n867 = VISA Write(VISA resource name=w1528, write buffer=w1517, error in (no error)=w1527) -> (VISA resource name out=w1524:refnum<visa-resource-name>, error out=w1522:errorcluster)  [unwired: 1 out]
            n868 = flat-sequence {
              tunnel: [w1534] -> w1523
              tunnel: w1524 -> [w1534]
              tunnel: [w1533] -> w1521
              tunnel: w1522 -> [w1533]
              frame #0 {
                n869 = Wait (ms)(milliseconds to wait=u32 100) -> ()  [unwired: 1 out]
              }
            }
            n870 = property class="Instr"(reference=w1523, error in=w1521) -> (reference out=w1531:refnum<visa-resource-name>, error out=w1529:errorcluster, "Serial Settings:Number of Bytes at Serial Port"=w1530:u32)
            n871 = VISA Read(VISA resource name=w1531, byte count=w1530, error in (no error)=w1529) -> (VISA resource name out=w1526:refnum<visa-resource-name>, read buffer=w1516:string, error out=w1525:errorcluster)  [unwired: 1 out]
            n872 = local write "VISA ERROR"(w1525) -> ()
            n873 = local write "ORSAY"(w1526) -> ()
          }
          frame True {
            n874 = local read "BLANKING CONTROL"() -> (w1539:u16)
            n875 = local read "APPEND"() -> (w1535:string)
            n876 = Pick Line(multi-line string="BL 0,0\nBL 1,1\nBL 2,0", line index=w1539) -> (output string=w1544:string)  [unwired: 1 in]
            n877 = Concatenate Strings(w1544, w1535) -> (w1537:string)
            n878 = local read "VISA ERROR"() -> (w1547:errorcluster)
            n879 = local read "ORSAY"() -> (w1548:refnum<visa-resource-name>)
            n880 = VISA Write(VISA resource name=w1548, write buffer=w1537, error in (no error)=w1547) -> (VISA resource name out=w1543:refnum<visa-resource-name>, error out=w1541:errorcluster)  [unwired: 1 out]
            n881 = flat-sequence {
              tunnel: [w1554] -> w1542
              tunnel: w1543 -> [w1554]
              tunnel: [w1553] -> w1540
              tunnel: w1541 -> [w1553]
              frame #0 {
                n882 = Wait (ms)(milliseconds to wait=u32 100) -> ()  [unwired: 1 out]
              }
            }
            n883 = property class="Instr"(reference=w1542, error in=w1540) -> (reference out=w1551:refnum<visa-resource-name>, error out=w1549:errorcluster, "Serial Settings:Number of Bytes at Serial Port"=w1550:u32)
            n884 = VISA Read(VISA resource name=w1551, byte count=w1550, error in (no error)=w1549) -> (VISA resource name out=w1546:refnum<visa-resource-name>, read buffer=w1538:string, error out=w1545:errorcluster)  [unwired: 1 out]
            n885 = local write "ORSAY"(w1546) -> ()
            n886 = local write "VISA ERROR"(w1545) -> ()
          }
        }
        n887 = Build Array (concatenate)(w1512, w1513) -> (w1509:string[])
        n888 = local write "PROCESS"(w1513) -> ()
        n889 = Build Array (concatenate)(w1510, w1511) -> (w1507:string[])
        n890 = local write "SERIAL \nRESPONSE"(w1507) -> ()
        n891 = local write "PROCESSES"(w1509) -> ()
      }
      frame "SET STIGMATOR" {
        w1558 = "ADJUSTING STIGMATOR" ("PROCESS")
        n892 = local read "VISA ERROR"() -> (w1564:errorcluster)
        n893 = local read "ORSAY"() -> (w1571:refnum<visa-resource-name>)
        n894 = call "CENTER STIGMATOR.vi"("STIGMATOR"="STIGMATOR") -> ("STIGMATOR COMMAND"=w1565:string)  [unwired: 5 in]
        n895 = VISA Write(VISA resource name=w1571, write buffer=w1565, error in (no error)=w1564) -> (VISA resource name out=w1566:refnum<visa-resource-name>, error out=w1568:errorcluster)  [unwired: 1 out]
        n896 = property class="Instr"(reference=w1566, error in=w1568) -> (reference out=w1567:refnum<visa-resource-name>, error out=w1569:errorcluster, "Serial Settings:Number of Bytes at Serial Port"=w1570:u32)
        n897 = local write "PROCESS"(w1558) -> ()
        n898 = Build Array (concatenate)(w1559, w1558) -> (w1557:string[])
        n899 = VISA Read(VISA resource name=w1567, byte count=w1570, error in (no error)=w1569) -> (VISA resource name out=w1563:refnum<visa-resource-name>, read buffer=w1561:string, error out=w1562:errorcluster)  [unwired: 1 out]
        n900 = local write "PROCESSES"(w1557) -> ()
        n901 = local write "ORSAY"(w1563) -> ()
        n902 = local write "VISA ERROR"(w1562) -> ()
        n903 = Build Array (concatenate)(w1560, w1561) -> (w1555:string[])
        n904 = local write "SERIAL \nRESPONSE"(w1555) -> ()
      }
      frame "SET WOBBLER FOR OBJECT" {
        n905 = local read "WOBBLER SETTINBGS FOR OBJECT ALIGNMENT"() -> (w1576:T11)
        n906 = Unbundle By Name(w1576) -> ()  [unwired: 2 out]
      }
      frame "STORE OBJECT POSITION" {
        n907 = flat-sequence {
          frame #0 {
            n908 = local read "OBJECT POSITIONS"() -> (w1587:T14)
            n909 = local read "OBJECT POSITION"() -> (w1582:T13)
            n910 = Unbundle By Name(w1582) -> ("Xo"=w1580:dbl, "Yo"=w1581:dbl)
            n911 = Index Array(array=w1587, index=0) -> (element=w1586:cluster{"POSITION":cluster{"Xm":dbl, "Ym":dbl}})
            n912 = local read "OBJECT APERTURE"() -> (w1588:u16)
            n913 = Bundle By Name(cluster=w1586, "POSITION.Xm"=w1580, "POSITION.Ym"=w1581) -> (w1585:cluster{"POSITION":cluster{"Xm":dbl, "Ym":dbl}})
            n914 = Replace Array Subset(array=w1587, new element=w1585, index=w1588) -> (w1584:T14)
            n915 = local write "OBJECT POSITIONS"(w1584) -> ()
          }
          frame #1 {
            n916 = local write "STORE OBJECT"(FALSE ("STORE OBJECT")) -> ()
          }
        }
      }
      frame "STORE APERTURE POSITION" {
        n917 = flat-sequence {
          frame #0 {
            n918 = local read "APERTURE POSITION"() -> (w1596:cluster{"Xm":dbl, "Ym":dbl})
            n919 = local read "APERTURE POSITIONS"() -> (w1601:T14)
            n920 = local read "APERTURE (MASS)"() -> (w1593:u16)
            n921 = Unbundle By Name(w1596) -> ("Xm"=w1594:dbl, "Ym"=w1595:dbl)
            n922 = Index Array(array=w1601, index=0) -> (element=w1600:cluster{"POSITION":cluster{"Xm":dbl, "Ym":dbl}})
            n923 = Bundle By Name(cluster=w1600, "POSITION.Xm"=w1594, "POSITION.Ym"=w1595) -> (w1599:cluster{"POSITION":cluster{"Xm":dbl, "Ym":dbl}})
            n924 = Replace Array Subset(array=w1601, new element=w1599, index=w1593) -> (w1598:T14)
            n925 = local write "APERTURE POSITIONS"(w1598) -> ()
          }
          frame #1 {
            n926 = local write "STORE APERTURE"(FALSE ("STORE OBJECT")) -> ()
          }
        }
      }
      frame "MOVE TO OBJECT" {
        n927 = local read "OBJECT POSITIONS"() -> (w1609:T14)
        n928 = local read "OBJECT APERTURE"() -> (w1603:u16)
        n929 = Index Array(array=w1609, index=w1603) -> (element=w1608:cluster{"POSITION":cluster{"Xm":dbl, "Ym":dbl}})
        n930 = Unbundle By Name(w1608) -> ("POSITION"=w1607:cluster{"Xm":dbl, "Ym":dbl})
        n931 = local write "SET OBJECT"(w1607) -> ()
      }
      frame "MOVE TO APERTURE" {
        n932 = local read "APERTURE (MASS)"() -> (w1610:u16)
        n933 = local read "APERTURE POSITIONS"() -> (w1615:T14)
        n934 = Index Array(array=w1615, index=w1610) -> (element=w1614:cluster{"POSITION":cluster{"Xm":dbl, "Ym":dbl}})
        n935 = Unbundle By Name(w1614) -> ("POSITION"=w1616:cluster{"Xm":dbl, "Ym":dbl})
        n936 = local write "SET APERTURE"(w1616) -> ()
      }
      frame "DEFINE NEW APERTURE" {
        n937 = local read "APERTURE POSITIONS"() -> (w1627:T14)
        n938 = local read "APERTURE POSITION"() -> (w1619:cluster{"Xm":dbl, "Ym":dbl})
        n939 = Unbundle By Name(w1619) -> ("Xm"=w1618:dbl, "Ym"=w1617:dbl)
        n940 = Index Array(array=w1627, index=0) -> (element=w1626:cluster{"POSITION":cluster{"Xm":dbl, "Ym":dbl}})
        n941 = Bundle By Name(cluster=w1626, "POSITION.Xm"=w1618, "POSITION.Ym"=w1617) -> (w1625:cluster{"POSITION":cluster{"Xm":dbl, "Ym":dbl}})
        n942 = local read "APERTURE (MASS)"() -> (w1628:u16)
        n943 = Replace Array Subset(array=w1627, new element=w1625, index=w1628) -> (w1624:T14)
        n944 = local write "APERTURE POSITIONS"(w1624) -> ()
      }
      frame "SHIFT OBJECT APERTURE" {
        n945 = flat-sequence {
          tunnel: [w1649] -> w1632
          tunnel: [w1648] -> w1631
          tunnel: [w1640] -> w1630
          tunnel: [w1638] -> w1629
          tunnel: w1632 -> [w1692]
          tunnel: w1631 -> [w1690]
          tunnel: w1630 -> [w1687]
          tunnel: w1629 -> [w1686]
          frame #0 {
            n946 = local read "OBJ APERTURE ALIGNMENT"() -> (w1649:T12)
            n947 = shared-variable "My Computer\\PI APERTURES.lvlib\\STAGE MAXIMUMS"() -> (w1645:T30)  [unwired: 1 in, 1 out]
            n948 = shared-variable "My Computer\\PI APERTURES.lvlib\\STAGE MINIMUMS"() -> (w1646:T31)  [unwired: 1 in, 1 out]
            n949 = local read "OBJECT POSITION"() -> (w1659:T13)
            n950 = Unbundle By Name(w1649) -> ("UP"=w1658:bool, "DOWN"=w1657:bool, "LEFT"=w1656:bool, "RIGHT"=w1655:bool, "STEP SIZE"=w1648:u16)
            n951 = Unbundle By Name(w1645) -> ("Xo MAX"=w1644:dbl, "Yo MAX"=w1642:dbl)
            n952 = Build Array(w1658, w1657, w1656, w1655) -> (w1654:bool[])
            n953 = Unbundle By Name(w1646) -> ("Xo MIN"=w1643:dbl, "Yo MIN"=w1641:dbl)
            n954 = case shown="7" w1648 {
              tunnel: [0.001 0.005 0.02 0.05 0.1 0.25 0.5 1.0] -> w1650
              frame 0 {
              }
              frame 1, Default {
              }
              frame 2 {
              }
              frame 3 {
              }
              frame 4 {
              }
              frame 5 {
              }
              frame 6 {
              }
              frame 7 {
              }
            }
            n955 = Unbundle By Name(w1659) -> ("Xo"=w1652:dbl, "Yo"=w1651:dbl)
            n956 = Boolean Array To Number(Boolean array=w1654) -> (number=w1653:u32)
            n957 = case shown="1" w1653 {
              tunnel: w1652 -> [w1669 w1673 w1677 w1681 w1685]
              tunnel: w1651 -> [w1668 w1672 w1676 w1678 w1683]
              tunnel: [w1669 w1673 w1677 w1680 w1684] -> w1647
              tunnel: [w1668 w1671 w1675 w1678 w1683] -> w1639
              tunnel: w1650 -> [_ w1670 w1674 w1679 w1682]
              frame 0, Default {
              }
              frame 1 {
                n958 = Add(x=w1672, y=w1670) -> (x+y=w1671:dbl)
              }
              frame 2 {
                n959 = Subtract(x=w1676, y=w1674) -> (x-y=w1675:dbl)
              }
              frame 4 {
                n960 = Subtract(x=w1681, y=w1679) -> (x-y=w1680:dbl)
              }
              frame 8 {
                n961 = Add(x=w1685, y=w1682) -> (x+y=w1684:dbl)
              }
            }
            n962 = In Range and Coerce(upper limit=w1644, x=w1647, lower limit=w1643) -> (coerced(x)=w1640:dbl)  [unwired: 1 out]
            n963 = In Range and Coerce(upper limit=w1642, x=w1639, lower limit=w1641) -> (coerced(x)=w1638:dbl)  [unwired: 1 out]
          }
          frame #1 {
            w1691 = FALSE ("UP")
            n964 = Bundle By Name(cluster=w1692, "UP"=w1691, "DOWN"=w1691, "LEFT"=w1691, "RIGHT"=w1691, "STEP SIZE"=w1690) -> (w1693:T12)
            n965 = local read "SET OBJECT"() -> (w1688:T13)
            n966 = Bundle By Name(cluster=w1688, "Xo"=w1687, "Yo"=w1686) -> (w1689:T13)
            n967 = local write "SET OBJECT"(w1689) -> ()
            n968 = local write "OBJ APERTURE ALIGNMENT"(w1693) -> ()
          }
        }
        n969 = Build Array (concatenate)(w1635, "SHIFT OBJECT APERTURE") -> (w1633:string[])
        n970 = local write "PROCESSES"(w1633) -> ()
      }
      frame "SHIFT MASS APERTURE" {
        n971 = flat-sequence {
          tunnel: [w1706] -> w1697
          tunnel: [w1705] -> w1696
          tunnel: [w1704] -> w1695
          tunnel: [w1703] -> w1694
          tunnel: w1697 -> [w1755]
          tunnel: w1696 -> [w1756]
          tunnel: w1695 -> [w1752]
          tunnel: w1694 -> [w1751]
          frame #0 {
            n972 = local read "MASS APERTURE ALIGNMENT"() -> (w1704:T12)
            n973 = shared-variable "My Computer\\PI APERTURES.lvlib\\STAGE MAXIMUMS"() -> (w1713:T30)  [unwired: 1 in, 1 out]
            n974 = shared-variable "My Computer\\PI APERTURES.lvlib\\STAGE MINIMUMS"() -> (w1714:T31)  [unwired: 1 in, 1 out]
            n975 = local read "APERTURE POSITION"() -> (w1715:cluster{"Xm":dbl, "Ym":dbl})
            n976 = Unbundle By Name(w1704) -> ("UP"=w1724:bool, "DOWN"=w1723:bool, "LEFT"=w1722:bool, "RIGHT"=w1721:bool, "STEP SIZE"=w1703:u16)
            n977 = Build Array(w1724, w1723, w1722, w1721) -> (w1720:bool[])
            n978 = case shown="0, Default" w1703 {
              tunnel: [0.001 0.005 0.02 0.05 0.1 0.25 0.5 1.0] -> w1716
              frame 0, Default {
              }
              frame 1 {
              }
              frame 2 {
              }
              frame 3 {
              }
              frame 4 {
              }
              frame 5 {
              }
              frame 6 {
              }
              frame 7 {
              }
            }
            n979 = Unbundle By Name(w1715) -> ("Xm"=w1718:dbl, "Ym"=w1717:dbl)
            n980 = Unbundle By Name(w1713) -> ("Xm MAX"=w1710:dbl, "Ym MAX"=w1708:dbl)
            n981 = Unbundle By Name(w1714) -> ("Xm MIN"=w1709:dbl, "Ym MIN"=w1707:dbl)
            n982 = Boolean Array To Number(Boolean array=w1720) -> (number=w1719:u32)
            n983 = case shown="8" w1719 {
              tunnel: w1718 -> [w1734 w1738 w1742 w1746 w1750]
              tunnel: w1717 -> [w1733 w1737 w1741 w1743 w1748]
              tunnel: [w1734 w1738 w1742 w1745 w1749] -> w1712
              tunnel: [w1733 w1736 w1740 w1743 w1748] -> w1711
              tunnel: w1716 -> [_ w1735 w1739 w1744 w1747]
              frame 0, Default {
              }
              frame 1 {
                n984 = Add(x=w1737, y=w1735) -> (x+y=w1736:dbl)
              }
              frame 2 {
                n985 = Subtract(x=w1741, y=w1739) -> (x-y=w1740:dbl)
              }
              frame 4 {
                n986 = Subtract(x=w1746, y=w1744) -> (x-y=w1745:dbl)
              }
              frame 8 {
                n987 = Add(x=w1750, y=w1747) -> (x+y=w1749:dbl)
              }
            }
            n988 = In Range and Coerce(upper limit=w1710, x=w1712, lower limit=w1709) -> (coerced(x)=w1705:dbl)  [unwired: 1 out]
            n989 = In Range and Coerce(upper limit=w1708, x=w1711, lower limit=w1707) -> (coerced(x)=w1706:dbl)  [unwired: 1 out]
          }
          frame #1 {
            w1754 = FALSE ("UP")
            n990 = local read "SET APERTURE"() -> (w1757:T15)
            n991 = Bundle By Name(cluster=w1757, "Xm"=w1756, "Ym"=w1755) -> (w1758:T15)
            n992 = Bundle By Name(cluster=w1752, "UP"=w1754, "DOWN"=w1754, "LEFT"=w1754, "RIGHT"=w1754, "STEP SIZE"=w1751) -> (w1753:T12)
            n993 = local write "SET APERTURE"(w1758) -> ()
            n994 = local write "MASS APERTURE ALIGNMENT"(w1753) -> ()
          }
        }
        n995 = Build Array (concatenate)(w1700, "SHIFT APERTURE") -> (w1698:string[])
        n996 = local write "PROCESSES"(w1698) -> ()
      }
    }
  }
  n997 = while {
    shift-right: [w1760] -> _
    shift-left: w11 -> [w1762]
    stop <- TRUE continue-if-true
    n998 = Dequeue Element(queue=w1762) -> (queue out=w1760:refnum<queue>, element=w1761:enum16{"INIT DAQ", "STOP TASKS"})  [unwired: 2 in, 2 out]
    n999 = case shown="\"STOP TASKS\"" w1761 {
      frame "INIT DAQ", Default {
      }
      frame "STOP TASKS" {
      }
    }
  }
  n1000 = while {
    shift-right: [w1764] -> _
    shift-left: w23 -> [w1767]
    stop <- w1765 stop-if-true
    n1001 = Dequeue Element(queue=w1767) -> (queue out=w1764:refnum<queue>, element=w1766:T20)  [unwired: 2 in, 2 out]
    n1002 = case shown="True" "ENABLE CAMERA" {
      tunnel: w1766 -> [_ w1768]
      frame False {
      }
      frame True {
        n1003 = case shown="\"INIT VIDEO\"" w1768 {
          frame "LOOP", Default {
            n1004 = local read "FIB SAMPLE CAMERA"() -> (w1770:T5)
            n1005 = local read "FIB CAMERA ERROR"() -> (w1771:errorcluster)
            n1006 = local read "FIB CAMERA"() -> (w1772:T6)
            n1007 = property on="ANGLE" class="DigNum (strict)"("Visible"="ROTATE VIEW") -> ()  [unwired: 2 in, 2 out]
            n1008 = call <vilib>:"IMAQdx Get Image2.vi"("Timeout (ms)"=500, "Buffer Number Mode (Next)"=IMAQdx_Buffer_Number_Mode."Last New", "error in"=w1771, "Image In"=w1772, "Session In"=w1770) -> ("error out"=w1782:errorcluster, "Image Out"=w1783:T6)  [unwired: 3 in, 2 out]
            n1009 = case shown="True" "ROTATE VIEW" {
              tunnel: w1783 -> [w1797 w1801]
              tunnel: w1782 -> [w1796 w1800]
              tunnel: [w1796 w1799] -> w1777
              tunnel: [w1797 w1798] -> w1778
              frame False {
              }
              frame True {
                n1010 = call "IMAQ Rotate"("error in (no error)"=w1800, "Angle (degrees)"="ANGLE", "Image Src"=w1801) -> ("error out"=w1799:errorcluster, "Image Dst Out"=w1798:T6)  [unwired: 7 in]
              }
            }
            n1011 = case shown="False" "SYMMETRY" {
              tunnel: w1778 -> [w1804 w1809]
              tunnel: w1777 -> [w1803 w1808]
              tunnel: "IMAGE SYMMETRY" -> [_ w1807]
              tunnel: [w1804 w1806] -> w1784
              tunnel: [w1803 w1805] -> w1785
              frame False {
              }
              frame True {
                n1012 = call "IMAQ Symmetry"("error in (no error)"=w1808, "Type of Symmetry"=w1807, "Image Src"=w1809) -> ("error out"=w1805:errorcluster, "Image Dst Out"=w1806:T6)  [unwired: 2 in]
              }
            }
            n1013 = property on="BRIGHT,CONT,GAMMA" class="Clust (strict)"("Visible"="REFLECTIVITY") -> ()  [unwired: 2 in, 2 out]
            n1014 = case shown="True" "REFLECTIVITY" {
              tunnel: w1784 -> [w1787 w1791]
              tunnel: [w1787 w1793] -> w1769
              tunnel: "BRIGHT,CONT,GAMMA" -> [_ w1792]
              tunnel: w1785 -> [w1786 w1790]
              tunnel: [w1786 w1788] -> _
              frame False {
              }
              frame True {
                w1795 = T34 0 items=["Grayscale (U8)", "Grayscale (I16)", "Grayscale (SGL)", "Complex (CSG)", "RGB (U32)", "HSL (U32)", "RGB (U64)", "Grayscale (U16)"] ("Image Type")
                n1015 = call "IMAQ Cast Image"("Image Type"=w1795, "error in (no error)"=w1790, "Image Src"=w1791) -> ("error out"=w1789:errorcluster, "Image Dst Out"=w1794:T6)  [unwired: 7 in]
                n1016 = call "IMAQ BCGLookup"("Image Src"=w1794, "BCG Values"=w1792, "error in (no error)"=w1789) -> ("Image Dst Out"=w1793:T6, "error out"=w1788:errorcluster)  [unwired: 4 in]
              }
            }
            n1017 = local write "FIB CAMERA"(w1769) -> ()
          }
          frame "INIT VIDEO" {
            w1816 = T34 4 items=["Grayscale (U8)", "Grayscale (I16)", "Grayscale (SGL)", "Complex (CSG)", "RGB (U32)", "HSL (U32)", "RGB (U64)", "Grayscale (U16)"] ("Image Type")
            w1819 = 2.0
            w1847 = 2.0
            w1846 = sgl 0.95 ("x")
            n1018 = call <vilib>:"IMAQdx Open Camera.vi"("Camera Control Mode"=IMAQdx_Camera_Control_Mode."Controller", "Session In"=T5 "MAKO") -> ("error out"=w1844:errorcluster, "Session Out"=w1845:T5)  [unwired: 8 in]
            n1019 = call <vilib>:"IMAQdx Enumerate Attributes.vi"("error in"=w1844, "Session In"=w1845) -> ("error out"=w1840:errorcluster, "Session Out"=w1841:T5)  [unwired: 7 in, 1 out]
            n1020 = property class="IMAQdx"(reference=w1841, error in=w1840) -> (reference out=w1839:T5, error out=w1838:errorcluster, "ActualPeakBandwidth"=→"ActualPeakBandwidth":dbl)
            n1021 = property class="IMAQdx"(reference=w1839, error in=w1838) -> (reference out=w1813:T5, error out=w1812:errorcluster, "IPAddress"=→"IP ADDRESS":string, "Width"=w1811:u32, "Height"=w1810:u32)
            "IMAGE XPIXELS" <- w1811
            "IMAGE YPIXELS" <- w1810
            n1022 = Multiply(x=w1811, y=w1846) -> (x*y=w1850:sgl)
            n1023 = Multiply(x=w1810, y=w1846) -> (x*y=w1849:sgl)
            n1024 = To Double Precision Float(number=w1811) -> (double precision float=w1852:dbl)
            n1025 = To Double Precision Float(number=w1810) -> (double precision float=w1853:dbl)
            n1026 = Bundle(w1850, w1849) -> ()  [unwired: 1 in, 1 out]
            n1027 = Divide(x=w1853, y=w1847) -> (x/y=→"IMAGE YCENTRE":dbl)
            n1028 = Divide(x=w1852, y=w1847) -> (x/y=→"IMAGE XCENTRE":dbl)
            n1029 = call <vilib>:"IMAQdx Configure Grab.vi"("error in"=w1812, "Session In"=w1813) -> ("error out"=w1826:errorcluster, "Session Out"=w1827:T5)  [unwired: 8 in]
            n1030 = case shown="False" FALSE {
              tunnel: w1827 -> [w1857 w1861]
              tunnel: [w1857 w1860] -> w1836
              tunnel: w1826 -> [w1856 w1859]
              tunnel: [w1856 w1858] -> w1837
              frame False {
              }
              frame True {
                n1031 = call <vilib>:"IMAQdx Read Attributes.vi"("error in"=w1859, "Session In"=w1861) -> ("error out"=w1858:errorcluster, "Session Out"=w1860:T5)  [unwired: 8 in]
              }
            }
            n1032 = Divide(x=w1811, y=w1819) -> (x/y=w1828:dbl)
            n1033 = Divide(x=w1810, y=w1819) -> (x/y=w1829:dbl)
            n1034 = To Long Integer(number=w1828) -> (32bit integer=w1830:i32)
            n1035 = To Long Integer(number=w1829) -> (32bit integer=w1831:i32)
            n1036 = Subtract(x=w1830, y=3) -> (x-y=w1833:i32)
            n1037 = call <vilib>:"IMAQdx Start Acquisition.vi"("error in"=w1837, "Session In"=w1836) -> ("error out"=→"FIB CAMERA ERROR":errorcluster, "Session Out"=→"FIB SAMPLE CAMERA":T5)  [unwired: 8 in]
            n1038 = Subtract(x=w1831, y=2) -> (x-y=w1832:i32)
            n1039 = call "IMAQ Create"("Image Name"="TARGET", "Image Type"=w1816, "error in (no error)"=w1837) -> ("New Image"=w1824:T6, "error out"=w1835:errorcluster)  [unwired: 2 in]
            n1040 = Bundle(w1833, w1832) -> (w1834:cluster{i32, i32})  [unwired: 1 in]
            "CENTRE CAMERA FOV" <- w1834
            n1041 = call "IMAQ Overlay Bitmap"("Group"="FEATURES", "error in (no error)"=w1835, "Bitmap"=u32[][] [[16777216, 16777216, 16777216, 16777216, 16777216, 16777216, 16777216, 16777216, 16777216, 16777216, 16777216, 12189440, 16777216, 16777216, 16777216, 16777216, 16777216, 16777216, 16777216, 16777216, 16777216, 16777216, 16777216], [16777216, 16777216, 16777216, 16777216, 16777216, 16777216, 16777216, 16777216, 16777216, 16777216, 16777216, 12189440, 16777216, 16777216, 16777216, 16777216, 16777216, 16777216, 16777216, 16777216, 16777216, 16777216, 16777216], [16777216, 16777216, 16777216, 16777216, 16777216, 16777216, 16777216, 16777216, 16777216, 16777216, 15859456, 12189440, 15859456, 16777216, 16777216, 16777216, 16777216, 16777216, 16777216, 16777216, 16777216, 16777216, 16777216], [16777216, 16777216, 16777216, 16777216, 16777216, 16777216, 16777216, 16777216, 16777216, 16777216, 15859456, 12189440, 15859456, 16777216, 16777216, 16777216, 16777216, 16777216, 16777216, 16777216, 16777216, 16777216, 16777216], [16777216, 16777216, 16777216, 16777216, 16777216, 16777216, 16777216, 16777216, 16777216, 16777216, 15859456, 12189440, 15859456, 16777216, 16777216, 16777216, 16777216, 16777216, 16777216, 16777216, 16777216, 16777216, 16777216], [16777216, 16777216, 16777216, 16777216, 16777216, 16777216, 16777216, 16777216, 16777216, 16777216, 15859456, 12189440, 15859456, 16777216, 16777216, 16777216, 16777216, 16777216, 16777216, 16777216, 16777216, 16777216, 16777216], [16777216, 16777216, 16777216, 16777216, 16777216, 16777216, 16777216, 16777216, 16777216, 16777216, 15859456, 12189440, 15859456, 16777216, 16777216, 16777216, 16777216, 16777216, 16777216, 16777216, 16777216, 16777216, 16777216], [16777216, 16777216, 16777216, 16777216, 16777216, 16777216, 16777216, 16777216, 16777216, 16777216, 16777216, 12189440, 16777216, 16777216, 16777216, 16777216, 16777216, 16777216, 16777216, 16777216, 16777216, 16777216, 16777216], [16777216, 16777216, 16777216, 16777216, 16777216, 16777216, 16777216, 16777216, 12189440, 16777216, 16777216, 12189440, 16777216, 16777216, 12189440, 16777216, 16777216, 16777216, 16777216, 16777216, 16777216, 16777216, 16777216], [16777216, 16777216, 16777216, 16777216, 16777216, 16777216, 16777216, 16777216, 16777216, 12189440, 16777216, 12189440, 16777216, 12189440, 16777216, 16777216, 16777216, 16777216, 16777216, 16777216, 16777216, 16777216, 16777216], [16777216, 16777216, 15859456, 15859456, 15859456, 15859456, 15859456, 16777216, 16777216, 16777216, 16777216, 12189440, 16777216, 16777216, 16777216, 16777216, 15859456, 15859456, 15859456, 15859456, 15859456, 16777216, 16777216], [12189440, 12189440, 12189440, 12189440, 12189440, 12189440, 12189440, 12189440, 12189440, 12189440, 12189440, 12189440, 12189440, 12189440, 12189440, 12189440, 12189440, 12189440, 12189440, 12189440, 12189440, 12189440, 12189440], [16777216, 16777216, 15859456, 15859456, 15859456, 15859456, 15859456, 16777216, 16777216, 16777216, 16777216, 12189440, 16777216, 16777216, 16777216, 16777216, 15859456, 15859456, 15859456, 15859456, 15859456, 16777216, 16777216], [16777216, 16777216, 16777216, 16777216, 16777216, 16777216, 16777216, 16777216, 16777216, 12189440, 16777216, 12189440, 16777216, 12189440, 16777216, 16777216, 16777216, 16777216, 16777216, 16777216, 16777216, 16777216, 16777216], [16777216, 16777216, 16777216, 16777216, 16777216, 16777216, 16777216, 16777216, 12189440, 16777216, 16777216, 12189440, 16777216, 16777216, 12189440, 16777216, 16777216, 16777216, 16777216, 16777216, 16777216, 16777216, 16777216], [16777216, 16777216, 16777216, 16777216, 16777216, 16777216, 16777216, 16777216, 16777216, 16777216, 16777216, 12189440, 16777216, 16777216, 16777216, 16777216, 16777216, 16777216, 16777216, 16777216, 16777216, 16777216, 16777216], [16777216, 16777216, 16777216, 16777216, 16777216, 16777216, 16777216, 16777216, 16777216, 16777216, 15859456, 12189440, 15859456, 16777216, 16777216, 16777216, 16777216, 16777216, 16777216, 16777216, 16777216, 16777216, 16777216], [16777216, 16777216, 16777216, 16777216, 16777216, 16777216, 16777216, 16777216, 16777216, 16777216, 15859456, 12189440, 15859456, 16777216, 16777216, 16777216, 16777216, 16777216, 16777216, 16777216, 16777216, 16777216, 16777216], [16777216, 16777216, 16777216, 16777216, 16777216, 16777216, 16777216, 16777216, 16777216, 16777216, 15859456, 12189440, 15859456, 16777216, 16777216, 16777216, 16777216, 16777216, 16777216, 16777216, 16777216, 16777216, 16777216], [16777216, 16777216, 16777216, 16777216, 16777216, 16777216, 16777216, 16777216, 16777216, 16777216, 15859456, 12189440, 15859456, 16777216, 16777216, 16777216, 16777216, 16777216, 16777216, 16777216, 16777216, 16777216, 16777216], [16777216, 16777216, 16777216, 16777216, 16777216, 16777216, 16777216, 16777216, 16777216, 16777216, 15859456, 12189440, 15859456, 16777216, 16777216, 16777216, 16777216, 16777216, 16777216, 16777216, 16777216, 16777216, 16777216], [16777216, 16777216, 16777216, 16777216, 16777216, 16777216, 16777216, 16777216, 16777216, 16777216, 16777216, 12189440, 16777216, 16777216, 16777216, 16777216, 16777216, 16777216, 16777216, 16777216, 16777216, 16777216, 16777216], [16777216, 16777216, 16777216, 16777216, 16777216, 16777216, 16777216, 16777216, 16777216, 16777216, 16777216, 12189440, 16777216, 16777216, 16777216, 16777216, 16777216, 16777216, 16777216, 16777216, 16777216, 16777216, 16777216]], "Top Left Point"=w1834, "Image"=w1824) -> ("Image Out"=w1825:T6)  [unwired: 5 in, 1 out]
            n1042 = local write "FIB CAMERA"(w1825) -> ()
          }
          frame "CAMERA GAIN" {
            n1043 = local read "FIB SAMPLE CAMERA"() -> (w1864:T5)
            n1044 = local read "FIB CAMERA ERROR"() -> (w1863:errorcluster)
            n1045 = property class="IMAQdx"(reference=w1864, error in=w1863, "ActiveAttribute"="GainAuto") -> (reference out=w1871:T5, error out=w1872:errorcluster)
            n1046 = property class="IMAQdx"(reference=w1871, error in=w1872, "ValueU32"="GAIN METHOD") -> (reference out=w1873:T5, error out=w1874:errorcluster)
            n1047 = property class="IMAQdx"(reference=w1873, error in=w1874, "ActiveAttribute"="GainRaw") -> (reference out=w1868:T5, error out=w1869:errorcluster)
            n1048 = property class="IMAQdx"(reference=w1868, error in=w1869, "ValueDBL"="GAIN") -> (reference out=w1865:T5, error out=w1862:errorcluster)
            n1049 = local write "FIB SAMPLE CAMERA"(w1865) -> ()
            n1050 = local write "FIB CAMERA ERROR"(w1862) -> ()
          }
          frame "CAMERA EXPOSURE" {
            n1051 = local read "FIB SAMPLE CAMERA"() -> (w1879:T5)
            n1052 = local read "FIB CAMERA ERROR"() -> (w1878:errorcluster)
            n1053 = property class="IMAQdx"(reference=w1879, error in=w1878, "ActiveAttribute"="ExposureAuto") -> (reference out=w1883:T5, error out=w1882:errorcluster)
            n1054 = property class="IMAQdx"(reference=w1883, error in=w1882, "ValueU32"=u32 1) -> (reference out=w1892:T5, error out=w1893:errorcluster)
            n1055 = case shown="0, Default" "CONFIGS" {
              tunnel: [w1908 20.0 ("EXPOSURE TIME") 5.0 ("EXPOSURE TIME")] -> w1891
              tunnel: "EXPOSURE" -> [w1908 _ _]
              frame 0, Default {
              }
              frame 1 {
              }
              frame 2 {
              }
            }
            n1056 = local write "EXPOSURE"(w1891) -> ()
            n1057 = Multiply(x=1000.0, y=w1891) -> (x*y=w1894:dbl)
            n1058 = case shown="True" TRUE {
              tunnel: w1892 -> [w1899 w1906]
              tunnel: w1893 -> [w1898 w1905]
              tunnel: w1894 -> [_ w1902]
              tunnel: [w1899 w1901] -> w1881
              tunnel: [w1898 w1900] -> w1880
              frame False {
              }
              frame True {
                n1059 = property class="IMAQdx"(reference=w1906, error in=w1905, "ActiveAttribute"="ExposureTimeAbs") -> (reference out=w1904:T5, error out=w1903:errorcluster)
                n1060 = property class="IMAQdx"(reference=w1904, error in=w1903, "ValueDBL"=w1902) -> (reference out=w1901:T5, error out=w1900:errorcluster)
              }
            }
            n1061 = property class="IMAQdx"(reference=w1881, error in=w1880, "ActiveAttribute"="GainAuto") -> (reference out=w1895:T5, error out=w1896:errorcluster)
            n1062 = property class="IMAQdx"(reference=w1895, error in=w1896, "ValueU32"=u32 2) -> (reference out=w1877:T5, error out=w1876:errorcluster)
            n1063 = local write "FIB SAMPLE CAMERA"(w1877) -> ()
            n1064 = local write "FIB CAMERA ERROR"(w1876) -> ()
          }
        }
      }
    }
    n1065 = local read "STOP"() -> (w1765:bool)
  }
  n1066 = case shown="True" FALSE {
    frame False {
    }
    frame True {
      n1067 = call "MNL.vi"() -> ()  [unwired: 5 in, 15 out]
      n1068 = call "MPL.vi"() -> ()  [unwired: 5 in, 15 out]
      n1069 = call "VEL.vi"() -> ()  [unwired: 6 in, 14 out]
      n1070 = call "VEL?.vi"() -> ()  [unwired: 5 in, 15 out]
      n1071 = call "TMN?.vi"() -> ()  [unwired: 5 in, 15 out]
      n1072 = call "LIM?.vi"() -> ()  [unwired: 5 in, 15 out]
      n1073 = call "GOH.vi"() -> ()  [unwired: 5 in, 15 out]
      n1074 = call "TMX?.vi"() -> ()  [unwired: 5 in, 15 out]
    }
  }
